vi "Position_TOTAL_R23.vi"(5 "Distance Between \nCameras  (*unit)":sgl=2.3) -> (12 "dX, dY\nLeft Cam":cluster{"X":sgl[], "Y":sgl[]}={"X"=[-1.0065897, 0.099401906, 1.1628555, 2.2500029, 0.0], "Y"=[10.716516, 10.801518, 10.883252, 10.9668045, 0.0]}, 13 "Position Valid":bool=TRUE, 14 "Left Camera Real Coordinates":cluster{"X":sgl, "Y":sgl}={"X"=10.842023, "Y"=1.3735824}, 16 "dX, dY\nRight Cam":cluster{"X":sgl[], "Y":sgl[]}={"X"=[-2.8840373, -1.7780458, -0.7145921, 0.3725553, -1.8774476], "Y"=[9.387911, 9.472914, 9.554648, 9.638201, -1.3286046]}, 18 "Robot Coordinates":cluster{"X":sgl, "Y":sgl}={"X"=10.17772, "Y"=2.3123062}, 19 "Orietnation\n(current)":sgl=-30.94054 format="%#_13g")   [LabVIEW 2015]
uses:
  <vilib>/Analysis/coordinate.llb/2D Cartesian Coordinate Rotation (Array).vi
  <vilib>/myRIO/Common/Instrument Driver Framework/myRIO v1.0/DIO/vis/myRIO v1.0 Close DIO.vi
  <vilib>/myRIO/Common/Instrument Driver Framework/myRIO v1.0/DIO/vis/myRIO v1.0 Unreserve DIO.vi
  <vilib>/myRIO/Common/Instrument Driver Framework/myRIO v1.0/DIO/vis/myRIO v1.0 Build MUX Configuration DIO.vi
  <vilib>/myRIO/Common/Instrument Driver Framework/myRIO v1.0/Resource Manager/vis/myRIO v1.0 Unreserve Channel List.vi
  <vilib>/myRIO/Common/Instrument Driver Framework/myRIO v1.0/Resource Manager/vis/myRIO v1.0 Create Configuration List.vi
  <vilib>/myRIO/Common/Instrument Driver Framework/myRIO v1.0/Resource Manager/vis/myRIO v1.0 Unreserve Channel.vi
  <vilib>/myRIO/Common/Instrument Driver Framework/myRIO v1.0/Resource Manager/vis/myRIO v1.0 Build Mutex Name.vi
  <vilib>/Instr/_visa.llb/VISA Configure Serial Port (Instr).vi
  <vilib>/myRIO/Common/Instrument Driver Framework/myRIO v1.0/DIO/vis/myRIO v1.0 Shutdown DIO.vi
  <vilib>/Utility/error.llb/Error Cluster From Error Code.vi
  <vilib>/myRIO/Common/Instrument Driver Framework/myRIO v1.0/Resource Manager/vis/myRIO v1.0 Configure IO.vi
  <vilib>/myRIO/Common/Instrument Driver Framework/Utilities/vis/Configuration Manager.vi
  <vilib>/myRIO/Common/Instrument Driver Framework/Utilities/vis/IO Manager.vi
  <vilib>/myRIO/Common/Instrument Driver Framework/myRIO v1.0/myRIO v1.0 Close.vi
  <vilib>/Analysis/NI_AALPro.lvlib
  <vilib>/myRIO/Instrument Drivers/Onboard IO/DIO/DIO.lvlib
panel:
  in  "New Orientation\nWeight":sgl=0.2
  out "Array 3":sgl[](array[numeric])=[3.2039287, 3.9103284, 4.8311996, 5.9665127, 6.4357905]
  out "Array 2":sgl[](array[numeric])=[5.5039287, 6.210328, 7.1312, 8.266513, 8.73579]
  out "Array":sgl[](array[numeric])=[9.555056, 8.575206, 8.036942, 7.810829, 6.6351933]
  in  "New Position\nWeight (Y coord)":sgl=0.3 format="%#_13g"
  out "Scale Based\nWeight":sgl=1.0 format="%#_13g"
  in  "Triangle Based\nWeight":sgl format="%#_13g"
  out "Current Cam State - R":T1(ring)=enum."Normal - 5"
  out "Current Cam State - L":T1(ring)=enum."Normal - 5"
  out "Valid Beacon Sets_":bool[](array[boolean])=[TRUE, TRUE, TRUE, TRUE, TRUE]
  in  "Distance Threshold\nRef Triangles (*unit)":sgl=30.0
  out "dA2 4":sgl=48.543114 format="%#_13g"
  out "dA2 2":sgl=48.543114 format="%#_13g"
  out "dA2 3":sgl=44.126 format="%#_13g"
  out "Beacon Scales - Left":sgl[](array[numeric])=[46.59789, 48.180458, 47.842606, 46.504417, 45.297752]
  out "Beacon Scales - Right":sgl[](array[numeric])=[50.81787, 54.150085, 54.01553, 51.723366, 54.605507]
  in  "New Orientation \nThreshold":sgl=20.0
  in  "Moving Average\nWindow Length":u8=10
  out "Current Recovery State -L":enum16{"Generic Sweep", "Recovery Search"}(ring)=enum."Recovery Search"
  out "Current Move Delta - L 2":u16
  out "Next Recovery State - Left":enum16{"Generic Sweep", "Recovery Search"}(ring)=enum."Recovery Search"
  out "Next Recovery State - Right":enum16{"Generic Sweep", "Recovery Search"}(ring)=enum."Recovery Search"
  out "Current Recovery State - Right":enum16{"Generic Sweep", "Recovery Search"}(ring)=enum."Recovery Search"
  in  "Initial Recovery State  - Right":enum16{"Generic Sweep", "Recovery Search"}(ring)=enum."Recovery Search"
  in  "Initial Recovery State - L":enum16{"Generic Sweep", "Recovery Search"}(ring)=enum."Recovery Search"
  out "Next Tracking State - Right":enum16{"Track", "Reactive Predict", ""}(ring)
  out "Current Tracking State - Right 2":enum16{"Track", "Reactive Predict", ""}(ring)
  in  "Initial Tracking State - Right":enum16{"Track", "Reactive Predict", ""}(ring)
  out "Last Track Angle - R":sgl=59.941406
  out "Next Tracking State - Left":enum16{"Track", "Reactive Predict", ""}(ring)
  in  "Initial Tracking State - Left":enum16{"Track", "Reactive Predict", ""}(ring)
  out "Current Tracking State - Left":enum16{"Track", "Reactive Predict", ""}(ring)
  in  "Timeout to \nEnable Reactive Predict":u16=5
  out "Tracking Timeout\nCount - R":i32
  in  "Tracking Timeout\nThreshold":i32=10
  out "Tracking Timeout\nCount - L":i32
  in  "Search Direction - in - Right":bool=TRUE
  out "Next Main State - Right":T2(ring)=enum."Tracking"
  in  "Recovery Search\nDirection - R":bool
  out "Recovery Mode Count in Right":i32
  out "Frames Processed\nCount - in Right":i32
  out "Recovery Search\nmove Count - Right":u16
  out "Recovery Search\nAttempt Count - Right":u16
  in  "Mounting Offset - Right":sgl=45.0
  in  "Tracking Angle - Right":sgl=58.953144
  in  "Current Servo Position\n- Right":u16
  out "New Data  Flag\nRight Servo":bool
  in  "Track Angle Valid  - Right":bool=TRUE
  out "Current Main State - Right":T2(ring)=enum."Tracking"
  in  "Initial Main State- Right":T2(ring)
  in  "Recovery Search\nDirection - L 2":bool
  in  "Max Recovery Count\n(Recovery Search) 2":u16
  in  "Max Recovery\nSearch Attempts 2":u16
  in  "Image Lock - Right 2":bool
  out "Last Track Angle - L":sgl=52.96875
  in  "Recovery Search\nDirection - L":bool=TRUE
  out "Next Main State - Left":T2(ring)=enum."Tracking"
  out "Current Move Delta - L":u16
  in  "Max Recovery Count\n(Recovery Search)":u16=10
  in  "Max Recovery\nSearch Attempts":u16=3
  out "Recovery Search\nAttempt Count - in - L":u16
  out "Recovery Search\nmove Count - in - L":u16
  in  "Image Lock - Right":bool=TRUE
  out "Recovery Mode Count - in Left":u16
  in  "Middle Beacon\nCoordinates":cluster{"X":sgl, "Y":sgl}={"X"=0.0, "Y"=2.5}
  in  "Min Num Frames\nper Search":i32=5
  in  "Wait Tick Threshold":i32=10
  out "Frames Processed\nCount - in -L":i32
  in  "Maximum Move \nServo Threshold":i16=300
  in  "Minimum Delta \nServo Threshold":i16=3
  in  "Mounting Offset - Left":sgl=-45.0
  in  "Search Step Size":u16=50
  in  "Search Direction - in - L":bool
  in  "Current Servo Position\n- Left":u16
  in  "Tracking Angle - Left":sgl=52.933372
  out "New Data  Flag\nLeft Servo":bool
  in  "Track Angle Valid - Left":bool=TRUE
  in  "Image Lock - Left":bool=TRUE
  in  "Initial Main State - Left":T2(ring)
  out "Current Main State - Left":T2(ring)=enum."Tracking"
  in  "Position Calc\nTimer":u32=100 caption="Position Calc Timer"
  in  "Fetch Input\n(mSec)":u32=20 caption="Update Camera Input\n(mSec)"
  out "Right Data\nInput Flag\n- Internal":bool
  in  "Position Calc\nReady":bool=TRUE
  out "This Servo \nAngle - Right":sgl=58.76953
  in  "Beacon Angles -R":sgl[](array[numeric])=[71.43643, 65.46979, 58.9926, 52.62266, 45.904842]
  in  "Beacon Angles - L":sgl[](array[numeric])=[64.19745, 58.642975, 52.682835, 47.05908, 41.446476]
  in  "Valid Angles -R":bool[](array[boolean])=[TRUE, TRUE, TRUE, TRUE, TRUE]
  in  "Valid Angles - L":bool[](array[boolean])=[TRUE, TRUE, TRUE, TRUE, TRUE]
  out "Left Data\nInput Flag\n- Internal":bool
  in  "Check Shared Var Timer":u32=50 caption="Main Loop\n Timer (ms)"
  out "Left_Flag 2":bool
  out "Right_Flag 2":bool
  out "Beacons Found\n- Left (Bool Array) 2":bool[](array[boolean])=[TRUE, TRUE, TRUE, TRUE, TRUE]
  out "LEFT Beacon Coord - X px (IN) 2":sgl[](array[numeric])=[96.57839, 127.0317, 159.93825, 190.94315, 221.86247]
  out "LEFT Beacon Position - Y px (IN) 2":sgl[](array[numeric])=[111.67795, 107.306076, 106.92789, 105.73433, 104.09002]
  out "This Servo \nAngle - Left":sgl=52.96875
  in  "Compliance Slope":u8=128
  out "deltaMoveServo\n- R":i16
  out "Move Respond - R":bool
  out "Move Respond - L":bool
  out "Last Position":cluster{"X":sgl, "Y":sgl}={"X"=10.147585, "Y"=2.64441}
  out "Last Orientation":sgl=-35.285717
  in  "Distance\nBetween Beacons \n- Tolerance":sgl=0.5 format="%#_13g"
  in  "Distance\nBetween Beacons":sgl=1.0 format="%#_13g"
  out "dT":dbl=144.111
  out "Position Valid\nHistory":bool[](array[boolean])=[TRUE, TRUE, TRUE, TRUE, FALSE, TRUE, TRUE, TRUE, TRUE, TRUE, TRUE, TRUE, TRUE, TRUE, TRUE]
  out "Orientation\nHistory":sgl[](array[numeric])=[-35.285717, -36.86449, -36.153664, -35.44657, 0.0, -37.6105, -36.02637, -35.82032, -36.08894, -37.01076, -36.293255, -36.40525, -35.738438, -35.683483, -35.770218]
  out "Robot Coordinates\nHistory":cluster{sgl, sgl}[](array[cluster])=[{10.147585, 2.64441}, {10.056327, 2.8351064}, {10.020484, 2.7815769}, {10.034186, 2.7172103}, {0.0, 0.0}, {10.036168, 2.7859242}, {9.938812, 2.8961887}, {10.1160965, 2.6632404}, {10.016709, 2.7454932}, {10.037537, 2.8544023}, {10.017025, 2.7817721}, {9.997087, 2.8064857}, {10.065648, 2.6537364}, {10.084976, 2.6750228}, {10.082739, 2.688601}]
  in  "New Position \nThreshold":sgl=2.0
  out "Orientation Avgd":sgl=-35.285717
  in  "History Size":u8=15
  in  "Max Y (arena)":sgl=15.0
  in  "Max X (arena)":sgl=35.0
  in  "New Position\nWeight (X coord)":sgl=0.8 format="%#_13g"
  in  "Max Std Dev (3)":sgl=0.2 format="%#_13g"
  in  "Max Std Dev (4)":sgl=0.1 format="%#_13g"
  out "Post Filtering\n- Valid Beacons":bool[](array[boolean])=[TRUE, TRUE, TRUE, TRUE, FALSE]
  out "Robot Coordinates - Avgd":cluster{"X":sgl, "Y":sgl}={"X"=10.147585, "Y"=2.64441}
  out "Real Position in Course 2":cluster{"X":dbl[], "Y":dbl[]}(graph)={"X"=[10.147584990557128], "Y"=[2.644409845240164]}
  out "Position \nLock Status":bool=TRUE
  out "Right Camera Real Coordinate":cluster{"X":sgl, "Y":sgl}={"X"=9.513418, "Y"=3.25103}
  out "deltaMoveServo\n- L":i16
  in  "Search Step Size\n(deg)":sgl=15.0 format="%#_13g"
  out "Beacons Found\n- Right (Bool Array)":bool[](array[boolean])=[TRUE, TRUE, TRUE, TRUE, TRUE]
  out "RIGHT Beacon Position - Y px (IN)":sgl[](array[numeric])=[106.21975, 102.49595, 103.61968, 103.22959, 103.920715]
  out "RIGHT Beacon Coord - X px (IN)":sgl[](array[numeric])=[88.975365, 121.85722, 157.60713, 192.74931, 229.82234]
  in  "Right Servo\nID":string="\u0001"
  in  "Servo Comm\nWait Time - (ms)":i32
  in  "Left Servo\nID":string="\u0000"
  out "dT - Comm Loop":u32=21
  in  "Servo Comm\nLoop Time (ms)":i32=20
  in  "close comms":bool
  in  "Max Read\nTx Attempts":u8=3
  in  "Max Write\nTx Attempts":u8=3
  out "Current R (10bit)":u16=559
  out "Servo Moving - R":bool
  out "Servo Moving - L":bool
  out "Current L (10bit)":u16=232
  in  "SERVO ENABLE":bool=TRUE
  out "Move Servo - L":bool
  out "Move Servo - R":bool
  in  "Servo Goal Position\n - Right":u16=563
  in  "Move Servo\nThreshold (deg)":sgl=2.0 format="%#_13g"
  in  "Servo Algorithm\nCycle Time(ms)":i32=25
  in  "Servo Goal Position\n - Left":u16=232
  in  "Current Angle\n - Left (internal)":sgl=52.96875
  in  "Current Angle\n - Right (internal)":sgl=58.76953
  in  "stop":bool
  in  "Num of Beacons (Total)":i8=5
  out "Angle to Pixel Ratios":T3={"Angle to Pixel\nRatio - Horizontal"=0.18125, "Angle to Pixel\nRatio - Vertical"=0.1875} {"Angle to Pixel\nRatio - Vertical" format="%#_13g"; "Angle to Pixel\nRatio - Horizontal" format="%#_13g"}
  in  "Cam AOV Vertical (deg)":sgl=45.0
  in  "Cam AOV Horizontal (deg)":sgl=58.0
  in  "Image Height (px)":sgl=240.0
  in  "Image Width (px)":sgl=320.0
  out "Beacon Coordinates - Left Image":T4={"Beacon Position - X px"=[96.57839, 127.0317, 159.93825, 190.94315, 221.86247], "Beacon Position - Y px"=[111.67795, 107.306076, 106.92789, 105.73433, 104.09002]}
  out "Beacon Coordinates - Right Image":T4={"Beacon Position - X px"=[88.975365, 121.85722, 157.60713, 192.74931, 229.82234], "Beacon Position - Y px"=[106.21975, 102.49595, 103.61968, 103.22959, 103.920715]}
  out "Distance to LBF":sgl[](array[numeric])=[0.024284193, 0.015691843, 0.008273765, 0.028971607, 0.03291407]
  out "Local Coordinates - Calculated":cluster{sgl[], sgl[]}(graph)={[5.5039287, 6.210328, 7.1312, 8.266513, 8.73579], [9.555056, 8.575206, 8.036942, 7.810829, 6.6351933]}
  out "Local Coordinates - Rotated":cluster{dbl[], dbl[]}(graph)={[1.8774476489648846, -1.0065896210507148, 0.09940190570174412, 1.1628555490135675, 2.250002943734801, 0.0], [1.3286045709883498, 10.716515276262749, 10.801518262128845, 10.883252530212562, 10.966804865321656, 0.0]}
  out "All Object Coordinates \n- Local - Rotated":cluster{"X":sgl[], "Y":sgl[]}={"X"=[1.8774476, -1.0065897, 0.099401906, 1.1628555, 2.2500029, 0.0], "Y"=[1.3286046, 10.716516, 10.801518, 10.883252, 10.9668045, 0.0]}
  out "Local Coordinates - Normalized":cluster{sgl[], dbl[]}(graph)={[2.3, 5.368779, 6.320682, 7.235974, 8.171657, 0.0], [0.0, 9.329154968261719, 8.759660720825195, 8.21207046508789, 7.65227746963501, 0.0]}
  in  "Max Std Dev (5)":sgl=0.1 format="%#_13g"
  out "All Object Coordinates \n- Local":cluster{"X":sgl[], "Y":sgl[]}={"X"=[2.3, 5.368779, 6.320682, 7.235974, 8.171657, 0.0], "Y"=[0.0, 9.329155, 8.759661, 8.21207, 7.6522775, 0.0]}
  out "LOCAL\nBeacon Coordinates\nRelative to Robot":cluster{"dX_beacon":sgl[], "dY_beacon":sgl[]}={"dX_beacon"=[5.5039287, 6.210328, 7.1312, 8.266513, 8.73579], "dY_beacon"=[9.555056, 8.575206, 8.036942, 7.810829, 6.6351933]}
  in  "Real Beacon\n - Coordinates":cluster{"X":dbl[], "Y":dbl[]}={"X"=[0.0, 0.0, 0.0, 0.0, 0.0, 0.0], "Y"=[0.5, 1.5, 2.5, 3.5, 4.5, 0.0]}
  # "POSITION CALCULATION VARIABLES"
  # "OUTPUT VALUES"
  # "CONFIG VALUES"
  # "FILTER CONFIG VALUES"
  # "FEEDBACK INPUT VALUES"
  # "INPUT VALUES"
  # "INTERMEDIATE VALUES"
  # "IMAGE TO ANGLE VARIABLES"
  # "update to coordinate outlier filtering R2"
  # "VISION PROCESSEING INPUTS"
  # "Use moving average for previous orientation thresholds"
  # "INPUTS"
  # "CONFIG"
  # "OUTPUT VALUES"
  # "*********************"
  # "unfiltered"
  # "NEW FILTER VALS"
  # "Inter Beacon Distance Filtering"
  # "MOVING AVERAGE\nVARIABLES"
  # "DISTANCE SOURCE WEIGHT"
  # "*****  I made this 0\n         bc it seems to be \n        more stable"
  # "SERVO CONTROL VARIABLES"
  # "SERVO CONTROL VARIABLES"
  # "CONFIG"
  # "SHARED VARIABLE INPUTS"
  # "LOCAL VARIABLE INPUTS"
  # "INTERNRAL VARIABLES"
  # "SEARCH ROUTINE VARIABLES"
  # "MISC"
  # "SERVO IDs"
  # "CONTROL DELAYS"
  # "COMM LOOP DELAY"
  # "COMM PROTOCOL"
  # "SETTINGS"
  # "Make function of distance^^"
  # "**** only left side starts search\nat previously known good angle"
  # "LEFT SERVO"
  # "RIGHT SERVO"
  # "Main State Machine"
  # "Recovery State Machine"
  # "Current Track Angle Inputs"
  # "Servo Status Inputs"
  # "Main State Machine Inputs"
  # "Recovery State Machine Inputs"
  # "Current Track Angle Inputs"
  # "Servo Status Inputs"
  # "Recovery State Machine Feedback"
  # "Tracking State Machine Inputs"
  # "Tracking State Machine Inputs"
  # "NOTE: Must be 1 bigger than amount of beacons"
  # "NOTE: Must be 1 bigger than amount of beacons"
types:
  T1 = enum16{"Sub - 2", "Sub - 3", "Sub - 4", "Normal - 5"}
  T2 = enum16{"Start Up Search", "Tracking", "Recovery Mode", ""}
  T3 = cluster{"Angle to Pixel\nRatio - Horizontal":sgl, "Angle to Pixel\nRatio - Vertical":sgl}
  T4 = cluster{"Beacon Position - X px":sgl[], "Beacon Position - Y px":sgl[]}
  T5 = cluster{"Tracking Coordinates":cluster{"X":dbl, "Y":dbl}, "Current Valid":bool, "Current State - Out":enum16{"Sub - 2", "Sub - 3", "Sub - 4", "Normal - 5"}, "Setting Values":cluster{"Min Scale":dbl, "Max Scale":dbl, "Min Score":dbl}}
  T6 = cluster{"Array of Double":dbl[], "Array of Double":dbl[]}
  T7 = typedef "DIO.lvlib/DIO Reference.ctl" = cluster{"myRIO Reference":T8, "DIO Channels List":T12}
  T8 = typedef "myRIO Generic Hardware Reference.ctl" = cluster{"myRIO Model":T9, "myRIO Hardware Reference":T10}
  T9 = typedef "Hardware Version Enum.ctl" = enum16{"Unknown", "myRIO-1900", "myRIO-1950", "roboRIO"}
  T10 = typedef "myRIO v1.0 Reference.ctl" = cluster{"Generic FPGA Reference":T11, "Allow multiple opens":bool}
  T11 = typedef "Generic FPGA Reference.ctl" = refnum<k20>
  T12 = typedef "DIO Channels List.ctl" = T13[]
  T13 = typedef "DIO Channels Enum.ctl" = enum16{"Not Connected", "C/DIO0", "C/DIO1", "C/DIO2", "C/DIO3", "C/DIO4", "C/DIO5", "C/DIO6", "C/DIO7", "A/DIO0", "A/DIO1", "A/DIO2", "A/DIO3", "A/DIO4", "A/DIO5", "A/DIO6", "A/DIO7", "A/DIO8", "A/DIO9", "A/DIO10", "A/DIO11", "A/DIO12", "A/DIO13", "A/DIO14", "A/DIO15", "B/DIO0", "B/DIO1", "B/DIO2", "B/DIO3", "B/DIO4", "B/DIO5", "B/DIO6", "B/DIO7", "B/DIO8", "B/DIO9", "B/DIO10", "B/DIO11", "B/DIO12", "B/DIO13", "B/DIO14", "B/DIO15", "LED0", "LED1", "LED2", "LED3", "Button0", "DIO/DIO0", "DIO/DIO1", "DIO/DIO2", "DIO/DIO3", "DIO/DIO4", "DIO/DIO5", "DIO/DIO6", "DIO/DIO7", "DIO/DIO8", "DIO/DIO9", "SPI/CS0", "SPI/CS1", "SPI/CS2", "SPI/CS3", "LED RADIO (Green)", "LED RADIO (Red)", "LED COMM (Green)", "LED COMM (Red)", "LED MODE (Green)", "LED MODE (Red)"}
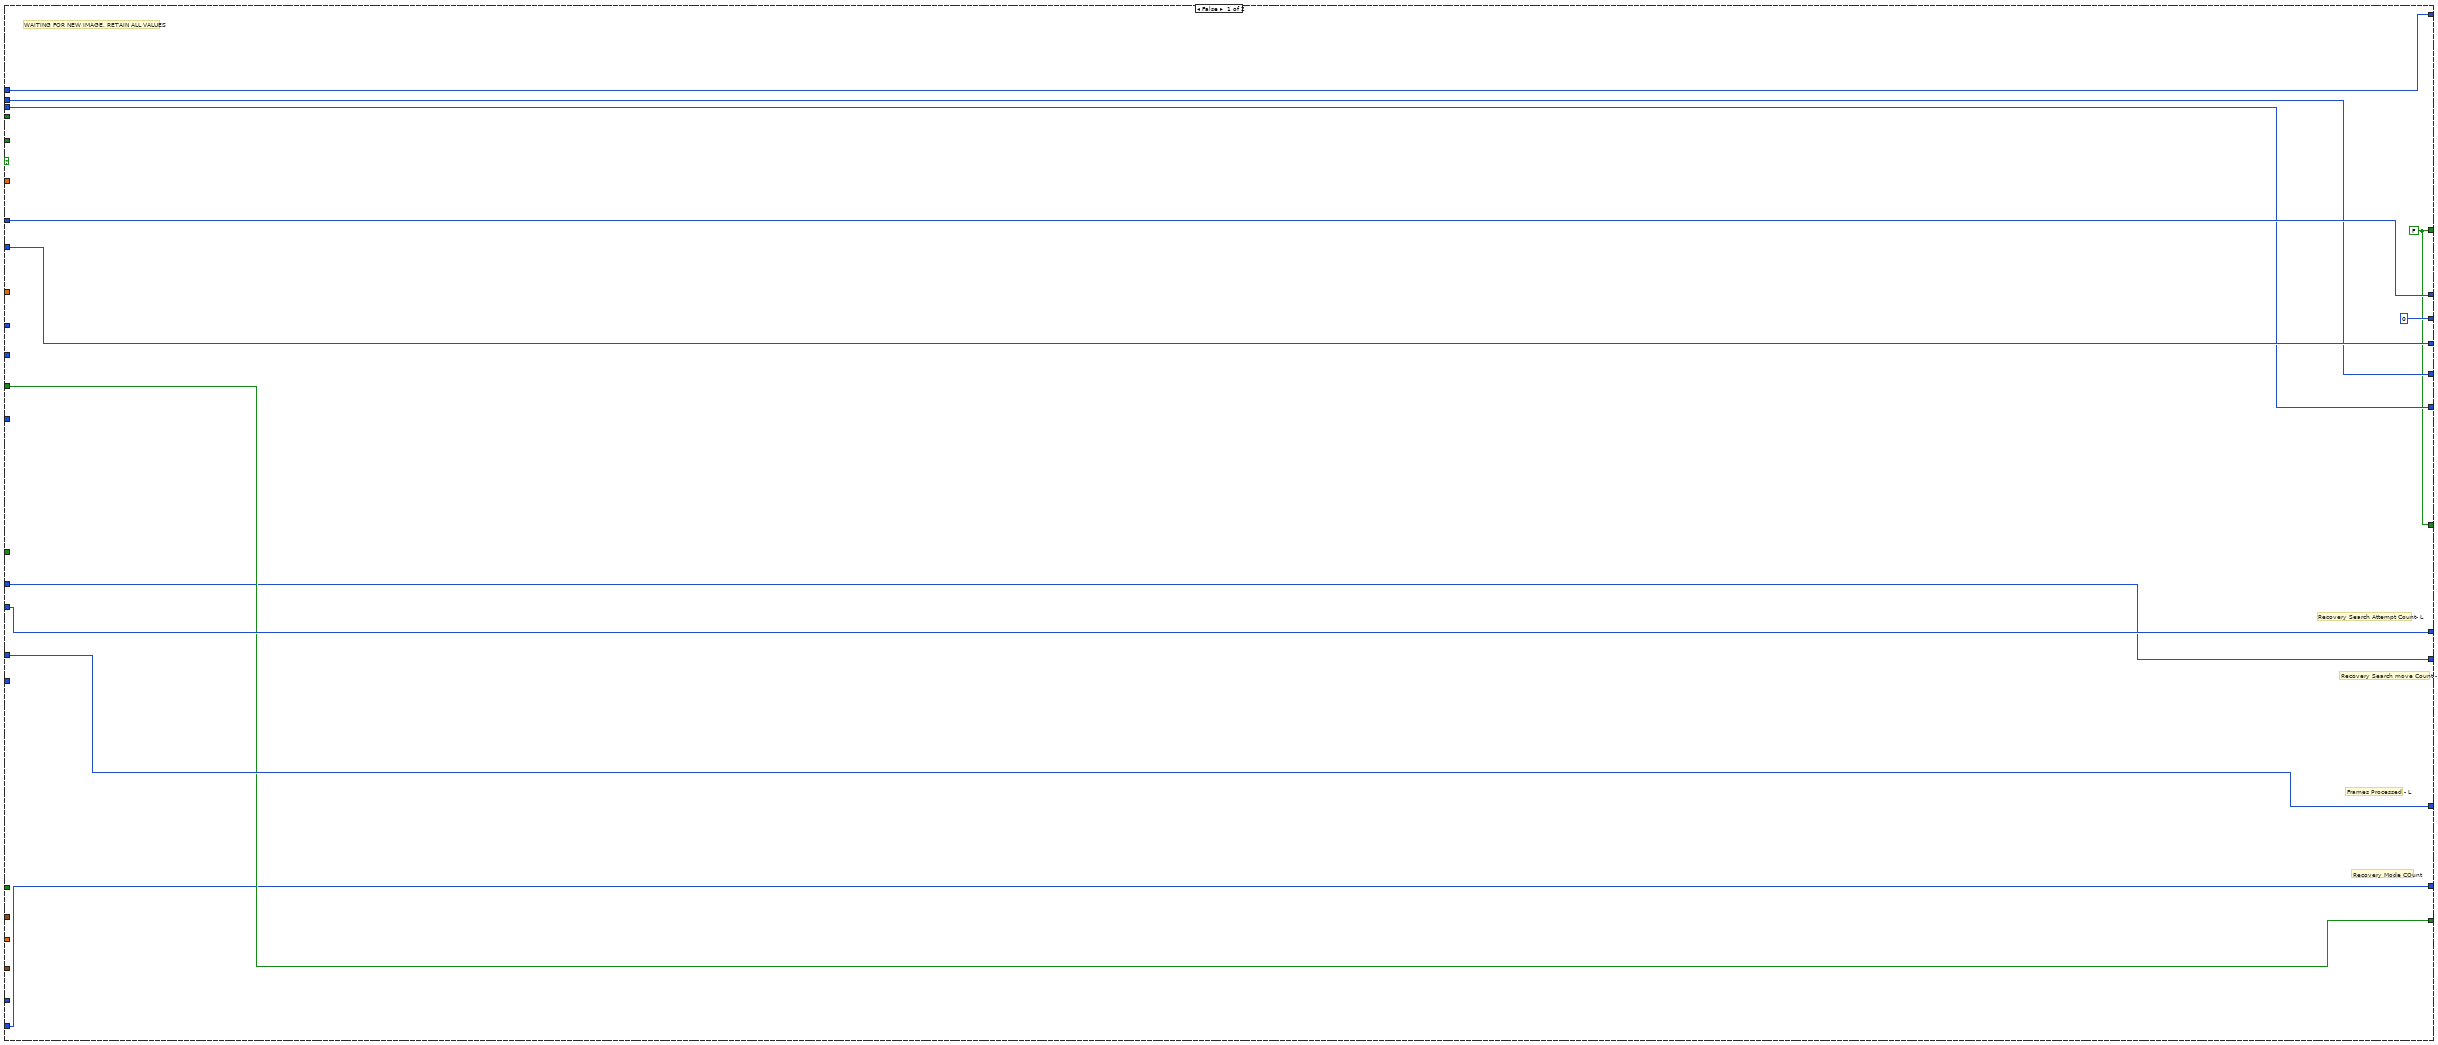
[diagram p2: hidden frame]
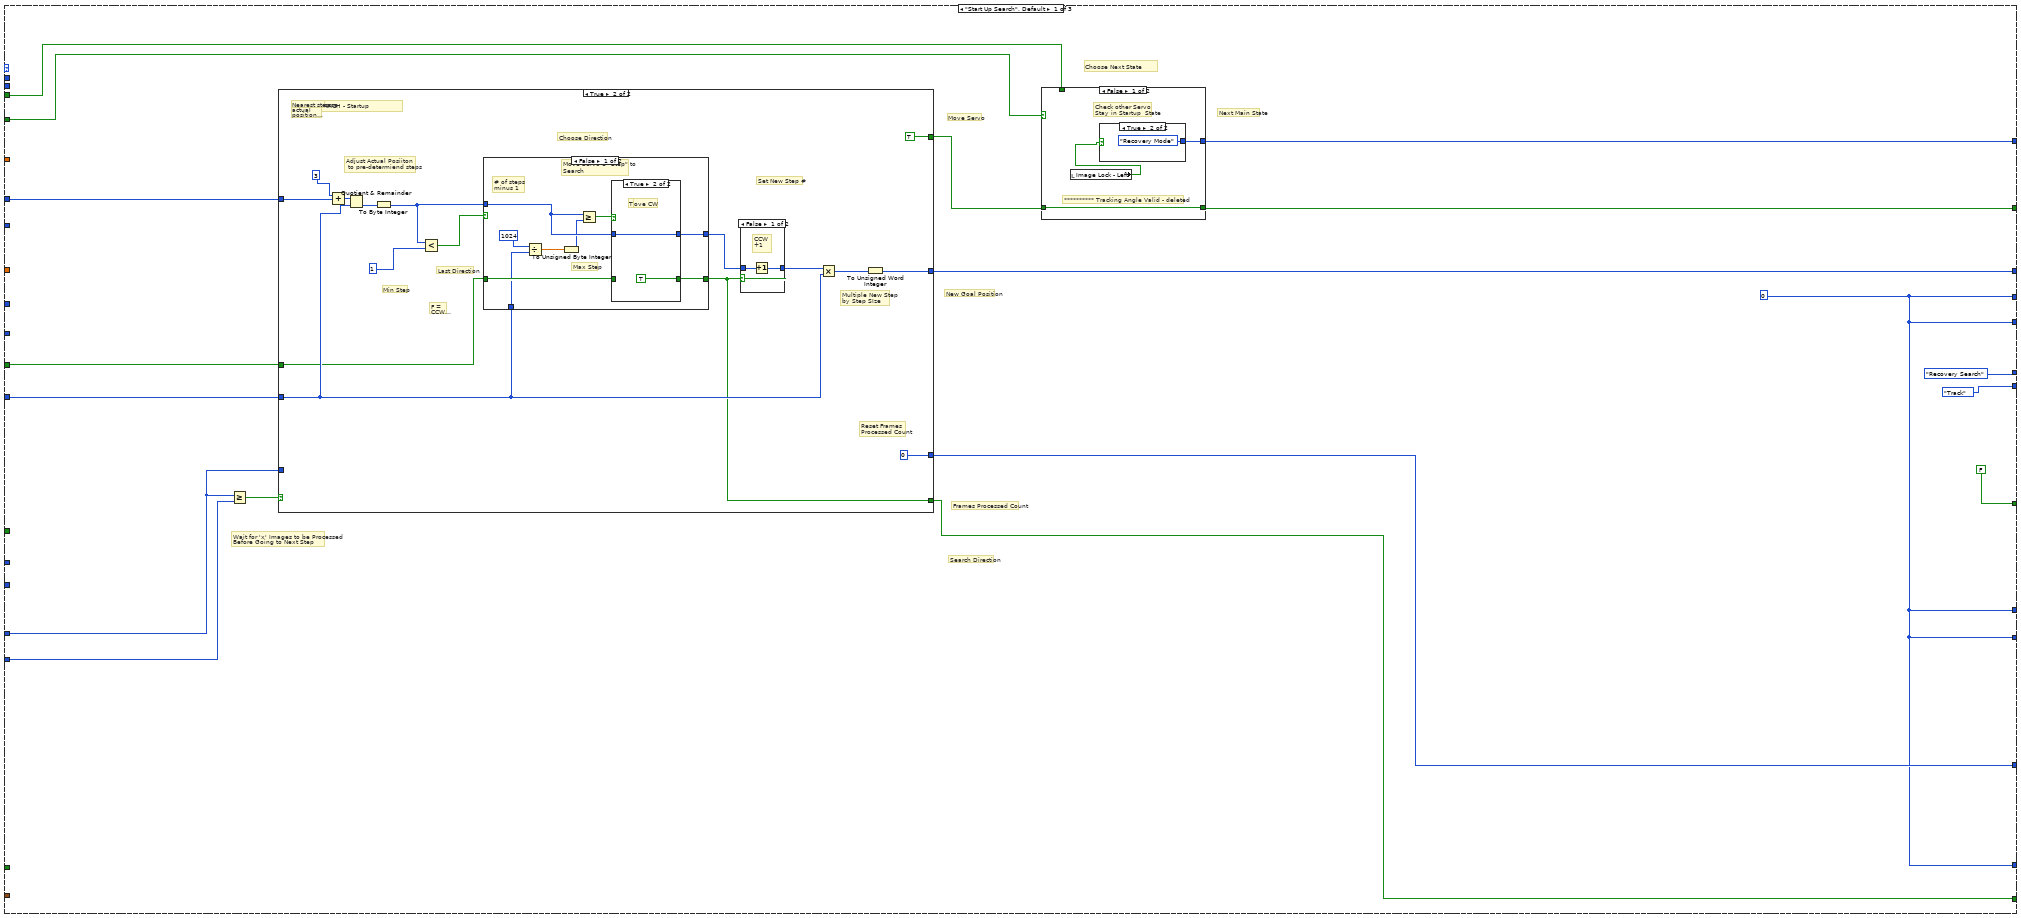
[diagram p3: hidden frame]
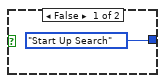
[diagram p4: hidden frame]
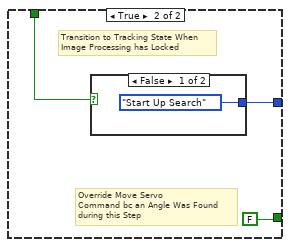
[diagram p5: hidden frame]
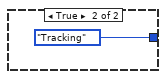
[diagram p6: hidden frame]
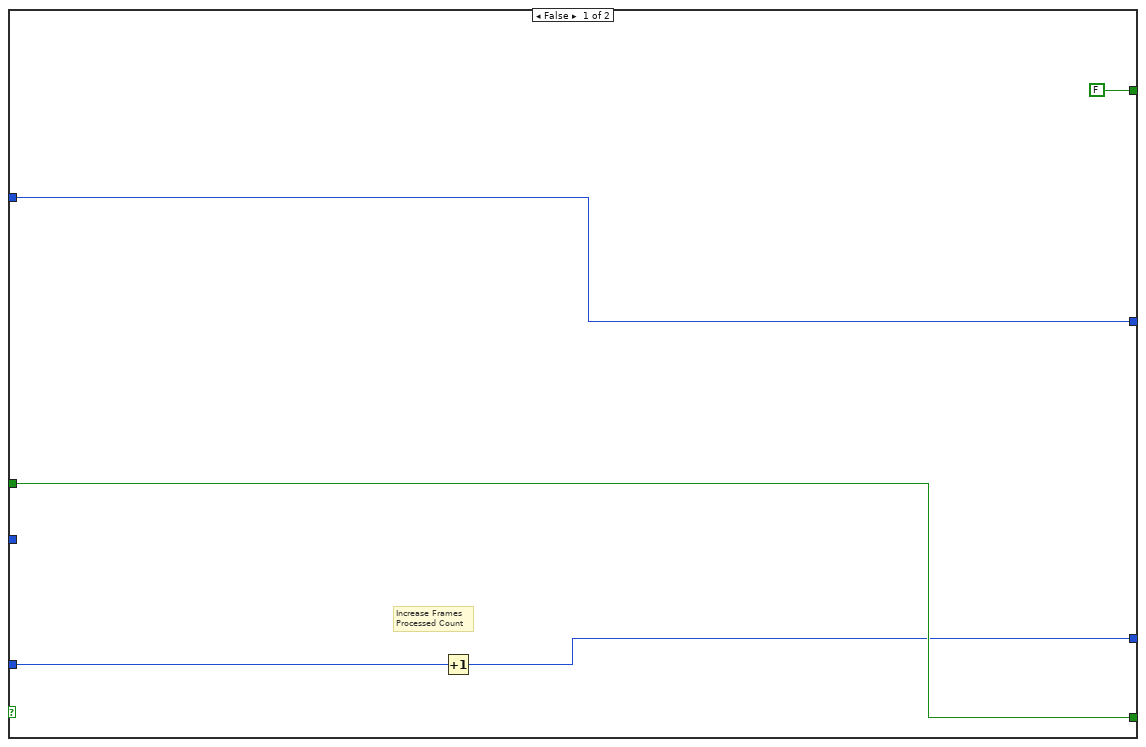
[diagram p7: hidden frame]
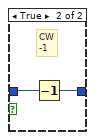
[diagram p8: hidden frame]
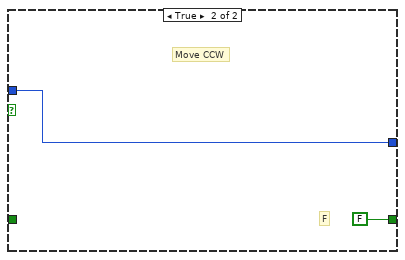
[diagram p10: hidden frame]
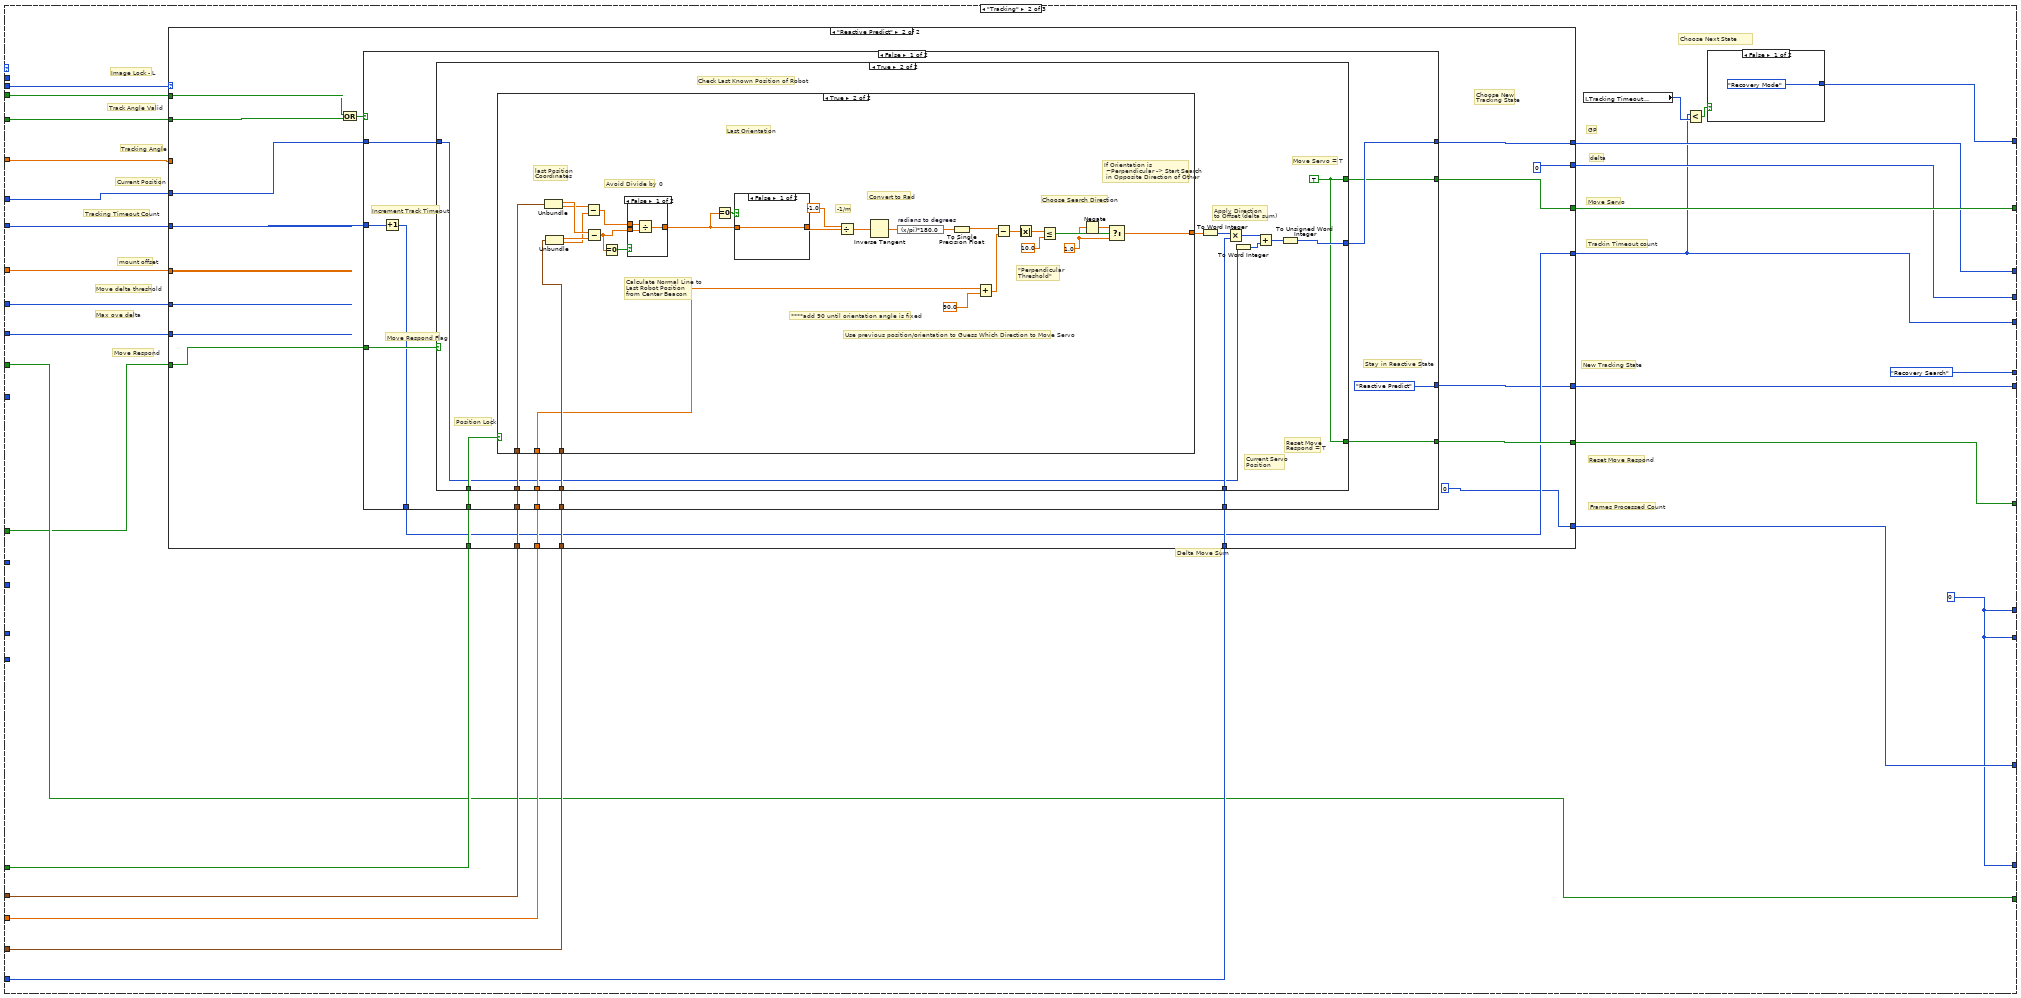
[diagram p11: hidden frame]
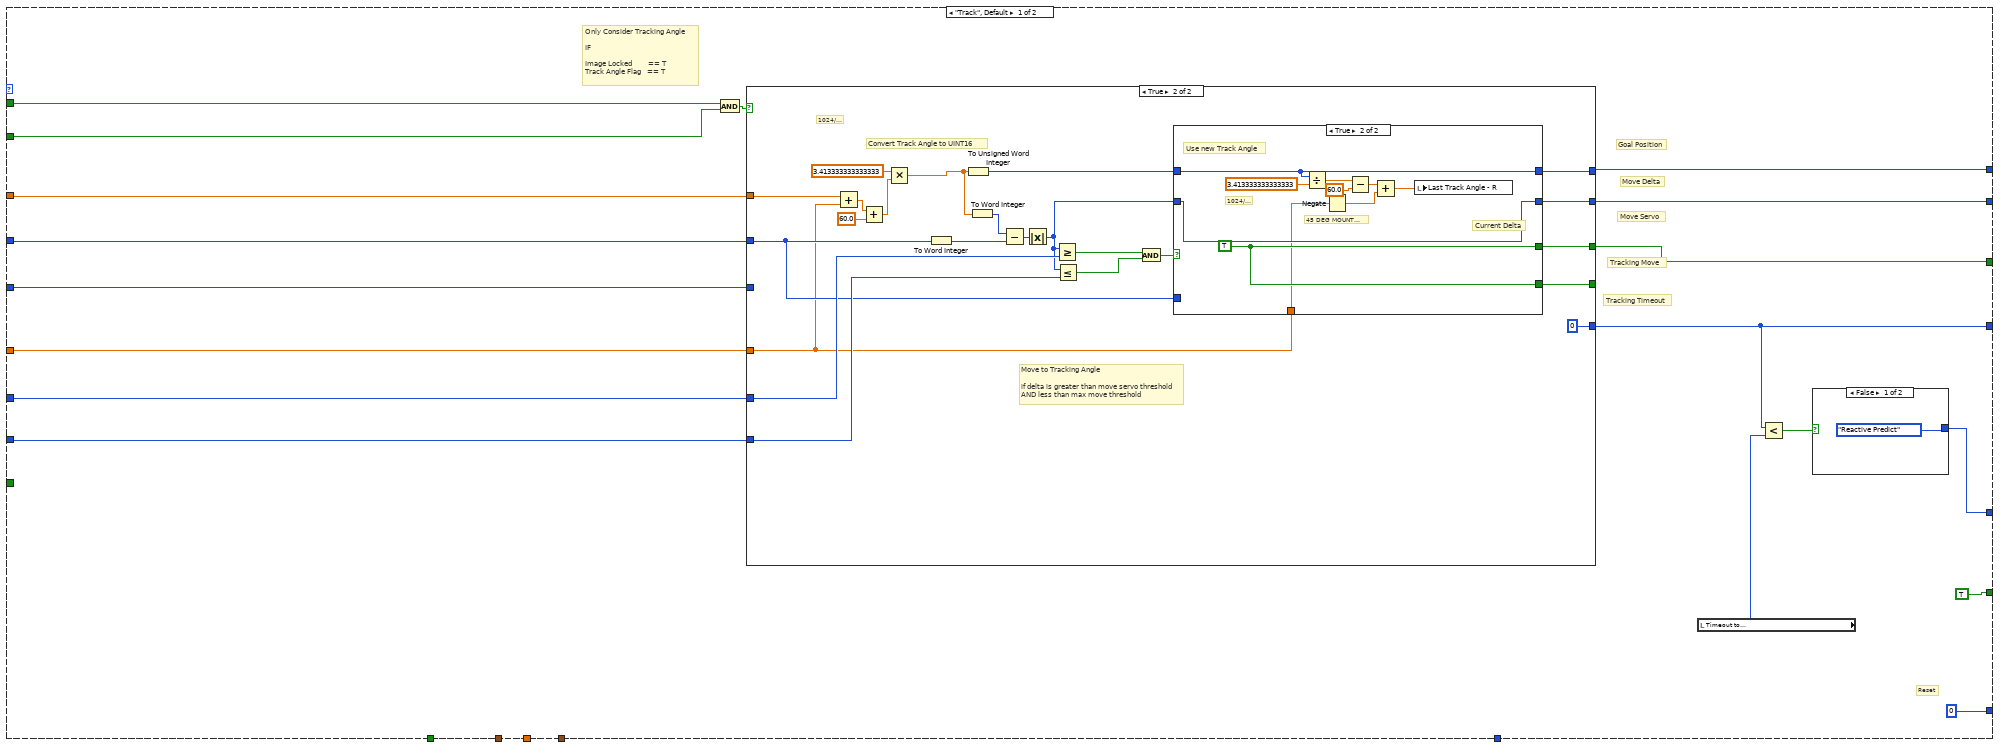
[diagram p12: hidden frame]
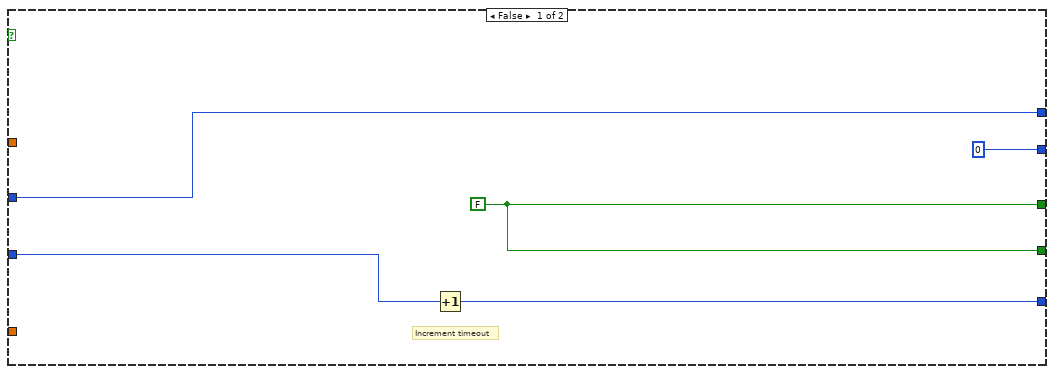
[diagram p13: hidden frame]
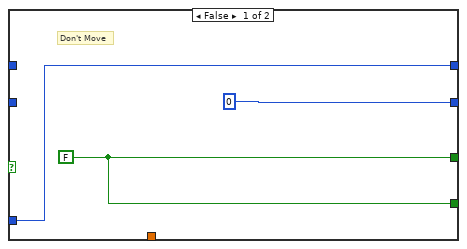
[diagram p14: hidden frame]
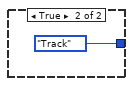
[diagram p15: hidden frame]
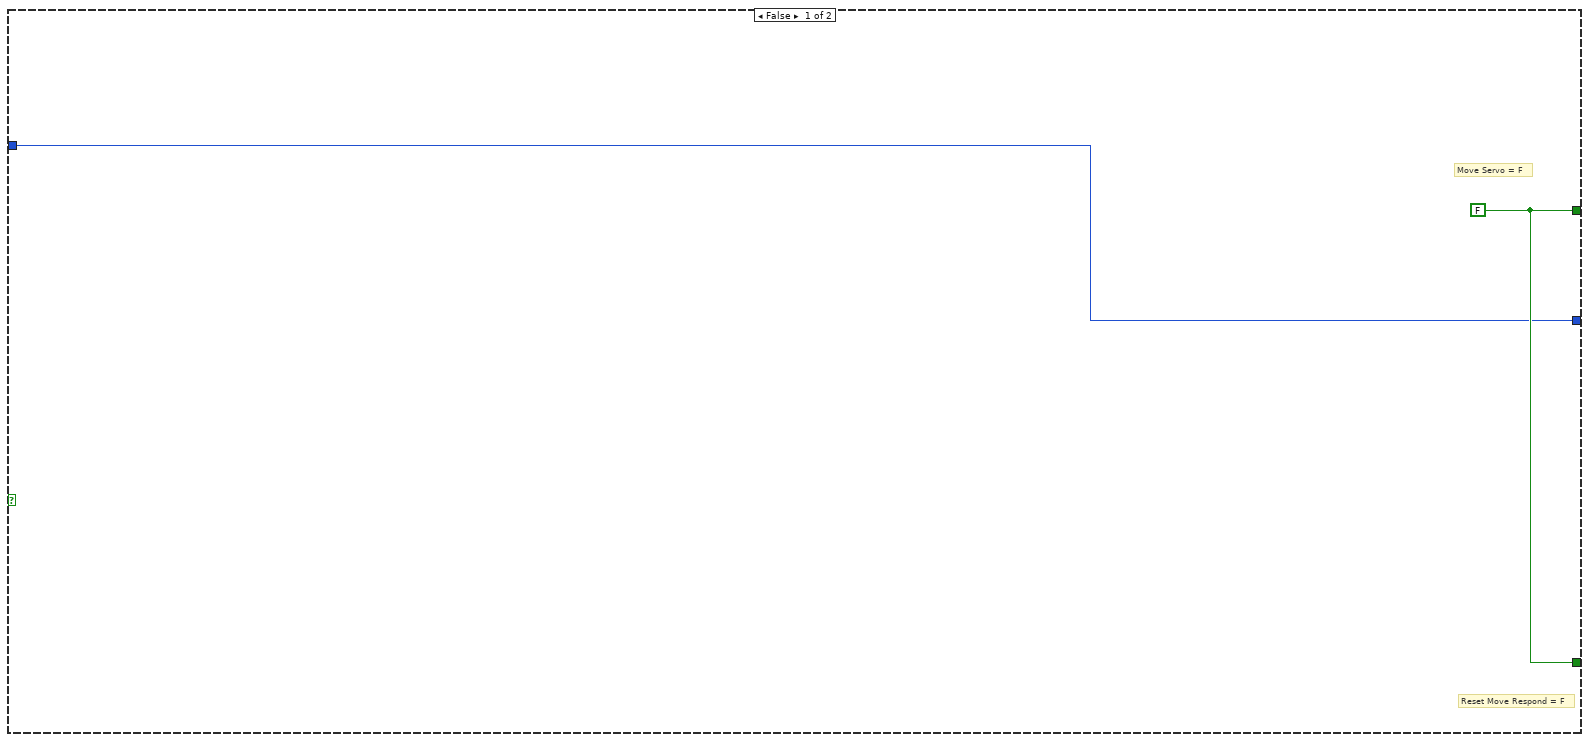
[diagram p16: hidden frame]
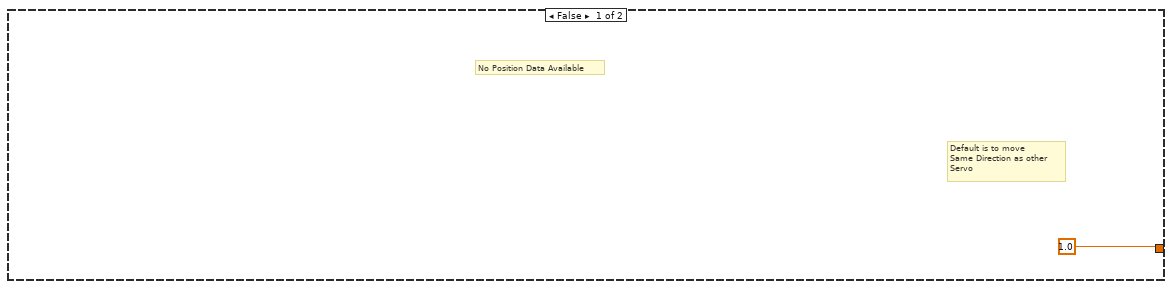
[diagram p17: hidden frame]
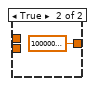
[diagram p18: hidden frame]
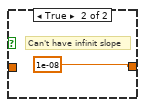
[diagram p19: hidden frame]
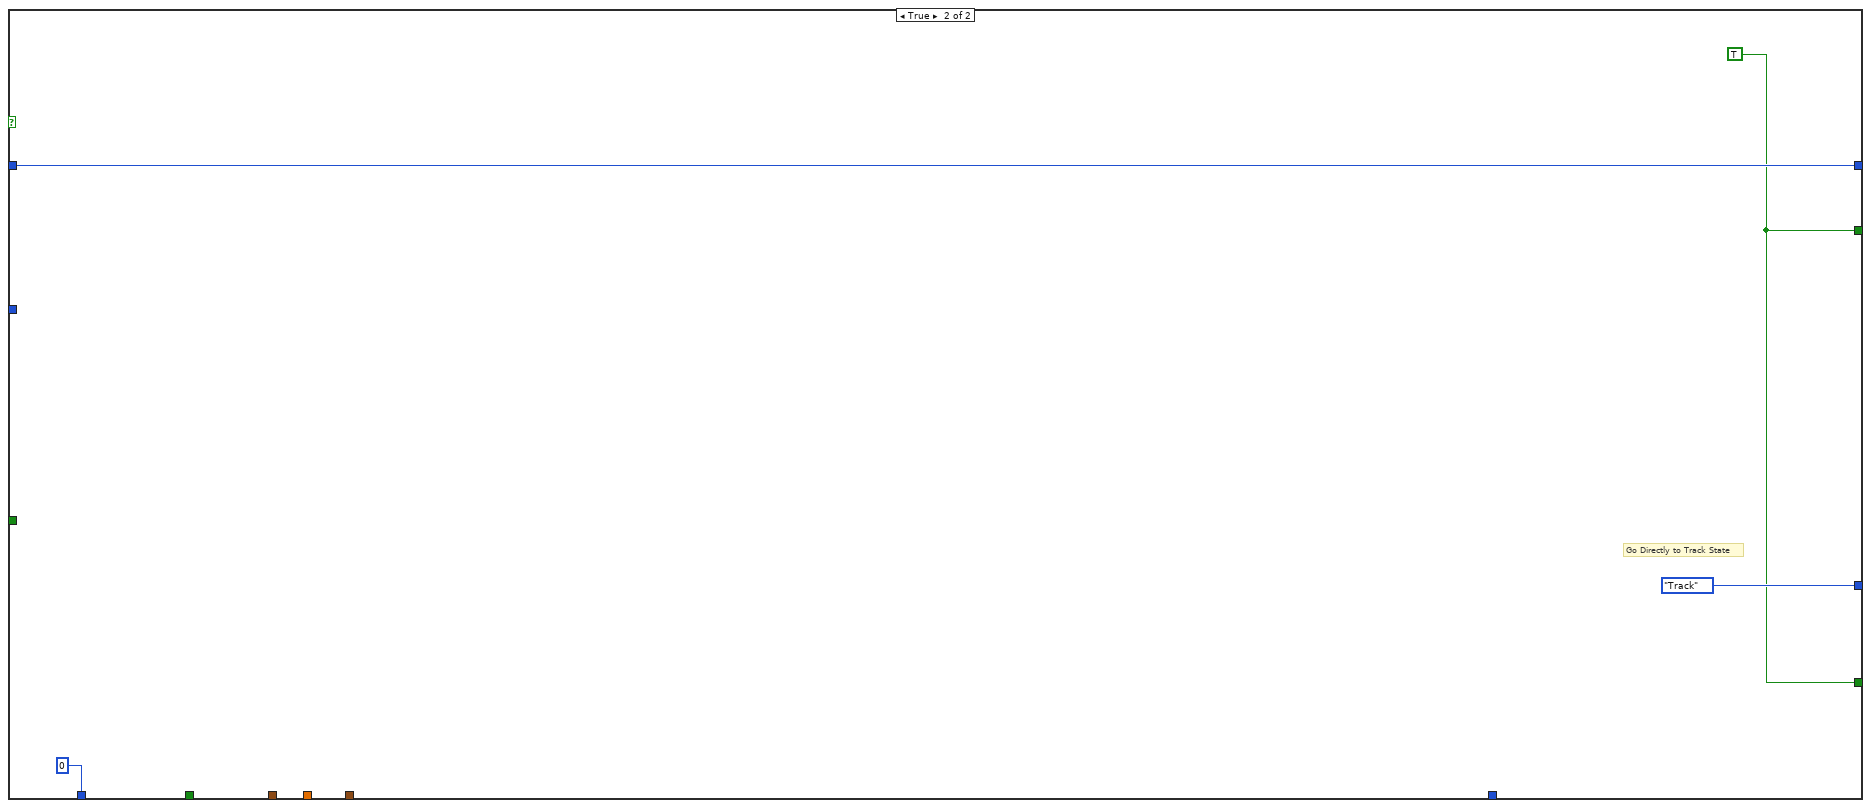
[diagram p20: hidden frame]
diagram:
  (unwired) enum16{"Generic Sweep", "Recovery Search"}."Recovery Search"
  w12 = 0 ("Frames Processed\nCount - in")
  w13 = 0 ("Frames Processed\nCount - in")
  w2 = FALSE
  w34 = sgl 0.0
  # "SERVO CONTROL FLAGS"
  # "***"
  # "Next Tracking State"
  # "Tracking Timeout Count"
  # "Search Direction - L"
  # "Next Recovery State"
  # "Move Respond"
  # "Recovery Mode Count - L"
  # "Delta Move Sum - L"
  # "Wait Tick Count - L"
  # "Frames Processed - L"
  # "Recovery Search move Count - L"
  # "Recovery Search Attempt Count- L"
  # "Next Main State"
  # "Search Direction - L"
  # "Next Recovery State"
  # "INPUTS - Local vars"
  # "Recovery Mode Count - L"
  # "Delta Move Sum - L"
  # "Frames Processed\nLeft"
  # "Move Respond - R"
  # "Initial Search Direction\n- Right"
  # "Move Respond"
  # "Recovery Mode Count - L"
  # "Delta Move Sum - L"
  # "Wait Tick Count - L"
  # "Frames Processed - L"
  # "Recovery Search move Count - L"
  # "Recovery Search Attempt Count- L"
  # "Next Main State"
  # "Settings -- Update in a slow loop"
  # "Recovery Mode Count - L"
  # "Delta Move Sum - L"
  # "Frames Processed\nLeft"
  # "Move Respond - L"
  # "Replace these with\nconstants"
  # "Initial Search Direction\n- Left"
  # "Read Inputs when Available"
  # "# of Physical Beacons"
  # "Right Data Internal Falg"
  # "Left Data Internal Falg"
  # "Initialize Shift Arrays"
  # "Robot Position (cluster)\nShift Array"
  # "Robot Position (cluster)\nShift Array"
  # "Position Valid Shift Array"
  # "Orientation Shift Array"
  # "Position Valid Shift Array"
  # "Orientation Shift Array"
  # "Servo Communication (to Servo- UART))"
  # "Internal Local Variables"
  # "Servo Control Logic"
  # "Local Variables"
  # "Images to Robot Position Calculation Process"
  # "SERVO MOTOR CONTROL"
  # "SERVO MOTOR CONTROL"
  n1 = Divide(x="Cam AOV Horizontal (deg)", y="Image Width (px)") -> (x/y=w25:sgl)
  n2 = Divide(x="Cam AOV Vertical (deg)", y="Image Height (px)") -> (x/y=w26:sgl)
  n3 = Bundle(w25, w26) -> (w20:cluster{sgl, sgl})  [unwired: 1 in]
  "Angle to Pixel Ratios" <- w20
  n4 = disable-structure shown="Disabled" {
    frame Disabled {
      # "Always Read Incoming Flags & Store"
      n5 = while {
        tunnel: "Check Shared Var Timer" -> [w46]
        stop <- FALSE stop-if-true
        n6 = shared-variable "myRIO-1900\\Lib1.lvlib\\RIGHT_FLAG"() -> (→"Right_Flag 2":bool)  [unwired: 1 in, 1 out]
        n7 = shared-variable "myRIO-1900\\Lib1.lvlib\\Left_Flag"() -> (→"Left_Flag 2":bool)  [unwired: 1 in, 1 out]
        n8 = call "Wait8"("Count(mSec)"=w46) -> ()  [unwired: 1 out]
      }
    }
    frame Enabled {
    }
  }
  n9 = while {
    shift-right: [w55] -> _
    shift-left: w2 -> [w60]
    shift-right: [w54] -> _
    shift-left: w2 -> [w58]
    tunnel: w20 -> [w56]
    tunnel: "Num of Beacons (Total)" -> [w57]
    stop <- FALSE stop-if-true
    # "Wait for Both Internal Flags"
    n10 = call "Wait6"("Count(mSec)"="Fetch Input\n(mSec)") -> ()  [unwired: 1 out]
    n11 = shared-variable "RT myRIO Target - Overlord\\Localization_Variables_r0.lvlib\\RIGHT_FLAG"() -> (w51:bool)  [unwired: 1 in, 1 out]
    n12 = shared-variable "RT myRIO Target - Overlord\\Localization_Variables_r0.lvlib\\Left_Flag"() -> (w52:bool)  [unwired: 1 in, 1 out]
    n13 = case shown="True" w51 {
      tunnel: w57 -> [_ w79]
      tunnel: w56 -> [_ w77]
      tunnel: [w61 w67] -> w49
      tunnel: w58 -> [w61 _]
      frame False {
        # "Don't Update Servo Position\nbc we're waiting on new Data to\ncome in and the servo position\nwas set at the previous set of data"
      }
      frame True {
        w67 = TRUE
        # "Store Values"
        # "Raise Internal Flag"
        # "If New Data Available"
        # "From Shift Reg"
        # "Perforrm Indivudual Angle Calculation"
        # "Pull Down Individual Flag"
        n14 = shared-variable "RT myRIO Target - Overlord\\Localization_Variables_r0.lvlib\\RIGHT_BEACON_X_array"() -> (w73:dbl[])  [unwired: 1 in, 1 out]
        "RIGHT Beacon Coord - X px (IN)" <- w73
        n15 = shared-variable "RT myRIO Target - Overlord\\Localization_Variables_r0.lvlib\\Image Lock - R"() -> (w68:bool)  [unwired: 1 in, 1 out]
        n16 = shared-variable "RT myRIO Target - Overlord\\Localization_Variables_r0.lvlib\\RIGHT_BEACON_Scales"() -> (→"Beacon Scales - Right":sgl[])  [unwired: 1 in, 1 out]
        n17 = shared-variable "RT myRIO Target - Overlord\\Localization_Variables_r0.lvlib\\Info - Right"() -> (w65:T5)  [unwired: 1 in, 1 out]
        n18 = shared-variable "RT myRIO Target - Overlord\\Localization_Variables_r0.lvlib\\RIGHT_BEACON_Y_array"() -> (w72:dbl[])  [unwired: 1 in, 1 out]
        "RIGHT Beacon Position - Y px (IN)" <- w72
        n19 = shared-variable "RT myRIO Target - Overlord\\Localization_Variables_r0.lvlib\\RIGHT_BEACON_BOOL_array"() -> (w71:bool[])  [unwired: 1 in, 1 out]
        "Beacons Found\n- Right (Bool Array)" <- w71
        n20 = Unbundle By Name(w65) -> ("Tracking Coordinates"=w64:cluster{"X":dbl, "Y":dbl}, "Current Valid"=w63:bool, "Current State - Out"=→"Current Cam State - R":T1)
        n21 = local write "Image Lock - Right"(w68) -> ()
        n22 = Bundle("Array of Double"=w73, "Array of Double"=w72) -> (w70:T6)  [unwired: 1 in]
        "Beacon Coordinates - Right Image" <- w70
        n23 = shared-variable "RT myRIO Target - Overlord\\Localization_Variables_r0.lvlib\\Right Servo Angle_Image"() -> (w69:dbl)  [unwired: 1 in, 1 out]
        "This Servo \nAngle - Right" <- w69
        n24 = shared-variable "RT myRIO Target - Overlord\\Localization_Variables_r0.lvlib\\RIGHT_FLAG"(FALSE) -> ()  [unwired: 1 in, 1 out]
        n25 = feedback #1() -> (w81:sgl[])  [unwired: 1 in]
        n26 = feedback #2() -> (w80:bool[])  [unwired: 1 in]
        n27 = call "Angle Calc_Individual Process R4.vi"("Angle to Pixel Ratios"=w77, "Previous Angles"=w81, "Num of Beacons"=w79, "Beacon Coordinates - Image"=w70, "Current Servo Angle"=w69, "Beacons Found (Bool Array)"=w71, "Previous Valid Angles"=w80, "Tracking Coordinates"=w64) -> ("Servo Goal Angle"=w76:sgl, "Valid Beacons (Bool Array)\nPosition Calc"=w75:bool[], "Angle Of Beacons \nRelative to Robot"=w74:sgl[])  [unwired: 4 in, 1 out]
        n28 = feedback-in #1(w74) -> ()
        n29 = feedback-in #2(w75) -> ()
        n30 = local write "Beacon Angles -R"(w74) -> ()
        n31 = local write "Tracking Angle - Right"(w76) -> ()
        n32 = local write "Valid Angles -R"(w75) -> ()
        n33 = local write "Track Angle Valid  - Right"(w63) -> ()
        n34 = local write "New Data  Flag\nRight Servo"(w67) -> ()
      }
    }
    "Right Data\nInput Flag\n- Internal" <- w49
    n35 = case shown="True" w52 {
      tunnel: [w82 w88] -> w48
      tunnel: w60 -> [w82 _]
      tunnel: w56 -> [_ w92]
      tunnel: w57 -> [_ w91]
      frame False {
        # "Don't Update Servo Position\nbc we're waiting on new Data to\ncome in and the servo position\nwas set at the previous set of data"
      }
      frame True {
        w88 = TRUE
        # "Store Values"
        # "Raise Internal Flag"
        # "If New Data Available"
        # "Perforrm Indivudual Angle Calculation"
        # "Pull Down Individual Flag"
        n36 = shared-variable ".\\Localization_Variables_r0.lvlib\\LEFT_BEACON_X_array"() -> (w98:dbl[])  [unwired: 1 in, 1 out]
        "LEFT Beacon Coord - X px (IN) 2" <- w98
        n37 = shared-variable "RT myRIO Target - Overlord\\Localization_Variables_r0.lvlib\\LEFT_BEACON_Scales"() -> (→"Beacon Scales - Left":sgl[])  [unwired: 1 in, 1 out]
        n38 = shared-variable "RT myRIO Target - Overlord\\Localization_Variables_r0.lvlib\\LEFT_BEACON_Y_array"() -> (w99:dbl[])  [unwired: 1 in, 1 out]
        "LEFT Beacon Position - Y px (IN) 2" <- w99
        n39 = shared-variable "RT myRIO Target - Overlord\\Localization_Variables_r0.lvlib\\LEFT_BEACON_BOOL_array"() -> (w100:bool[])  [unwired: 1 in, 1 out]
        "Beacons Found\n- Left (Bool Array) 2" <- w100
        n40 = shared-variable "RT myRIO Target - Overlord\\Localization_Variables_r0.lvlib\\Image Lock - L"() -> (w89:bool)  [unwired: 1 in, 1 out]
        n41 = shared-variable "RT myRIO Target - Overlord\\Localization_Variables_r0.lvlib\\Info - Left"() -> (w86:T5)  [unwired: 1 in, 1 out]
        n42 = Unbundle By Name(w86) -> ("Tracking Coordinates"=w85:cluster{"X":dbl, "Y":dbl}, "Current Valid"=w84:bool, "Current State - Out"=→"Current Cam State - L":T1)
        n43 = local write "Image Lock - Left"(w89) -> ()
        n44 = Bundle("Array of Double"=w98, "Array of Double"=w99) -> (w96:T6)  [unwired: 1 in]
        "Beacon Coordinates - Left Image" <- w96
        n45 = shared-variable "RT myRIO Target - Overlord\\Localization_Variables_r0.lvlib\\Left Servo Angle_Image"() -> (w90:dbl)  [unwired: 1 in, 1 out]
        "This Servo \nAngle - Left" <- w90
        n46 = shared-variable "RT myRIO Target - Overlord\\Localization_Variables_r0.lvlib\\Left_Flag"(FALSE) -> ()  [unwired: 1 in, 1 out]
        n47 = feedback #3() -> (w102:sgl[])  [unwired: 1 in]
        n48 = feedback #4() -> (w101:bool[])  [unwired: 1 in]
        n49 = call "Angle Calc_Individual Process R4.vi"("Angle to Pixel Ratios"=w92, "Previous Angles"=w102, "Num of Beacons"=w91, "Beacon Coordinates - Image"=w96, "Current Servo Angle"=w90, "Beacons Found (Bool Array)"=w100, "Previous Valid Angles"=w101, "Tracking Coordinates"=w85) -> ("Servo Goal Angle"=w95:sgl, "Valid Beacons (Bool Array)\nPosition Calc"=w94:bool[], "Angle Of Beacons \nRelative to Robot"=w93:sgl[])  [unwired: 4 in, 1 out]
        n50 = feedback-in #3(w93) -> ()
        n51 = feedback-in #4(w94) -> ()
        n52 = local write "Beacon Angles - L"(w93) -> ()
        n53 = local write "Valid Angles - L"(w94) -> ()
        n54 = local write "Tracking Angle - Left"(w95) -> ()
        n55 = local write "Track Angle Valid - Left"(w84) -> ()
        n56 = local write "New Data  Flag\nLeft Servo"(w88) -> ()
      }
    }
    "Left Data\nInput Flag\n- Internal" <- w48
    n57 = And(x=w48, y=w49) -> (x .and. y?=w59:bool)
    n58 = case shown="True" w59 {
      selector: w59 -> [_ w105]
      tunnel: w48 -> [w104 _]
      tunnel: [w104 w106] -> w55
      tunnel: [w103 w106] -> w54
      tunnel: w49 -> [w103 _]
      frame False {
      }
      frame True {
        w106 = FALSE
        # "Reset Internal Data Flags"
        # "Position Data\nReady Enabled"
        n59 = local write "Position Calc\nReady"(w105) -> ()
      }
    }
  }
  n60 = Bundle(w34, w34) -> (w37:cluster{sgl, sgl})  [unwired: 1 in]
  n61 = Initialize Array(w34, "History Size") -> (w32:sgl[])
  n62 = Initialize Array(w37, "History Size") -> (w33:cluster{sgl, sgl}[])
  n63 = Initialize Array(FALSE, "History Size") -> (w31:bool[])
  n64 = call "Tick Count4"() -> ("Tick Count(uSec)"=w30:u32)
  n65 = while {
    shift-right: [w117] -> _
    shift-left: w32 -> [w114]
    shift-right: [w116] -> _
    shift-left: w31 -> [w115]
    shift-right: [w118] -> _
    shift-left: w33 -> [w109]
    shift-right: [w110] -> _
    shift-left: w30 -> [w111]
    stop <- "stop" stop-if-true
    n66 = call "Wait5"("Count(mSec)"="Position Calc\nTimer") -> ()  [unwired: 1 out]
    n67 = case shown="True" "Position Calc\nReady" {
      selector: "Position Calc\nReady" -> [_ w187]
      tunnel: w109 -> [_ w209]
      tunnel: w109 -> [w127 w203]
      tunnel: w114 -> [w129 w202]
      tunnel: w115 -> [w128 w201]
      tunnel: [w129 w208] -> w117
      tunnel: [w128 w206] -> w116
      tunnel: [w127 w207] -> w118
      tunnel: w115 -> [_ w200]
      tunnel: w114 -> [_ w199]
      tunnel: [w126 w194] -> w112
      tunnel: w111 -> [_ w194]
      tunnel: [FALSE TRUE] -> w113
      tunnel: w109 -> [_ w189]
      frame False {
        n68 = call "Tick Count5"() -> ("Tick Count(uSec)"=w126:u32)
      }
      frame True {
        # "dY"
        # "dX"
        # "Valid"
        # "Find Local Coordinates"
        # "Valid COunt"
        # "Make sure 2+ Data Sets are Still available"
        # "Check 1st element\nwith rest of elements"
        # "Make Sure all Pointed \nIn Same Direction"
        # "For Each Valid Beacon\nCalculate Distance from Each Camera to Each Beacon"
        # "Find Common Beacons\nAmong Cameras"
        # "Currently will only\ncalculate position if 2+ \nbeacons are available \nfrom both cameras"
        # "System is in Normal (long range) State"
        # "Average Both Data Sets"
        # "Estimate Distance for each Available Beacon Angle\nPER Camera, indivduallly"
        # "At least 2+ Avaialbe"
        # "CALCULATE AVERAGE ORIENTATION"
        # "Update Outputs\nif Current Calc is Invalid\n(shouldn't matter)"
        # "Estimate Orienation Based on Previous Position"
        # "****# of previous in history that must be true\nin order for position to be considered \"locked\""
        # "New Position is Valid if both \nOrientation and Positions\nis within range of previous"
        # "Robot Position\n Shift Array"
        # "Position Valid Shift Array"
        # "Orientation Shift Array"
        # "Orientation Value"
        # "Shift & Insert Current Position Valid"
        # "Position Valid\n(orientation)"
        # "Position Valid\n(position)"
        # "Update Shift Registers"
        # "Shift & Insert Current Calculated Orientation"
        # "Shift & Insert Current Robot Position"
        # "UPDATE FINAL OUTPUT\n VALUES"
        n69 = local read "Num of Beacons (Total)"() -> (w170:i8)
        n70 = Not(x=w187) -> (.not. x?=w188:bool)
        n71 = local write "Position Calc\nReady"(w188) -> ()
        n72 = disable-structure shown="Disabled" {
          frame Disabled {
            w210 = T1."Normal - 5" ("Initial State")
            # "***********do for both"
            # "sTATE"
            n73 = local read "Current Cam State - L"() -> (w214:T1)
            n74 = local read "Current Cam State - R"() -> (w213:T1)
            n75 = Equal?(x=w214, y=w210) -> (x = y?=w212:bool)
            n76 = Equal?(x=w213, y=w210) -> (x = y?=w211:bool)
            n77 = And(x=w212, y=w211) -> ()  [unwired: 1 out]
          }
          frame Enabled {
          }
        }
        n78 = local read "Beacon Scales - Left"() -> (w176:sgl[])
        n79 = local read "Beacon Scales - Right"() -> (w173:sgl[])
        n80 = for {
          N: w170 -> [_]
          tunnel: "Valid Angles - L" -> [w346] mode=indexing
          tunnel: "Beacon Angles - L" -> [w353] mode=indexing
          tunnel: w176 -> [w354] mode=indexing
          tunnel: "Valid Angles -R" -> [w345] mode=indexing
          tunnel: "Beacon Angles -R" -> [w352] mode=indexing
          tunnel: w173 -> [w351] mode=indexing
          tunnel: "Distance Between \nCameras  (*unit)" -> [w350]
          tunnel: [w344] -> w167 mode=indexing
          tunnel: [w343] -> w166 mode=indexing
          tunnel: [w342] -> w168 mode=indexing
          tunnel: [w341] -> w132 mode=indexing
          tunnel: [w340] -> w131 mode=indexing
          tunnel: [w339] -> w130 mode=indexing
          # "dY"
          # "dX"
          # "Valid"
          # "If Both Cameras are using Same Beacon Data,\nAverage the 2 independently esitmated positions"
          # "dY"
          # "dX"
          # "dY"
          # "dX"
          n81 = case shown="True" w346 {
            tunnel: w353 -> [_ w431]
            tunnel: [w418 w422] -> w348
            tunnel: [w418 w423] -> w347
            tunnel: w354 -> [_ w419]
            frame False {
              w418 = sgl 0.0
              # "Current Data Set Was Not Valid\nFill with 0\nWill not be used later"
            }
            frame True {
              # "Estimate Distance"
              # "Negate dX if A2>90"
              # "Find LOCAL Coordinate of Each Beacon"
              # "Current - Valid Data Set"
              n82 = call "Scaling and Mapping"("Signals"=w419) -> ("Scaled Signals"=w420:dynamicdata)  [unwired: 9 in, 1 out]
              n83 = To Single Precision Float(number=w420) -> (single precision float=w421:sgl)
              n84 = Less?(x=w431, y=sgl 90.0) -> (x < y?=w433:bool)
              n85 = case shown="False" w433 {
                tunnel: w431 -> [w440 w442]
                tunnel: [w438 w443] -> w430
                tunnel: [FALSE TRUE] -> w425
                frame False {
                  # "Negative Y"
                  # "A2 is > 90"
                  n86 = Subtract(x=w440, y=sgl 90.0) -> (x-y=w438:sgl)
                }
                frame True {
                  # "Positive Y"
                  # "A2 is < 90"
                  n87 = Subtract(x=sgl 90.0, y=w442) -> (x-y=w443:sgl)
                }
              }
              "dA2 2" <- w430
              n88 = expression code="(x/180.0)*pi" "degrees to radians"(w430) -> (w428:sgl)
              n89 = expression code="(x/180.0)*pi" "degrees to radians"(w430) -> (w429:sgl)
              n90 = Cosine(x=w428) -> (cos(x)=w426:sgl)
              n91 = Sine(x=w429) -> (sin(x)=w427:sgl)
              n92 = Multiply(x=w421, y=w426) -> (x*y=w423:sgl)
              n93 = Multiply(x=w421, y=w427) -> (x*y=w424:sgl)
              n94 = case shown="True" w425 {
                tunnel: w424 -> [w435 w436]
                tunnel: [w434 w436] -> w422
                frame False {
                  n95 = Negate(x=w435) -> (-x=w434:sgl)
                }
                frame True {
                }
              }
            }
          }
          n96 = case shown="True" w345 {
            tunnel: w352 -> [_ w404]
            tunnel: [w389 w392] -> w340
            tunnel: [w389 w391] -> w341
            tunnel: w351 -> [_ w396]
            tunnel: w350 -> [_ w393]
            tunnel: [w389 w390] -> w339
            frame False {
              w389 = sgl 0.0
              # "Current Data Set Was Not Valid\nFill with 0\nWill not be used later"
            }
            frame True {
              # "Add delta for\nRIGHT camera ONLY"
              # "Estimate Distance"
              # "Negate dX if A2>90"
              # "Find LOCAL Coordinate of Each Beacon"
              # "Current - Valid Data Set"
              n97 = call "Scaling and Mapping2"("Signals"=w396) -> ("Scaled Signals"=w395:dynamicdata)  [unwired: 9 in, 1 out]
              n98 = To Single Precision Float(number=w395) -> (single precision float=w394:sgl)
              n99 = Less?(x=w404, y=sgl 90.0) -> (x < y?=w406:bool)
              n100 = case shown="False" w406 {
                tunnel: w404 -> [w413 w415]
                tunnel: [w411 w416] -> w403
                tunnel: [FALSE TRUE] -> w398
                frame False {
                  # "Negative Y"
                  # "A2 is > 90"
                  n101 = Subtract(x=w413, y=sgl 90.0) -> (x-y=w411:sgl)
                }
                frame True {
                  # "Positive Y"
                  # "A2 is < 90"
                  n102 = Subtract(x=sgl 90.0, y=w415) -> (x-y=w416:sgl)
                }
              }
              "dA2 3" <- w403
              n103 = expression code="(x/180.0)*pi" "degrees to radians"(w403) -> (w401:sgl)
              n104 = expression code="(x/180.0)*pi" "degrees to radians"(w403) -> (w402:sgl)
              n105 = Cosine(x=w401) -> (cos(x)=w399:sgl)
              n106 = Sine(x=w402) -> (sin(x)=w400:sgl)
              n107 = Multiply(x=w394, y=w399) -> (x*y=w391:sgl)
              n108 = Multiply(x=w394, y=w400) -> (x*y=w397:sgl)
              n109 = case shown="True" w398 {
                tunnel: w397 -> [w408 w409]
                tunnel: [w407 w409] -> w390
                frame False {
                  n110 = Negate(x=w408) -> (-x=w407:sgl)
                }
                frame True {
                }
              }
              n111 = Add(x=w393, y=w390) -> (x+y=w392:sgl)
            }
          }
          n112 = And(x=w346, y=w345) -> (x .and. y?=w349:bool)
          n113 = case shown="False" w349 {
            tunnel: w348 -> [w362 w388]
            tunnel: w347 -> [w359 w387]
            tunnel: w340 -> [w361 w386]
            tunnel: w341 -> [w360 w385]
            tunnel: [w357 w381] -> w344
            tunnel: [w356 w380] -> w343
            tunnel: w346 -> [w358 _]
            tunnel: w345 -> [w363 _]
            tunnel: [w355 TRUE] -> w342
            frame False {
              n114 = Exclusive Or(1:w363, 2:w358) -> (0:w364:bool)
              n115 = case shown="True" w364 {
                tunnel: w362 -> [_ w372]
                tunnel: w361 -> [_ w369]
                tunnel: w360 -> [_ w368]
                tunnel: w359 -> [_ w370]
                tunnel: w358 -> [_ w374]
                tunnel: [w365 w373] -> w357
                tunnel: [w365 w371] -> w356
                tunnel: [FALSE TRUE] -> w355
                frame False {
                  w365 = sgl 0.0
                  # "None are valid,"
                }
                frame True {
                  # "Only 1 beacon is valid,\nUse the valid beacon"
                  n116 = case shown="False" w374 {
                    tunnel: [w376 w378] -> w373
                    tunnel: w372 -> [_ w378]
                    tunnel: [w375 w377] -> w371
                    tunnel: w370 -> [_ w377]
                    tunnel: w369 -> [w376 _]
                    tunnel: w368 -> [w375 _]
                    frame False {
                      # "Left is invalid,\nRight MUST be valid"
                    }
                    frame True {
                      # "Left is Valid"
                    }
                  }
                }
              }
            }
            frame True {
              w382 = sgl 2.0 ("y")
              # "Both are Valid"
              n117 = Add(x=w388, y=w386) -> (x+y=w383:sgl)
              n118 = Add(x=w387, y=w385) -> (x+y=w384:sgl)
              n119 = Divide(x=w384, y=w382) -> (x/y=w380:sgl)
              n120 = Divide(x=w383, y=w382) -> (x/y=w381:sgl)
            }
          }
        }
        "Array" <- w132
        "Array 2" <- w131
        "Array 3" <- w130
        n121 = And(x="Valid Angles - L", y="Valid Angles -R") -> (x .and. y?=w158:bool[])
        n122 = Boolean To (0,1)(Boolean=w158) -> (0, 1=w155:i16[])
        n123 = Add Array Elements(numeric array=w155) -> (sum=w156:i16)
        n124 = Greater?(x=w156, y=1) -> (0:w154:bool)
        n125 = for {
          N: w170 -> [_]
          tunnel: w154 -> [w275]
          tunnel: "Beacon Angles - L" -> [w274] mode=indexing
          tunnel: "Beacon Angles -R" -> [w273] mode=indexing
          tunnel: "Distance Between \nCameras  (*unit)" -> [w272]
          tunnel: "Distance Threshold\nRef Triangles (*unit)" -> [w271]
          tunnel: [w270] -> w141 mode=indexing
          tunnel: [w269] -> _ mode=indexing
          tunnel: [w268] -> w140 mode=indexing
          tunnel: [w267] -> _ mode=indexing
          tunnel: [w266] -> w142 mode=indexing
          tunnel: [w265] -> w148 mode=indexing
          n126 = case shown="True" w275 {
            tunnel: w274 -> [w280 w290]
            tunnel: w273 -> [w279 w289]
            tunnel: w272 -> [_ w281]
            tunnel: w271 -> [_ w282]
            tunnel: [w280 w288] -> w270
            tunnel: [w279 w287] -> w269
            tunnel: [FALSE w286] -> w268
            tunnel: [w277 w285] -> w267
            tunnel: [w277 w284] -> w266
            tunnel: [0 w283] -> w265
            frame False {
              w277 = sgl 1.0
            }
            frame True {
              # "Build Reference Triangle"
              n127 = call "Position Calc_Build Reference Triangle_R1.vi"("A2_in"=w290, "A3_in"=w289, "S1 (Length Between\n Cameras - inches)"=w281, "Distance\nThreshold"=w282) -> ("S2"=w285:sgl, "S3"=w284:sgl, "Direction"=w283:i8, "A2"=w288:sgl, "A3"=w287:sgl, "Accept"=w286:bool)  [unwired: 6 in]
            }
          }
        }
        n128 = for {
          N: w170 -> [_]
          tunnel: w140 -> [w260] mode=indexing
          tunnel: w148 -> [w264] mode=indexing
          tunnel: [w264] -> w150 mode=indexing if=w260
          shift-right: [w263] -> w144
          shift-left: 0 -> [w261]
          # "Only add to array\nif valid distance"
          n129 = Increment(x=w261) -> (x+1=w262:i32)
          n130 = Select(t=w262, s=w260, f=w261) -> (s? t:f=w263:i32)
        }
        n131 = Index Array(array=w150, index=0) -> (element=w151:i32)
        n132 = Equal?(x=w150, y=w151) -> (x = y?=w152:bool[])
        n133 = And Array Elements(Boolean array=w152) -> (logical AND=w146:bool)
        n134 = Greater?(x=w144, y=1) -> (0:w145:bool)
        n135 = And(x=w146, y=w145) -> (x .and. y?=w139:bool)
        n136 = case shown="True" w139 {
          tunnel: w170 -> [w217 w226]
          tunnel: w142 -> [_ w225]
          tunnel: w141 -> [_ w224]
          tunnel: w140 -> [_ w223]
          tunnel: [w216 w222] -> w169
          tunnel: [w215 w221] -> w165
          tunnel: [w215 w220] -> w164
          frame False {
            # "Build Array for False"
            n137 = for {
              N: w217 -> [_]
              tunnel: [sgl 0.0] -> w215 mode=indexing
              tunnel: [FALSE] -> w216 mode=indexing
            }
          }
          frame True {
            n138 = for {
              N: w226 -> [_]
              tunnel: w224 -> [w232] mode=indexing
              tunnel: w225 -> [w231] mode=indexing
              tunnel: [w230] -> w221 mode=indexing
              tunnel: [w229] -> w220 mode=indexing
              tunnel: [w228] -> w222 mode=indexing
              tunnel: w223 -> [w227] mode=indexing
              n139 = case shown="True" w227 {
                selector: w227 -> [w234 w238]
                tunnel: w232 -> [_ w246]
                tunnel: [w233 w236] -> w230
                tunnel: [w233 w237] -> w229
                tunnel: w231 -> [_ w235]
                tunnel: [w234 w238] -> w228
                frame False {
                  w233 = sgl 0.0
                  # "Current Data Set Was Not Valid\nFill with 0\nWill not be used later"
                }
                frame True {
                  # "dY"
                  # "dX"
                  # "Negate dX if A2>90"
                  # "Find LOCAL Coordinate of Each Beacon"
                  # "Current - Valid Data Set"
                  n140 = Less?(x=w246, y=sgl 90.0) -> (x < y?=w248:bool)
                  n141 = case shown="False" w248 {
                    tunnel: w246 -> [w255 w257]
                    tunnel: [w253 w258] -> w245
                    tunnel: [FALSE TRUE] -> w240
                    frame False {
                      # "Negative Y"
                      # "A2 is > 90"
                      n142 = Subtract(x=w255, y=sgl 90.0) -> (x-y=w253:sgl)
                    }
                    frame True {
                      # "Positive Y"
                      # "A2 is < 90"
                      n143 = Subtract(x=sgl 90.0, y=w257) -> (x-y=w258:sgl)
                    }
                  }
                  "dA2 4" <- w245
                  n144 = expression code="(x/180.0)*pi" "degrees to radians"(w245) -> (w243:sgl)
                  n145 = expression code="(x/180.0)*pi" "degrees to radians"(w245) -> (w244:sgl)
                  n146 = Cosine(x=w243) -> (cos(x)=w241:sgl)
                  n147 = Sine(x=w244) -> (sin(x)=w242:sgl)
                  n148 = Multiply(x=w235, y=w241) -> (x*y=w237:sgl)
                  n149 = Multiply(x=w235, y=w242) -> (x*y=w239:sgl)
                  n150 = case shown="True" w240 {
                    tunnel: w239 -> [w250 w251]
                    tunnel: [w249 w251] -> w236
                    frame False {
                      n151 = Negate(x=w250) -> (-x=w249:sgl)
                    }
                    frame True {
                    }
                  }
                }
              }
            }
          }
        }
        n152 = Subtract(x=sgl 1.0, y="Triangle Based\nWeight") -> (x-y=w161:sgl)
        "Scale Based\nWeight" <- w161
        n153 = for {
          N: w170 -> [_]
          tunnel: w169 -> [w295] mode=indexing
          tunnel: w168 -> [w294] mode=indexing
          tunnel: w167 -> [w299] mode=indexing
          tunnel: w166 -> [w298] mode=indexing
          tunnel: w165 -> [w301] mode=indexing
          tunnel: w164 -> [w300] mode=indexing
          tunnel: "Triangle Based\nWeight" -> [w297]
          tunnel: w161 -> [w296]
          tunnel: [w293] -> w138 mode=indexing
          tunnel: [w292] -> w160 mode=indexing
          tunnel: [w291] -> w159 mode=indexing
          # "If Beacon info \nis available from\nboth"
          n154 = And(x=w295, y=w294) -> (x .and. y?=w302:bool)
          n155 = case shown="True" w302 {
            selector: w302 -> [_ w328]
            tunnel: w301 -> [w309 w336]
            tunnel: w300 -> [w307 w337]
            tunnel: w299 -> [w305 w335]
            tunnel: w298 -> [w304 w334]
            tunnel: w297 -> [_ w338]
            tunnel: w296 -> [_ w333]
            tunnel: [w308 w326] -> w291
            tunnel: [w310 w327] -> w292
            tunnel: w295 -> [w311 _]
            tunnel: w294 -> [w306 _]
            tunnel: [w303 w328] -> w293
            frame False {
              n156 = case shown="False" w311 {
                selector: w311 -> [_ w323]
                tunnel: [w316 w325] -> w310
                tunnel: w309 -> [_ w325]
                tunnel: [w314 w324] -> w308
                tunnel: w307 -> [_ w324]
                tunnel: w306 -> [w317 _]
                tunnel: w305 -> [w315 _]
                tunnel: w304 -> [w313 _]
                tunnel: [w312 w323] -> w303
                frame False {
                  n157 = case shown="False" w317 {
                    selector: w317 -> [w318 w320]
                    tunnel: [w319 w322] -> w316
                    tunnel: w315 -> [_ w322]
                    tunnel: [w319 w321] -> w314
                    tunnel: w313 -> [_ w321]
                    tunnel: [w318 w320] -> w312
                    frame False {
                      w319 = sgl 0.0
                      # "None avail"
                    }
                    frame True {
                    }
                  }
                }
                frame True {
                }
              }
            }
            frame True {
              n158 = Multiply(x=w336, y=w338) -> (x*y=w332:sgl)
              n159 = Multiply(x=w337, y=w338) -> (x*y=w330:sgl)
              n160 = Multiply(x=w335, y=w333) -> (x*y=w331:sgl)
              n161 = Multiply(x=w334, y=w333) -> (x*y=w329:sgl)
              n162 = Add(x=w332, y=w331) -> (x+y=w327:sgl)
              n163 = Add(x=w330, y=w329) -> (x+y=w326:sgl)
            }
          }
        }
        "Valid Beacon Sets_" <- w138
        n164 = Boolean To (0,1)(Boolean=w138) -> (0, 1=w181:i16[])
        n165 = Add Array Elements(numeric array=w181) -> (sum=w180:i16)
        n166 = Greater?(x=w180, y=i16 1) -> (0:w178:bool)
        n167 = case shown="True" w178 {
          tunnel: w209 -> [_ w535]
          tunnel: [0.0 ("f") w534] -> w205
          tunnel: [w447 w533] -> w204
          tunnel: w200 -> [_ w452]
          tunnel: w199 -> [_ w532]
          tunnel: [FALSE w531] -> w192
          tunnel: [FALSE w530] -> w191
          tunnel: w189 -> [_ w529]
          tunnel: [sgl 0.0 w527] -> w182
          tunnel: "Distance Between \nCameras  (*unit)" -> [_ w464]
          tunnel: w160 -> [_ w463]
          tunnel: w159 -> [_ w462]
          tunnel: w138 -> [_ w461]
          tunnel: w170 -> [_ w460]
          frame False {
            w446 = 0.0 ("f")
            n168 = Bundle("f"=w446, "f"=w446) -> (w447:cluster{"f":dbl, "f":dbl})  [unwired: 1 in]
          }
          frame True {
            w499 = sgl 2.0
            w516 = 0
            # "Current Orientaiton"
            # "Valid Position Ccount\n(within moving avg\nwinfow)"
            # "Valid Position Ccount"
            # "Only Apply This Filtering \nif 3 or More Beacons Still Valid"
            # "Orientation Value"
            # "Orientation Valid"
            # "Y (current)"
            # "X (current)"
            # "Number of Valid\nPrevious Orientations"
            # "More than 1 Previous\nValid Positions"
            # "More than\n2previous position\navailable"
            # "Choose Beacon Set\nwith Lowest Std Dev"
            # "Y value cannot be negative"
            # "Find New # Of Valid Beacons"
            # "Adjust/Normalize\nLocal Beacon Positions\nusing Line of Best fit"
            # "# Valid\nData Sets"
            # "cam, y"
            # "cam, x"
            # "Calculate dX and dY\nfor right cam"
            # "Average dX and dY from each (valid) beacon to find position of each camera\n\nthen average all  positions for each camera find center between"
            # "Convert Slope\nto Radians"
            # "*rotate CCW in rad"
            # "Rotate Coordinate\n System by Slope"
            n169 = Boolean To (0,1)(Boolean=w452) -> (0, 1=w483:i16[])
            n170 = Initialize Array(u8 0, "Moving Average\nWindow Length") -> (w457:u8[])
            n171 = Add Array Elements(numeric array=w483) -> (sum=w451:i16)
            n172 = Greater?(x=w451, y=0) -> (0:w454:bool)
            n173 = while {
              shift-right: [w537] -> w455
              shift-left: w457 -> [w539]
              tunnel: w452 -> [w544] mode=indexing
              shift-right: [w543] -> w453
              shift-left: u8 0 -> [w545]
              tunnel: "Moving Average\nWindow Length" -> [w536]
              i -> [w538]
              stop <- w540 stop-if-true
              # "Grab Last 2 Valid Position Indexes"
              n174 = case shown="True" w544 {
                tunnel: w545 -> [w547 w549]
                tunnel: [w547 w552] -> w543
                tunnel: w539 -> [w546 w551]
                tunnel: w538 -> [_ w550]
                tunnel: [w546 w548] -> w537
                frame False {
                }
                frame True {
                  # "Update Index\nto use"
                  # "Increment\nValid Count"
                  n175 = Replace Array Subset(array=w551, new element=w550, index=w549) -> (w548:u8[])
                  n176 = Increment(x=w549) -> (x+1=w552:u8)
                }
              }
              n177 = Greater Or Equal?(x=w543, y=w536) -> (x >= y?=w542:bool)
              n178 = Greater Or Equal?(x=w538, y=w536) -> (x >= y?=w541:bool)
              n179 = Or(x=w542, y=w541) -> (x .or. y?=w540:bool)
            }
            n180 = Bundle(w463, w462) -> (→"LOCAL\nBeacon Coordinates\nRelative to Robot" →"Local Coordinates - Calculated":cluster{sgl[], sgl[]})  [unwired: 1 in]
            n181 = call "Coordinate_Outlier_Filtering_R2.vi"("Num of Beacons"=w460, "Max Std Dev(all 5)"="Max Std Dev (5)", "X in"=w463, "Valid Data\nSets in"=w461, "Y in"=w462, "Max Std Dev( 4 )"="Max Std Dev (4)", "Max Std Dev (3)"="Max Std Dev (3)") -> ("Y out"=w474:sgl[], "X out"=w475:sgl[], "Valid Beacons\nout"=w472:bool[], "Slope out"=w480:dbl)  [unwired: 3 in, 2 out]
            n182 = Inverse Tangent(1:w480) -> (0:w495:dbl)
            n183 = expression code="(x/pi)*180.0" "radians to degrees"(w495) -> (w479:dbl)
            n184 = Boolean To (0,1)(Boolean=w472) -> (0, 1=w471:i16[])
            n185 = To Single Precision Float(number=w479) -> (single precision float=w527:sgl)
            n186 = case shown="True" w454 {
              tunnel: [w562 w580] -> w530
              tunnel: w532 -> [_ w582]
              tunnel: w527 -> [w563 w577]
              tunnel: [w561 w581] -> w534
              tunnel: w529 -> [_ _]
              tunnel: w455 -> [_ w578]
              tunnel: w453 -> [_ w568]
              frame False {
                # "Since no history available,\ncheck that current is with 0-360"
                # "Use Current Orientation bc \nPrevious are not available"
                # "New Position\nValid"
                n187 = In Range and Coerce(upper limit=sgl 360.0, x=w563, lower limit=sgl -360.0 ("upper limit")) -> (In Range?=w562:bool)  [unwired: 1 out]
                n188 = Select(t=w563, s=w562, f=sgl 0.0) -> (s? t:f=w561:sgl)
              }
              frame True {
                # "Moving Average Out"
                n189 = for {
                  N: w568 -> [_]
                  shift-right: [w606] -> w574
                  shift-left: 0.0 -> [w605]
                  tunnel: w578 -> [w604] mode=indexing
                  tunnel: w582 -> [w602]
                  # "Fetch Last Valid Values\nand Sum"
                  n190 = Index Array(array=w602, index=w604) -> (element=w603:sgl)
                  n191 = Add(x=w603, y=w605) -> (x+y=w606:dbl)
                }
                n192 = Subtract(x=sgl 1.0, y="New Orientation\nWeight") -> (x-y=w573:sgl)
                n193 = Multiply(x=w577, y="New Orientation\nWeight") -> (x*y=w571:sgl)
                n194 = Multiply(x=w573, y=w574) -> (x*y=w569:dbl)
                n195 = To Double Precision Float(number=w568) -> (double precision float=w567:dbl)
                n196 = Divide(x=w569, y=w567) -> (x/y=w570:dbl)
                n197 = Add(x=w571, y=w570) -> (x+y=w572:dbl)
                n198 = Greater Than 0?(x=w568) -> (x > 0?=w579:bool)
                n199 = case shown="True" w579 {
                  tunnel: w572 -> [w586 w592]
                  tunnel: w578 -> [_ w599]
                  tunnel: w582 -> [_ w598]
                  tunnel: [w585 w591] -> w581
                  tunnel: [w584 w594] -> w580
                  frame False {
                    # "No Pevious is Available to Compare\ncheck that current is real angle"
                    n200 = In Range and Coerce(upper limit=sgl 360.0, x=w586, lower limit=sgl -360.0 ("upper limit")) -> (In Range?=w584:bool)  [unwired: 1 out]
                    n201 = Select(t=w586, s=w584, f=sgl 0.0) -> (s? t:f=w585:dbl)
                  }
                  frame True {
                    # "Calculate New, Weighted\nOrientation"
                    # "Check That New Value\nis within Range of Old\n(avg)"
                    # "(X1 - X2)^2"
                    # "Previous"
                    # "Pevious is Available to Compare"
                    n202 = Index Array(array=w599, index=u8 0) -> (element=w600:u8)
                    n203 = Index Array(array=w598, index=w600) -> (element=w597:sgl)
                    n204 = Subtract(x=w597, y=w592) -> (x-y=w596:dbl)
                    n205 = Absolute Value(x=w596) -> (abs(x)=w595:dbl)
                    n206 = Less Or Equal?(x=w595, y="New Orientation \nThreshold") -> (x <= y?=w594:bool)
                    n207 = Select(t=w592, s=w594, f=sgl 0.0) -> (s? t:f=w591:dbl)
                  }
                }
              }
            }
            n208 = Add Array Elements(numeric array=w471) -> (sum=w470:i16)
            n209 = Greater?(x=w470, y=i16 2) -> (0:w468:bool)
            n210 = case shown="True" w468 {
              tunnel: w460 -> [_ w560]
              tunnel: w472 -> [w553 w559]
              tunnel: w475 -> [_ w558]
              tunnel: w474 -> [_ w557]
              tunnel: [w553 w556] -> w473
              tunnel: "Distance\nBetween Beacons" -> [_ w555]
              tunnel: "Distance\nBetween Beacons \n- Tolerance" -> [_ w554]
              frame False {
                # "Don't apply filtering,\nnot enough data points"
              }
              frame True {
                # "This will filter beacons if they are calculate to be \ntoo close to each other. The beacon(s) that is\n discarded is chosen based distance between each/every\nbeacon,. Capable of filtering as long as 1/2 of sample\nset has uniform distances (between beacons)."
                # "Validate Distance Between\nEach Beacon"
                n211 = call "Beacon_Filtering_Inter_Beacon_Distance_R1.vi"("Num of Beacons"=w560, "Inter Beacon\nReal Distance"=w555, "X in"=w558, "Inter Beacon\ndelta Threshold"=w554, "Y in"=w557, "Valid Data\nSets in"=w559) -> ("Beacons Valid - Out"=w556:bool[])  [unwired: 9 in]
              }
            }
            "Post Filtering\n- Valid Beacons" <- w473
            n212 = Increment(x=w460) -> (x+1=w517:i8)
            n213 = for {
              N: w517 -> [_]
              tunnel: [w722] -> w518 mode=indexing
              tunnel: w475 -> [w718]
              tunnel: w474 -> [w721]
              tunnel: [w720] -> w519 mode=indexing
              tunnel: w464 -> [w717]
              i -> [w719]
              # "Build Array's of Coordinates\nFor All Objects"
              n214 = Greater Than 0?(x=w719) -> (x > 0?=w723:bool)
              n215 = case shown="True" w723 {
                tunnel: [w725 w731] -> w722
                tunnel: w718 -> [w728 _]
                tunnel: w721 -> [w727 _]
                tunnel: [w724 0.0] -> w720
                tunnel: w719 -> [w729 _]
                tunnel: w717 -> [_ w731]
                frame True {
                  # "Rest of Array is\nBeacon Coordinates"
                  n216 = Decrement(x=w729) -> (x-1=w726:i32)
                  n217 = Index Array(array=w728, index=w726) -> (element=w725:sgl)
                  n218 = Index Array(array=w727, index=w726) -> (element=w724:sgl)
                }
                frame False {
                  # "First object is the\nother Camera\n\nthis coordinate\nis simply:\nx = 0\ny = distance btween cams"
                }
              }
            }
            n219 = Bundle(w518, w519) -> (→"All Object Coordinates \n- Local" →"Local Coordinates - Normalized":cluster{sgl[], dbl[]})  [unwired: 1 in]
            n220 = expression code="(x/180.0)*pi" "degrees to radians"(w534) -> (w478:dbl)
            n221 = call-poly <vilib>:"2D Cartesian Coordinate Rotation.vi"("theta"=w478, "Y"=w519, "X"=w518) -> ("Y Out"=w496:dbl[], "X Out"=w497:dbl[])  [unwired: 6 in, 1 out]
            n222 = Bundle("X Out"=w497, "Y Out"=w496) -> (→"All Object Coordinates \n- Local - Rotated" →"Local Coordinates - Rotated":cluster{"X Out":dbl[], "Y Out":dbl[]})  [unwired: 1 in]
            n223 = Index Array(array=w496, index=w516) -> (element=w492:dbl)
            n224 = Index Array(array=w497, index=w516) -> (element=w515:dbl)
            n225 = for {
              N: w460 -> [_]
              tunnel: w496 -> [w713]
              tunnel: w497 -> [w714]
              tunnel: w515 -> [w712]
              tunnel: w492 -> [w711]
              tunnel: [w710] -> w489 mode=indexing
              tunnel: [w709] -> w488 mode=indexing
              tunnel: [w708] -> w465 mode=indexing
              tunnel: [w707] -> w490 mode=indexing
              i -> [w716]
              n226 = Increment(x=w716) -> (x+1=w715:i32)
              n227 = Index Array(array=w713, index=w715) -> (element=w707:dbl)
              n228 = Index Array(array=w714, index=w715) -> (element=w708:dbl)
              n229 = Subtract(x=w707, y=w711) -> (x-y=w709:dbl)
              n230 = Subtract(x=w708, y=w712) -> (x-y=w710:dbl)
            }
            n231 = Bundle(w489, w488) -> (→"dX, dY\nRight Cam":cluster{dbl[], dbl[]})  [unwired: 1 in]
            n232 = Bundle(w465, w490) -> (→"dX, dY\nLeft Cam":cluster{dbl[], dbl[]})  [unwired: 1 in]
            n233 = Unbundle("Real Beacon\n - Coordinates") -> ("X"=w513:dbl[], "Y"=w493:dbl[])
            n234 = Boolean To (0,1)(Boolean=w473) -> (0, 1=w491:i16[])
            n235 = for {
              N: w460 -> [_]
              tunnel: w473 -> [w693] mode=indexing
              tunnel: w513 -> [w690] mode=indexing
              tunnel: w493 -> [w689] mode=indexing
              tunnel: w465 -> [w692] mode=indexing
              tunnel: w490 -> [w688] mode=indexing
              tunnel: w489 -> [w691] mode=indexing
              tunnel: w488 -> [w687] mode=indexing
              tunnel: [w686] -> w512 mode=indexing
              tunnel: [w685] -> w511 mode=indexing
              tunnel: [w684] -> w510 mode=indexing
              tunnel: [w683] -> w509 mode=indexing
              n236 = case shown="True" w693 {
                tunnel: w692 -> [_ w706]
                tunnel: w691 -> [_ w705]
                tunnel: w690 -> [_ w696]
                tunnel: w689 -> [_ w695]
                tunnel: w688 -> [_ w704]
                tunnel: w687 -> [_ w697]
                tunnel: [w694 w702] -> w686
                tunnel: [w694 w701] -> w685
                tunnel: [w694 w700] -> w684
                tunnel: [w694 w699] -> w683
                frame False {
                  w694 = sgl 0.0
                  # "Add Nothing"
                }
                frame True {
                  # "realX = beaconX + dY\nrealY = beaconY + (-dx)"
                  # "Right Cam"
                  # "Left Cam"
                  # "dX = -dX\nSwap dX, dY"
                  # "Translate to Real Coordinates\nOnly Apply for Valid Beacons"
                  n237 = Negate(x=w706) -> (-x=w703:dbl)
                  n238 = Negate(x=w705) -> (-x=w698:dbl)
                  n239 = Add(x=w696, y=w704) -> (x+y=w702:dbl)
                  n240 = Add(x=w695, y=w703) -> (x+y=w701:dbl)
                  n241 = Add(x=w696, y=w697) -> (x+y=w700:dbl)
                  n242 = Add(x=w695, y=w698) -> (x+y=w699:dbl)
                }
              }
            }
            n243 = Add Array Elements(numeric array=w491) -> (sum=w494:i16)
            n244 = Add Array Elements(numeric array=w512) -> (sum=w508:dbl)
            n245 = Add Array Elements(numeric array=w511) -> (sum=w507:dbl)
            n246 = Add Array Elements(numeric array=w510) -> (sum=w506:dbl)
            n247 = Add Array Elements(numeric array=w509) -> (sum=w505:dbl)
            n248 = Divide(x=w508, y=w494) -> (x/y=w504:dbl)
            n249 = Divide(x=w507, y=w494) -> (x/y=w502:dbl)
            n250 = Divide(x=w506, y=w494) -> (x/y=w503:dbl)
            n251 = Divide(x=w505, y=w494) -> (x/y=w501:dbl)
            n252 = Bundle(w504, w502) -> (→"Left Camera Real Coordinates":cluster{dbl, dbl})  [unwired: 1 in]
            n253 = Bundle(w503, w501) -> (→"Right Camera Real Coordinate":cluster{dbl, dbl})  [unwired: 1 in]
            n254 = Add(x=w504, y=w503) -> (x+y=w500:dbl)
            n255 = Add(x=w502, y=w501) -> (x+y=w498:dbl)
            n256 = Divide(x=w500, y=w499) -> (x/y=w482:dbl)
            n257 = Divide(x=w498, y=w499) -> (x/y=w481:dbl)
            n258 = Bundle(w482, w481) -> (→"Robot Coordinates":cluster{dbl, dbl})  [unwired: 1 in]
            n259 = Less Than 0?(x=w481) -> ()  [unwired: 1 out]
            n260 = case shown="True" w454 {
              tunnel: w451 -> [_ _]
              tunnel: w482 -> [w611 w632]
              tunnel: [w612 w642] -> w531
              tunnel: w535 -> [_ w636]
              tunnel: w481 -> [w610 w619]
              tunnel: [w609 w646] -> w533
              tunnel: "Max X (arena)" -> [w608 w641]
              tunnel: "Max Y (arena)" -> [w607 w640]
              tunnel: w455 -> [_ w638]
              tunnel: w453 -> [_ w637]
              frame False {
                # "New Position\nValid"
                # "Since no history available,\ncheck that current is within\nthe bounds of the arena size"
                # "Use Current Position bc \nPrevious are not available"
                n261 = In Range and Coerce(upper limit=w608, x=w611, lower limit=sgl 0.0 ("upper limit")) -> (In Range?=w614:bool)  [unwired: 1 out]
                n262 = In Range and Coerce(upper limit=w607, x=w610, lower limit=sgl 0.0 ("upper limit")) -> (In Range?=w613:bool)  [unwired: 1 out]
                n263 = Bundle(w611, w610) -> (w609:cluster{dbl, dbl})  [unwired: 1 in]
                n264 = And(x=w614, y=w613) -> (x .and. y?=w612:bool)
              }
              frame True {
                w639 = 0.0
                # "If needed, make seperate FOR Loop for \nY only... Using more previous values than X"
                # "New Y"
                # "New X"
                # "Only consider if velocity is\ngreater than certain speed"
                # "Weighted Robot \nCoordinates"
                # "Position\nValid\n(current)"
                n265 = for {
                  N: w637 -> [_]
                  shift-right: [w655] -> w635
                  shift-left: w639 -> [w654]
                  shift-right: [w653] -> w620
                  shift-left: w639 -> [w652]
                  tunnel: w638 -> [w650] mode=indexing
                  tunnel: w636 -> [w648]
                  # "Fetch Last Valid Values\nand Sum"
                  n266 = Index Array(array=w648, index=w650) -> (element=w649:cluster{sgl, sgl})
                  n267 = Unbundle(w649) -> (w651:sgl, w647:sgl)
                  n268 = Add(x=w647, y=w652) -> (x+y=w653:dbl)
                  n269 = Add(x=w651, y=w654) -> (x+y=w655:dbl)
                }
                n270 = Subtract(x=sgl 1.0, y="New Position\nWeight (X coord)") -> (x-y=w634:sgl)
                n271 = Subtract(x=sgl 1.0, y="New Position\nWeight (Y coord)") -> (x-y=w618:sgl)
                n272 = To Single Precision Float(number=w637) -> (single precision float=w626:sgl)
                n273 = Multiply(x=w634, y=w635) -> (x*y=w627:dbl)
                n274 = Multiply(x=w620, y=w618) -> (x*y=w628:dbl)
                n275 = Divide(x=w627, y=w626) -> (x/y=w624:dbl)
                n276 = Divide(x=w628, y=w626) -> (x/y=w625:dbl)
                n277 = Multiply(x="New Position\nWeight (X coord)", y=w632) -> (x*y=w630:dbl)
                n278 = Multiply(x=w619, y="New Position\nWeight (Y coord)") -> (x*y=w629:dbl)
                n279 = Add(x=w630, y=w624) -> (x+y=w623:dbl)
                n280 = Add(x=w629, y=w625) -> (x+y=w622:dbl)
                n281 = Greater Than 0?(x=w637) -> (x > 0?=w645:bool)
                n282 = case shown="True" w645 {
                  tunnel: w623 -> [w660 w667]
                  tunnel: w622 -> [w659 w666]
                  tunnel: w638 -> [_ w679]
                  tunnel: w636 -> [_ w678]
                  tunnel: [w657 w667] -> w644
                  tunnel: [w656 w666] -> w643
                  tunnel: [w661 w668] -> w642
                  tunnel: w641 -> [w663 _]
                  tunnel: w640 -> [w662 _]
                  frame False {
                    w658 = sgl 0.0 ("upper limit")
                    # "Check that within bounds of arena"
                    # "No Pevious is Available to Compare"
                    n283 = In Range and Coerce(upper limit=w663, x=w660, lower limit=w658) -> (In Range?=w665:bool)  [unwired: 1 out]
                    n284 = In Range and Coerce(upper limit=w662, x=w659, lower limit=w658) -> (In Range?=w664:bool)  [unwired: 1 out]
                    n285 = And(x=w665, y=w664) -> (x .and. y?=w661:bool)
                    n286 = Select(t=w660, s=w661, f=w658) -> (s? t:f=w657:dbl)
                    n287 = Select(t=w659, s=w661, f=w658) -> (s? t:f=w656:dbl)
                  }
                  frame True {
                    # "New"
                    # "(Y1 - Y2)^2"
                    # "(X1 - X2)^2"
                    # "Previous"
                    # "Pevious is Available to Compare"
                    n288 = Index Array(array=w679, index=u8 0) -> (element=w681:u8)
                    n289 = Index Array(array=w678, index=w681) -> (element=w680:cluster{sgl, sgl})
                    n290 = Unbundle(w680) -> (w670:sgl, w669:sgl)
                    n291 = Subtract(x=w670, y=w667) -> (x-y=w675:dbl)
                    n292 = Subtract(x=w666, y=w669) -> (x-y=w674:dbl)
                    n293 = Square(x=w675) -> (x^2=w673:dbl)
                    n294 = Square(x=w674) -> (x^2=w672:dbl)
                    n295 = Add(x=w673, y=w672) -> (x+y=w676:dbl)
                    n296 = Square Root(x=w676) -> (sqrt(x)=w671:dbl)
                    n297 = Less Or Equal?(x=w671, y="New Position \nThreshold") -> (x <= y?=w668:bool)
                  }
                }
                n298 = Bundle("upper limit"=w644, "upper limit"=w643) -> (w646:cluster{"upper limit":dbl, "upper limit":dbl})  [unwired: 1 in]
              }
            }
          }
        }
        "Orietnation\n(current)" <- w182
        n299 = And(x=w192, y=w191) -> (x .and. y?=w133:bool)
        "Position Valid" <- w133
        n300 = Exclusive Or(1:w191, 2:w192) -> (0:w190:bool)
        n301 = case shown="True" w133 {
          tunnel: [w738 w741] -> w134
          tunnel: [w739 w740] -> w137
          tunnel: w205 -> [_ w741]
          tunnel: w204 -> [_ w740]
          tunnel: w190 -> [_ _]
          frame False {
            w738 = sgl 0.0 ("f")
            n302 = Bundle("f"=w738, "f"=w738) -> (w739:cluster{"f":sgl, "f":sgl})  [unwired: 1 in]
          }
          frame True {
            # "For Servos"
            "Last Orientation" <- w741
            "Last Position" <- w740
          }
        }
        "Robot Coordinates - Avgd" <- w137
        "Orientation Avgd" <- w134
        n303 = local read "History Size"() -> (w184:u8)
        n304 = Decrement(x=w184) -> (x-1=w185:u8)
        n305 = for {
          N: w184 -> [_]
          shift-right: [w779] -> w207
          shift-left: w203 -> [w778]
          tunnel: w137 -> [w777]
          tunnel: w185 -> [w776]
          i -> [w775]
          n306 = Subtract(x=w776, y=w775) -> (x-y=w774:i32)
          n307 = Equal To 0?(x=w774) -> (x = 0?=w773:bool)
          n308 = case shown="False" w773 {
            tunnel: w774 -> [w781 w786]
            tunnel: w778 -> [w784 w787]
            tunnel: [w782 w788] -> w779
            tunnel: w777 -> [_ w785]
            frame False {
              n309 = Decrement(x=w781) -> (x-1=w780:i32)
              n310 = Index Array(array=w784, index=w780) -> (element=w783:cluster{sgl, sgl})
              n311 = Replace Array Subset(array=w784, new element=w783, index=w781) -> (w782:cluster{sgl, sgl}[])
            }
            frame True {
              n312 = Replace Array Subset(array=w787, new element=w785, index=w786) -> (w788:cluster{sgl, sgl}[])
            }
          }
        }
        n313 = Unbundle(w137) -> ("upper limit"=w136:dbl, "upper limit"=w135:dbl)
        n314 = shared-variable "RT myRIO Target - Overlord\\Localization_Variables_r0.lvlib\\loc_x"(w136) -> ()  [unwired: 1 in, 1 out]
        n315 = shared-variable "RT myRIO Target - Overlord\\Localization_Variables_r0.lvlib\\loc_y"(w135) -> ()  [unwired: 1 in, 1 out]
        n316 = shared-variable "RT myRIO Target - Overlord\\Localization_Variables_r0.lvlib\\loc_theta"(w134) -> ()  [unwired: 1 in, 1 out]
        n317 = shared-variable "RT myRIO Target - Overlord\\Localization_Variables_r0.lvlib\\loc_flag"(w133) -> ()  [unwired: 1 in, 1 out]
        n318 = Decrement(x=w184) -> (x-1=w186:u8)
        n319 = for {
          N: w184 -> [_]
          shift-right: [w763] -> w208
          shift-left: w202 -> [w762]
          tunnel: w134 -> [w761]
          tunnel: w186 -> [w760]
          i -> [w759]
          n320 = Subtract(x=w760, y=w759) -> (x-y=w757:i32)
          n321 = Equal To 0?(x=w757) -> (x = 0?=w758:bool)
          n322 = case shown="False" w758 {
            tunnel: w757 -> [w765 w770]
            tunnel: w762 -> [w768 w771]
            tunnel: [w766 w772] -> w763
            tunnel: w761 -> [_ w769]
            frame False {
              # "Shift"
              n323 = Decrement(x=w765) -> (x-1=w764:i32)
              n324 = Index Array(array=w768, index=w764) -> (element=w767:sgl)
              n325 = Replace Array Subset(array=w768, new element=w767, index=w765) -> (w766:sgl[])
            }
            frame True {
              # "insert new"
              n326 = Replace Array Subset(array=w771, new element=w769, index=w770) -> (w772:sgl[])
            }
          }
        }
        n327 = Decrement(x=w184) -> (x-1=w183:u8)
        n328 = for {
          N: w184 -> [_]
          shift-right: [w748] -> w206
          shift-left: w201 -> [w747]
          tunnel: w133 -> [w746]
          tunnel: w183 -> [w745]
          i -> [w744]
          n329 = Subtract(x=w745, y=w744) -> (x-y=w742:i32)
          n330 = Equal To 0?(x=w742) -> (x = 0?=w743:bool)
          n331 = case shown="False" w743 {
            tunnel: w747 -> [w753 w755]
            tunnel: [w751 w756] -> w748
            tunnel: w746 -> [_ w754]
            tunnel: w742 -> [w749 _]
            frame False {
              n332 = Decrement(x=w749) -> (x-1=w750:i32)
              n333 = Index Array(array=w753, index=w750) -> (element=w752:bool)
              n334 = Replace Array Subset(array=w753, new element=w752, index=w749) -> (w751:bool[])
            }
            frame True {
              n335 = Replace Array Subset(array=w755, new element=w754) -> (w756:bool[])  [unwired: 1 in]
            }
          }
        }
        n336 = Boolean To (0,1)(Boolean=w206) -> (0, 1=w198:i16[])
        n337 = Add Array Elements(numeric array=w198) -> (sum=w196:i16)
        n338 = Greater Or Equal?(x=w196, y=i16 2) -> (x >= y?=→"Position \nLock Status":bool)
        n339 = case shown="True" w133 {
          tunnel: w137 -> [_ w737]
          frame False {
          }
          frame True {
            # "update debug graph\nif current is valid"
            n340 = Unbundle(w737) -> ("upper limit"=w736:dbl, "upper limit"=w735:dbl)
            n341 = Build Array(w735) -> (w733:dbl[])
            n342 = Build Array(w736) -> (w734:dbl[])
            n343 = Bundle(w734, w733) -> (→"Real Position in Course 2":cluster{dbl[], dbl[]})  [unwired: 1 in]
          }
        }
      }
    }
    n344 = case shown="True" w113 {
      tunnel: w112 -> [_ w120]
      frame False {
      }
      frame True {
        n345 = call "Tick Count3"() -> ("Tick Count(uSec)"=w121:u32)
        n346 = Subtract(x=w121, y=w120) -> (x-y=w124:u32)
        n347 = Divide(x=w124, y=u32 1000 ("x")) -> (x/y=→"dT":dbl)
      }
    }
    n348 = call "Tick Count6"() -> ("Tick Count(uSec)"=w110:u32)
    "Robot Coordinates\nHistory" <- w109
    "Orientation\nHistory" <- w114
    "Position Valid\nHistory" <- w115
  }
  n349 = disable-structure shown="Enabled" {
    disable-tunnel: [w791 _] -> _
    disable-tunnel: ["Search Step Size\n(deg)" _] -> _
    frame Enabled {
      n350 = Multiply(x=3.413333333333333, y="Search Step Size\n(deg)") -> (x*y=w789:dbl)
      n351 = To Unsigned Word Integer(number=w789) -> (unsigned 16bit integer=w791:u16)
    }
    frame Disabled {
    }
  }
  n352 = Multiply(x="Move Servo\nThreshold (deg)", y=3.413333333333333) -> (x*y=w18:dbl)
  n353 = To Unsigned Word Integer(number=w18) -> ()  [unwired: 1 out]
  n354 = call "Tick Count8"() -> ()  [unwired: 1 out]
  n355 = flat-sequence {
    tunnel: [w795] -> w42
    tunnel: [w794] -> w41
    tunnel: [w799] -> w40
    tunnel: ["Left Servo\nID"] -> w29
    tunnel: ["Right Servo\nID"] -> w28
    tunnel: ["Compliance Slope"] -> w27
    tunnel: [w839] -> w39
    tunnel: [w838] -> w38
    tunnel: w42 -> [w837]
    tunnel: w41 -> [w836]
    tunnel: w40 -> [w835]
    tunnel: w29 -> [w833]
    tunnel: w28 -> [w832]
    tunnel: w27 -> [w831]
    tunnel: w39 -> [w1112]
    tunnel: w38 -> [w1111]
    frame #0 {
      # "BAUD RATE"
      # "Initialize UART and DIO"
      n356 = call-poly "VISA Configure Serial Port"("VISA resource name"=refnum<visa-resource-name> "ASRL1::INSTR", "Enable Termination\nChar (T)"=FALSE ("Enable Termination\nChar (T)"), "baud rate (9600)"=u32 115200) -> ("VISA resource name out"=w795:refnum<visa-resource-name>)  [unwired: 11 in, 1 out]
      n357 = call <vilib>:"Smart Open.vi"("Channel Names"=tag[] ["A/DIO2"]) -> ("DIO Ref Out"=w794:T7)  [unwired: 9 in, 1 out]
      n358 = flat-sequence {
        tunnel: w795 -> [w807]
        tunnel: w794 -> [w806]
        tunnel: "Left Servo\nID" -> [w808]
        tunnel: [w805] -> w796
        tunnel: "Compliance Slope" -> [w804]
        tunnel: "Right Servo\nID" -> [w821]
        tunnel: w796 -> [w820]
        tunnel: "Compliance Slope" -> [w819]
        tunnel: w795 -> [w818]
        tunnel: w794 -> [w817]
        frame #0 {
          w805 = 3
          n359 = while {
            tunnel: w805 -> [w814]
            tunnel: w807 -> [w812]
            tunnel: w806 -> [w811]
            tunnel: w808 -> [w810]
            tunnel: w804 -> [w809]
            i -> [w815]
            stop <- w813 stop-if-true
            n360 = call "Set_Compliance_Slope_R2.vi"("Compliance Slope"=w809, "DIO Ref Out"=w811, "VISA resource name"=w812, "Servo ID"=w810) -> ()  [unwired: 6 in, 2 out]
            n361 = Increment(x=w815) -> (x+1=w816:i32)
            n362 = Greater Or Equal?(x=w816, y=w814) -> (x >= y?=w813:bool)
          }
        }
        frame #1 {
          n363 = while {
            tunnel: w820 -> [w827]
            tunnel: w821 -> [w825]
            tunnel: w818 -> [w824]
            tunnel: w817 -> [w823]
            tunnel: w819 -> [w822]
            i -> [w828]
            stop <- w826 stop-if-true
            n364 = call "Set_Compliance_Slope_R2.vi"("Compliance Slope"=w822, "DIO Ref Out"=w823, "VISA resource name"=w824, "Servo ID"=w825) -> ()  [unwired: 6 in, 2 out]
            n365 = Increment(x=w828) -> (x+1=w829:i32)
            n366 = Greater Or Equal?(x=w829, y=w827) -> (x >= y?=w826:bool)
          }
        }
      }
      n367 = call "Tick Count"() -> ("Tick Count(uSec)"=w799:u32)
    }
    frame #1 {
      # "Service Count"
      n368 = while {
        shift-right: [w842] -> _
        shift-left: w835 -> [w859]
        tunnel: "Max Write\nTx Attempts" -> [w854]
        tunnel: "Max Read\nTx Attempts" -> [w853]
        shift-right: [w849] -> w839
        shift-left: w837 -> [w852]
        shift-right: [w848] -> w838
        shift-left: w836 -> [w851]
        tunnel: w833 -> [w847]
        tunnel: w832 -> [w846]
        tunnel: w831 -> [w845]
        shift-right: [w843] -> _
        shift-left: u16 0 -> [w844]
        stop <- "close comms" stop-if-true
        # "Loop Timer"
        n369 = local read "SERVO ENABLE"() -> (w841:bool)
        n370 = call "Tick Count2"() -> ("Tick Count(uSec)"=w842:u32)
        n371 = Subtract(x=w842, y=w859) -> (x-y=w858:u32)
        n372 = call "Wait4"("Count(mSec)"="Servo Comm\nLoop Time (ms)") -> ()  [unwired: 1 out]
        n373 = Divide(x=w858, y=u32 1000) -> (x/y=→"dT - Comm Loop":dbl)
        n374 = case shown="True" w841 {
          tunnel: w854 -> [_ w868]
          tunnel: w853 -> [_ w899]
          tunnel: w852 -> [w862 w863]
          tunnel: w851 -> [w861 w892]
          tunnel: [w862 w865] -> w849
          tunnel: [w861 w864] -> w848
          tunnel: w847 -> [_ w871]
          tunnel: w846 -> [_ w870]
          tunnel: w845 -> [_ w869]
          tunnel: w844 -> [_ w867]
          tunnel: [u16 100 w866] -> w843
          frame False {
            # "Restart at same value\nUsed to Periodically update \nCompliance Slope"
          }
          frame True {
            n375 = flat-sequence {
              tunnel: [w905] -> w903
              tunnel: [w906] -> w902
              tunnel: [w904] -> w901
              tunnel: w899 -> [w907]
              tunnel: [w909] -> w890
              tunnel: [w908] -> w888
              tunnel: w863 -> [w909]
              tunnel: w892 -> [w908]
              tunnel: w871 -> [w904]
              tunnel: w903 -> [w927]
              tunnel: w902 -> [w928]
              tunnel: w901 -> [w926]
              tunnel: [w926] -> w900
              tunnel: [w925] -> w893
              tunnel: [w924] -> w891
              tunnel: w890 -> [w924]
              tunnel: [w923] -> w889
              tunnel: w888 -> [w923]
              tunnel: w900 -> [w949]
              tunnel: w868 -> [w948]
              tunnel: w893 -> [w943]
              tunnel: w891 -> [w945]
              tunnel: w889 -> [w944]
              tunnel: [w945] -> w886
              tunnel: [w944] -> w884
              tunnel: [w982] -> w887
              tunnel: w886 -> [w982]
              tunnel: [w981] -> w885
              tunnel: w884 -> [w981]
              tunnel: ["Servo Comm\nWait Time - (ms)"] -> w876
              tunnel: w899 -> [w989]
              tunnel: [w988] -> w898
              tunnel: [w987] -> w897
              tunnel: [w983] -> w895
              tunnel: w887 -> [w986]
              tunnel: w885 -> [w985]
              tunnel: [w986] -> w883
              tunnel: [w985] -> w880
              tunnel: [w984] -> w877
              tunnel: w876 -> [w984]
              tunnel: w870 -> [w983]
              tunnel: w898 -> [w1009]
              tunnel: w897 -> [w1008]
              tunnel: [w1007] -> w896
              tunnel: w895 -> [w1007]
              tunnel: [w1006] -> w894
              tunnel: w883 -> [w1005]
              tunnel: [w1005] -> w882
              tunnel: [w1004] -> w881
              tunnel: w880 -> [w1004]
              tunnel: w877 -> [w1003]
              tunnel: [w1003] -> w875
              tunnel: w896 -> [w1031]
              tunnel: w894 -> [w1029]
              tunnel: w868 -> [w1030]
              tunnel: w882 -> [w1028]
              tunnel: w881 -> [w1027]
              tunnel: [w1028] -> w879
              tunnel: [w1027] -> w878
              tunnel: w875 -> [w1024]
              tunnel: [w1024] -> w874
              tunnel: w879 -> [w1064]
              tunnel: w878 -> [w1063]
              tunnel: w874 -> [w1062]
              tunnel: [w1064] -> w873
              tunnel: [w1063] -> w872
              tunnel: w873 -> [w1068]
              tunnel: w872 -> [w1067]
              tunnel: w871 -> [w1073]
              tunnel: w870 -> [w1072]
              tunnel: w869 -> [w1071]
              tunnel: w867 -> [w1066]
              tunnel: w868 -> [w1070]
              tunnel: [w1069] -> w866
              tunnel: [w1068] -> w865
              tunnel: [w1067] -> w864
              frame #0 {
                n376 = while {
                  tunnel: [w922] -> w905
                  tunnel: w904 -> [w921]
                  tunnel: [w914] -> w906
                  tunnel: w907 -> [w912]
                  tunnel: w909 -> [w911]
                  tunnel: w908 -> [w910]
                  i -> [w913]
                  stop <- w915 stop-if-true
                  # "Attemp to Read Until\nMax Read Tx Attemps Limit"
                  n377 = call "ReadServo_R3.vi"("DIO Ref In"=w910, "VISA resource name out"=w911, "Servo ID"=w921) -> ("Error"=w918:u8, "Valid Checksum"=w919:bool, "Current Position"=w922:u64)  [unwired: 6 in]
                  n378 = Increment(x=w913) -> (x+1=w916:i32)
                  n379 = Equal To 0?(x=w918) -> (x = 0?=w920:bool)
                  n380 = Greater Or Equal?(x=w916, y=w912) -> (x >= y?=w917:bool)
                  n381 = And(x=w919, y=w920) -> (x .and. y?=w914:bool)
                  n382 = Or(x=w914, y=w917) -> (x .or. y?=w915:bool)
                }
              }
              frame #1 {
                # "Read Position First"
                n383 = local read "Servo Goal Position\n - Left"() -> (w925:u16)
                n384 = case shown="True" w928 {
                  tunnel: w927 -> [_ w933]
                  tunnel: w925 -> [_ w931]
                  frame False {
                  }
                  frame True {
                    # "Convert Received Position to Angle Relative to Robot"
                    # "45 DEG MOUNT OFFSET"
                    # "1024/300"
                    n385 = local write "Current L (10bit)"(w933) -> ()
                    n386 = To Word Integer(number=w933) -> (16bit integer=w937:i16)
                    n387 = To Word Integer(number=w931) -> (16bit integer=w936:i16)
                    n388 = Subtract(x=w936, y=w937) -> (x-y=w935:i16)
                    n389 = Divide(x=w933, y=3.413333333333333) -> (x/y=w941:dbl)
                    n390 = Absolute Value(x=w935) -> (abs(x)=w934:i16)
                    n391 = Subtract(x=w941, y=sgl 60.0) -> (x-y=w939:dbl)
                    n392 = Greater?(x=w934, y=u16 5) -> (0:w930:bool)
                    n393 = Add(x=w939, y=sgl 45.0) -> (x+y=w929:dbl)
                    n394 = local write "Move Servo - L"(w930) -> ()
                    n395 = local write "Servo Moving - L"(w930) -> ()
                    n396 = local write "Current Angle\n - Left (internal)"(w929) -> ()
                    n397 = shared-variable "RT myRIO Target - Overlord\\Localization_Variables_r0.lvlib\\Left Servo Angle_Current"(w929) -> ()  [unwired: 1 in, 1 out]
                  }
                }
              }
              frame #2 {
                n398 = local read "Move Servo - L"() -> (w946:bool)
                n399 = case shown="True" w946 {
                  tunnel: w949 -> [_ w964]
                  tunnel: w943 -> [_ w951]
                  tunnel: [TRUE w962] -> w947
                  tunnel: w948 -> [_ w954]
                  tunnel: w945 -> [_ w953]
                  tunnel: w944 -> [_ w952]
                  frame False {
                    # "Only Send if Current Position is far enough"
                  }
                  frame True {
                    w960 = 1
                    # "High Byte"
                    # "Low Byte"
                    n400 = Type Cast(type="", x=w951) -> (*(type *) &x=w961:string)
                    n401 = local write "Servo Moving - L"(TRUE) -> ()
                    n402 = String Subset(string=w961, offset (0)=1, length (rest)=w960) -> (substring=w956:string)
                    n403 = String Subset(string=w961, offset (0)=0, length (rest)=w960) -> (substring=w955:string)
                    n404 = while {
                      tunnel: w964 -> [w978]
                      tunnel: [w970] -> w962
                      tunnel: w956 -> [w974]
                      tunnel: w955 -> [w973]
                      tunnel: w954 -> [w967]
                      tunnel: w953 -> [w966]
                      tunnel: w952 -> [w965]
                      i -> [w968]
                      stop <- w969 stop-if-true
                      # "Attemp to Write Until\nMax Write Tx Attemps Limit"
                      n405 = call "MoveServo_R3.vi"("DIO Ref Out"=w965, "VISA resource name out"=w966, "GP - Low Byte"=w974, "GP - High Byte"=w973, "Servo ID"=w978) -> ("Valid Checksum"=w975:bool, "Error"=w977:u64)  [unwired: 5 in]
                      n406 = Equal To 0?(x=w977) -> (x = 0?=w976:bool)
                      n407 = And(x=w975, y=w976) -> (x .and. y?=w970:bool)
                      n408 = Increment(x=w968) -> (x+1=w972:i32)
                      n409 = Greater Or Equal?(x=w972, y=w967) -> (x >= y?=w971:bool)
                      n410 = Or(x=w970, y=w971) -> (x .or. y?=w969:bool)
                    }
                  }
                }
                n411 = case shown="True" w947 {
                  frame False {
                  }
                  frame True {
                    # "Update Servo flag"
                    n412 = local write "Move Servo - L"(FALSE) -> ()
                  }
                }
              }
              frame #3 {
                n413 = call "Wait2"("Count(mSec)"="Servo Comm\nWait Time - (ms)") -> ()  [unwired: 1 out]
              }
              frame #4 {
                n414 = while {
                  tunnel: [w1002] -> w988
                  tunnel: w983 -> [w1001]
                  tunnel: [w994] -> w987
                  tunnel: w989 -> [w992]
                  tunnel: w986 -> [w991]
                  tunnel: w985 -> [w990]
                  i -> [w993]
                  stop <- w995 stop-if-true
                  # "Attemp to Read Until\nMax Read Tx Attemps Limit"
                  n415 = call "ReadServo_R3.vi"("DIO Ref In"=w990, "VISA resource name out"=w991, "Servo ID"=w1001) -> ("Error"=w998:u8, "Valid Checksum"=w999:bool, "Current Position"=w1002:u64)  [unwired: 6 in]
                  n416 = Increment(x=w993) -> (x+1=w996:i32)
                  n417 = Equal To 0?(x=w998) -> (x = 0?=w1000:bool)
                  n418 = Greater Or Equal?(x=w996, y=w992) -> (x >= y?=w997:bool)
                  n419 = And(x=w999, y=w1000) -> (x .and. y?=w994:bool)
                  n420 = Or(x=w994, y=w997) -> (x .or. y?=w995:bool)
                }
              }
              frame #5 {
                n421 = local read "Servo Goal Position\n - Right"() -> (w1006:u16)
                n422 = case shown="True" w1008 {
                  tunnel: w1009 -> [_ w1013]
                  tunnel: w1006 -> [_ w1012]
                  frame False {
                    # "Don't update current position"
                  }
                  frame True {
                    # "Convert Received Position to Angle Relative to Robot"
                    # "45 DEG MOUNT OFFSET"
                    # "1024/300"
                    n423 = local write "Current R (10bit)"(w1013) -> ()
                    n424 = Divide(x=w1013, y=3.413333333333333) -> (x/y=w1022:dbl)
                    n425 = Subtract(x=w1022, y=sgl 60.0) -> (x-y=w1020:dbl)
                    n426 = Subtract(x=w1020, y=sgl 45.0) -> (x-y=w1010:dbl)
                    n427 = To Word Integer(number=w1012) -> (16bit integer=w1017:i16)
                    n428 = To Word Integer(number=w1013) -> (16bit integer=w1018:i16)
                    n429 = shared-variable "RT myRIO Target - Overlord\\Localization_Variables_r0.lvlib\\Right Servo Angle_Current"(w1010) -> ()  [unwired: 1 in, 1 out]
                    n430 = local write "Current Angle\n - Right (internal)"(w1010) -> ()
                    n431 = Subtract(x=w1017, y=w1018) -> (x-y=w1016:i16)
                    n432 = Absolute Value(x=w1016) -> (abs(x)=w1015:i16)
                    n433 = Greater?(x=w1015, y=u16 5) -> (0:w1011:bool)
                    n434 = local write "Move Servo - R"(w1011) -> ()
                    n435 = local write "Servo Moving - R"(w1011) -> ()
                  }
                }
              }
              frame #6 {
                n436 = local read "Move Servo - R"() -> (w1025:bool)
                n437 = case shown="True" w1025 {
                  tunnel: w1029 -> [_ w1034]
                  tunnel: w1031 -> [_ w1041]
                  tunnel: [TRUE w1042] -> w1026
                  tunnel: w1030 -> [_ w1037]
                  tunnel: w1028 -> [_ w1036]
                  tunnel: w1027 -> [_ w1035]
                  frame False {
                  }
                  frame True {
                    w1044 = 1
                    # "High Byte"
                    # "Low Byte"
                    n438 = Type Cast(type="", x=w1034) -> (*(type *) &x=w1043:string)
                    n439 = local write "Servo Moving - R"(TRUE) -> ()
                    n440 = String Subset(string=w1043, offset (0)=1, length (rest)=w1044) -> (substring=w1040:string)
                    n441 = String Subset(string=w1043, offset (0)=0, length (rest)=w1044) -> (substring=w1039:string)
                    n442 = while {
                      tunnel: [w1053] -> w1042
                      tunnel: w1041 -> [w1058]
                      tunnel: w1040 -> [w1057]
                      tunnel: w1039 -> [w1056]
                      tunnel: w1037 -> [w1051]
                      tunnel: w1036 -> [w1049]
                      tunnel: w1035 -> [w1048]
                      i -> [w1052]
                      stop <- w1050 stop-if-true
                      # "Attemp to Write Until\nMax Write Tx Attemps Limit"
                      n443 = call "MoveServo_R3.vi"("DIO Ref Out"=w1048, "VISA resource name out"=w1049, "GP - Low Byte"=w1057, "GP - High Byte"=w1056, "Servo ID"=w1058) -> ("Valid Checksum"=w1060:bool, "Error"=w1059:u64)  [unwired: 5 in]
                      n444 = Increment(x=w1052) -> (x+1=w1054:i32)
                      n445 = Greater Or Equal?(x=w1054, y=w1051) -> (x >= y?=w1055:bool)
                      n446 = Equal To 0?(x=w1059) -> (x = 0?=w1061:bool)
                      n447 = And(x=w1060, y=w1061) -> (x .and. y?=w1053:bool)
                      n448 = Or(x=w1053, y=w1055) -> (x .or. y?=w1050:bool)
                    }
                  }
                }
                n449 = case shown="True" w1026 {
                  frame False {
                  }
                  frame True {
                    # "Update Servo flag"
                    n450 = local write "Move Servo - R"(FALSE) -> ()
                  }
                }
              }
              frame #7 {
                n451 = call "Wait3"("Count(mSec)"=w1062) -> ()  [unwired: 1 out]
              }
              frame #8 {
                # "Increment Service Count"
                # "Update Compliance Slope\nEvery x loops"
                n452 = Equal?(x=w1066, y=u16 1000) -> (x = y?=w1075:bool)
                n453 = case shown="True" w1075 {
                  tunnel: w1071 -> [_ w1085]
                  tunnel: w1068 -> [_ w1084]
                  tunnel: w1067 -> [_ w1083]
                  tunnel: w1068 -> [_ w1082]
                  tunnel: w1067 -> [_ w1081]
                  tunnel: w1073 -> [_ w1080]
                  tunnel: w1072 -> [_ w1079]
                  tunnel: w1066 -> [w1076 _]
                  tunnel: [w1076 u16 0] -> w1074
                  tunnel: w1070 -> [_ w1077]
                  frame False {
                  }
                  frame True {
                    # "Reset Service\nCount"
                    n454 = flat-sequence {
                      tunnel: w1084 -> [w1090]
                      tunnel: w1083 -> [w1089]
                      tunnel: w1080 -> [w1091]
                      tunnel: [w1087] -> w1086
                      tunnel: w1085 -> [w1088]
                      tunnel: w1077 -> [w1087]
                      tunnel: w1079 -> [w1103]
                      tunnel: w1086 -> [w1102]
                      tunnel: w1085 -> [w1101]
                      tunnel: w1082 -> [w1100]
                      tunnel: w1081 -> [w1099]
                      frame #0 {
                        n455 = while {
                          tunnel: w1087 -> [w1098]
                          tunnel: w1090 -> [w1096]
                          tunnel: w1089 -> [w1095]
                          tunnel: w1091 -> [w1094]
                          tunnel: w1088 -> [w1093]
                          i -> [w1092]
                          stop <- w1097 stop-if-true
                          n456 = call "Set_Compliance_Slope_R2.vi"("Compliance Slope"=w1093, "DIO Ref Out"=w1095, "VISA resource name"=w1096, "Servo ID"=w1094) -> ()  [unwired: 6 in, 2 out]
                          n457 = Greater Or Equal?(x=w1092, y=w1098) -> (x >= y?=w1097:bool)
                        }
                      }
                      frame #1 {
                        n458 = while {
                          tunnel: w1102 -> [w1110]
                          tunnel: w1103 -> [w1108]
                          tunnel: w1100 -> [w1107]
                          tunnel: w1099 -> [w1106]
                          tunnel: w1101 -> [w1105]
                          i -> [w1104]
                          stop <- w1109 stop-if-true
                          n459 = call "Set_Compliance_Slope_R2.vi"("Compliance Slope"=w1105, "DIO Ref Out"=w1106, "VISA resource name"=w1107, "Servo ID"=w1108) -> ()  [unwired: 6 in, 2 out]
                          n460 = Greater Or Equal?(x=w1104, y=w1110) -> (x >= y?=w1109:bool)
                        }
                      }
                    }
                  }
                }
                n461 = Increment(x=w1074) -> (x+1=w1069:u16)
              }
            }
          }
        }
      }
    }
    frame #2 {
      n462 = VISA Close(VISA resource name=w1112) -> ()  [unwired: 1 in, 1 out]
      n463 = call <vilib>:"Close.vi"("DIO Ref In"=w1111) -> ()  [unwired: 10 in, 1 out]
    }
  }
  n464 = while {
    stop <- FALSE stop-if-true
    n465 = call "Wait9"("Count(mSec)"=u32 1000) -> ()  [unwired: 1 out]
  }
  n466 = while {
    shift-right: [w1173] -> _
    shift-left: "Initial Main State - Left" -> [w1198]
    shift-right: [w1165] -> _
    shift-left: "Search Direction - in - L" -> [w1192]
    shift-right: [w1164] -> _
    shift-left: FALSE -> [w1191]
    shift-right: [w1167] -> _
    shift-left: w13 -> [w1166]
    shift-right: [w1168] -> _
    shift-left: w13 -> [w1185]
    shift-right: [w1169] -> _
    shift-left: w13 -> [w1190]
    shift-right: [w1170] -> _
    shift-left: w13 -> [w1184]
    shift-right: [w1171] -> _
    shift-left: w13 -> [w1183]
    shift-right: [w1116] -> _
    shift-left: "Search Direction - in - Right" -> [w1140]
    shift-right: [w1161] -> _
    shift-left: FALSE -> [w1138]
    shift-right: [w1162] -> _
    shift-left: w12 -> [w1129]
    shift-right: [w1117] -> _
    shift-left: w12 -> [w1128]
    shift-right: [w1118] -> _
    shift-left: w12 -> [w1135]
    shift-right: [w1119] -> _
    shift-left: w12 -> [w1137]
    shift-right: [w1120] -> _
    shift-left: w12 -> [w1136]
    shift-right: [w1127] -> _
    shift-left: "Initial Main State- Right" -> [w1152]
    shift-right: [w1157] -> _
    shift-left: 0 -> [w1159]
    shift-right: [w1124] -> _
    shift-left: 0 -> [w1144]
    shift-right: [w1156] -> _
    shift-left: "Initial Tracking State - Left" -> [w1158]
    shift-right: [w1122] -> _
    shift-left: "Initial Tracking State - Right" -> [w1150]
    shift-right: [w1123] -> _
    shift-left: "Initial Recovery State  - Right" -> [w1151]
    shift-right: [w1154] -> _
    shift-left: "Initial Recovery State - L" -> [w1155]
    stop <- FALSE stop-if-true
    w1177 = T2."Tracking" ("Next Main State")
    # "Wait for New"
    # "ADD TRACKING TIMEOUT COUNT**********************"
    # "Service Track Angle Flag"
    # "Add Logic to Have Search Directions\nopposite if Both Searching"
    # "REMOVE LAST GOAL POSITION WITH cURRENT"
    # "Go to Current State"
    # "Add Logic to Have Search Directions\nopposite if Both Searching"
    # "Manuallly Reset\nRespond Var"
    # "Manuallly Reset\nRespond Var"
    # "Update Comm Process Variables"
    # "Both Tracking"
    # "Current delta - L"
    # "delta move sum - R"
    # "delta move sum - L"
    # "Current delta - R"
    # "Service Move Respond Variables"
    n467 = local read "Min Num Frames\nper Search"() -> (w1163:i32)
    n468 = local read "Minimum Delta \nServo Threshold"() -> (w1182:i16)
    n469 = local read "Maximum Move \nServo Threshold"() -> (w1181:i16)
    n470 = local read "Middle Beacon\nCoordinates"() -> (w1130:cluster{"X":sgl, "Y":sgl})
    n471 = local read "Position \nLock Status"() -> (w1189:bool)
    n472 = local read "Position \nLock Status"() -> (w1133:bool)
    n473 = local read "Search Step Size"() -> (w1180:u16)
    n474 = local read "Last Orientation"() -> (w1187:sgl)
    n475 = local read "Last Orientation"() -> (w1131:sgl)
    n476 = local read "Last Position"() -> (w1188:cluster{"X":sgl, "Y":sgl})
    n477 = local read "Last Position"() -> (w1132:cluster{"X":sgl, "Y":sgl})
    n478 = local read "Min Num Frames\nper Search"() -> (w1134:i32)
    n479 = call "Wait"("Count(mSec)"="Servo Algorithm\nCycle Time(ms)") -> ()  [unwired: 1 out]
    n480 = local read "Minimum Delta \nServo Threshold"() -> (w1142:i16)
    n481 = local read "Maximum Move \nServo Threshold"() -> (w1141:i16)
    n482 = local read "Search Step Size"() -> (w1139:u16)
    n483 = local read "New Data  Flag\nRight Servo"() -> (w1147:bool)
    n484 = local read "New Data  Flag\nLeft Servo"() -> (w1153:bool)
    n485 = local read "Image Lock - Right"() -> (w1149:bool)
    n486 = local read "Image Lock - Left"() -> (w1197:bool)
    n487 = local read "Tracking Angle - Right"() -> (w1146:sgl)
    n488 = local read "Tracking Angle - Left"() -> (w1195:sgl)
    n489 = local read "Current R (10bit)"() -> (w1145:u16)
    n490 = local read "Current L (10bit)"() -> (w1194:u16)
    n491 = case shown="True" w1147 {
      tunnel: [w1225 w1263] -> w1115
      tunnel: [w1219 w1262] -> w1126
      tunnel: w1152 -> [w1220 w1261]
      tunnel: w1149 -> [_ w1260]
      tunnel: "Track Angle Valid  - Right" -> [_ w1259]
      tunnel: w1146 -> [_ w1258]
      tunnel: w1145 -> [w1225 w1257]
      tunnel: "Mounting Offset - Right" -> [_ w1256]
      tunnel: w1140 -> [w1216 w1255]
      tunnel: w1138 -> [_ w1254]
      tunnel: w1135 -> [w1217 w1253]
      tunnel: w1133 -> [_ w1252]
      tunnel: w1132 -> [_ w1251]
      tunnel: w1131 -> [_ w1250]
      tunnel: w1130 -> [_ w1249]
      tunnel: w1128 -> [w1215 w1248]
      tunnel: w1137 -> [w1214 w1247]
      tunnel: w1136 -> [w1218 w1246]
      tunnel: w1142 -> [_ w1245]
      tunnel: w1141 -> [_ w1244]
      tunnel: w1139 -> [_ w1243]
      tunnel: [0 w1242] -> w1125
      tunnel: [w1220 w1241] -> w1127
      tunnel: [w1219 w1240] -> w1121
      tunnel: [w1218 w1239] -> w1120
      tunnel: [w1214 w1238] -> w1119
      tunnel: [w1217 w1237] -> w1118
      tunnel: [w1215 w1236] -> w1117
      tunnel: w1129 -> [_ w1235]
      tunnel: [w1216 w1234] -> w1116
      tunnel: w1134 -> [_ w1233]
      tunnel: w1144 -> [w1223 w1232]
      tunnel: w1150 -> [w1222 w1231]
      tunnel: [w1223 w1230] -> w1124
      tunnel: [w1222 w1229] -> w1122
      tunnel: w1151 -> [w1221 w1228]
      tunnel: [w1221 w1227] -> w1123
      frame False {
        w1219 = FALSE
        # "Recovery Mode COunt"
        # "Frames Processed - L"
        # "Recovery Search move Count - L"
        # "Recovery Search Attempt Count- L"
        # "WAITING FOR NEW IMAGE, RETAIN ALL VALUES"
      }
      frame True {
        w1265 = u16 1023
        w1268 = u16 0
        # "New Tracking State"
        # "Tracking Timeout Count"
        # "Next Main State"
        # "Next Recovery State"
        # "Reset Respond"
        # "Search Direction"
        # "Recovery Count"
        # "Recovery Search move Count"
        # "Recovery Search Attempt Count"
        # "Frames Processed"
        # "Apply Floor/Ceiling to Goal Position"
        # "Current move Delta"
        # "Service Track Angle Flag"
        # "Move Servo"
        # "Goal Position"
        # "Go to Current State"
        n492 = case shown="\"Recovery Mode\"" w1261 {
          tunnel: w1257 -> [w1287 w1362 w1539]
          tunnel: w1258 -> [_ w1364 _]
          tunnel: w1243 -> [w1286 _ w1534]
          tunnel: w1255 -> [w1285 w1344 w1528]
          tunnel: [w1284 w1360 w1538] -> w1269
          tunnel: [w1282 w1361 w1537] -> w1262
          tunnel: w1259 -> [w1280 w1355 w1513]
          tunnel: [w1279 w1357 w1524] -> w1241
          tunnel: w1260 -> [w1278 w1356 w1514]
          tunnel: w1256 -> [_ w1365 w1535]
          tunnel: w1245 -> [_ w1363 _]
          tunnel: [w1272 w1359 w1519] -> w1242
          tunnel: w1244 -> [_ w1358 _]
          tunnel: w1253 -> [w1277 _ w1529]
          tunnel: [enum16{"Generic Sweep", "Recovery Search"}."Recovery Search" enum16{"Generic Sweep", "Recovery Search"}."Recovery Search" w1536] -> w1227
          tunnel: w1248 -> [_ _ w1533]
          tunnel: w1228 -> [_ _ w1516]
          tunnel: w1254 -> [_ w1341 w1545]
          tunnel: w1235 -> [_ w1346 w1540]
          tunnel: w1250 -> [_ w1348 w1542]
          tunnel: w1251 -> [_ w1349 w1543]
          tunnel: w1252 -> [_ w1350 w1544]
          tunnel: w1249 -> [_ w1347 w1541]
          tunnel: [FALSE w1343 w1517] -> w1240
          tunnel: w1233 -> [w1276 _ w1527]
          tunnel: [w1272 w1338 w1526] -> w1236
          tunnel: [w1272 w1338 w1532] -> w1239
          tunnel: [w1272 w1338 w1531] -> w1238
          tunnel: [w1275 w1339 w1530] -> w1237
          tunnel: w1247 -> [_ _ w1522]
          tunnel: w1246 -> [_ _ w1521]
          tunnel: [w1273 w1344 w1520] -> w1234
          tunnel: w1232 -> [_ w1354 _]
          tunnel: [w1272 w1345 w1519] -> w1230
          tunnel: w1231 -> [_ w1351 _]
          tunnel: [enum16{"Track", "Reactive Predict", ""}."Track" ("Initial Tracking State - Right") w1342 enum16{"Track", "Reactive Predict", ""}."Track" ("Initial Tracking State - Right")] -> w1229
          frame "Start Up Search", Default {
            w1272 = u16 0
            # "Search Direction"
            # "Wait for 'x' Images to be Processed\nBefore Going to Next Step"
            # "Next Main State"
            # "New Goal Position"
            # "Move Servo"
            # "Choose Next State"
            # "Frames Processed Count"
            n493 = Greater Or Equal?(x=w1277, y=w1276) -> (x >= y?=w1283:bool)
            n494 = case shown="True" w1283 {
              tunnel: w1287 -> [w1300 w1312]
              tunnel: w1286 -> [_ w1310]
              tunnel: w1285 -> [w1299 w1309]
              tunnel: [w1300 w1306] -> w1284
              tunnel: [w1298 0] -> w1275
              tunnel: [FALSE TRUE] -> w1281
              tunnel: w1277 -> [w1301 _]
              tunnel: [w1299 w1303] -> w1273
              frame False {
                # "Increase Frames\nProcessed Count"
                n495 = Increment(x=w1301) -> (x+1=w1298:i32)
              }
              frame True {
                # "Reset Frames\nProcessed Count"
                # "SWEEP SEARCH - Startup"
                # "Multiple New Step\nby Step SIze"
                # "F = CCW\nT = CW"
                # "Last Direction"
                # "Min Step"
                # "add 10 in case\nactual position\nis lower than GP"
                # "Set New Step #"
                # "Choose Direction"
                # "Nearest step"
                # "Adjust Actual Posiiton\n to pre-determiend steps"
                # "Move Servo 1 \"Step\" to\nSearch"
                n496 = Add(x=3, y=w1312) -> (x+y=w1318:i32)
                n497 = Quotient & Remainder(x=w1318, y=w1310) -> (floor(x/y)=w1316:i32)  [unwired: 1 out]
                n498 = To Byte Integer(number=w1316) -> (8bit integer=w1307:i8)
                n499 = Less?(x=w1307, y=1) -> (x < y?=w1313:bool)
                n500 = case shown="False" w1313 {
                  tunnel: w1307 -> [w1329 w1337]
                  tunnel: [w1331 FALSE] -> w1303
                  tunnel: [w1330 w1337] -> w1315
                  tunnel: w1309 -> [w1328 _]
                  tunnel: w1310 -> [w1326 _]
                  frame False {
                    # "Max Step"
                    # "# of steps\nminus 1"
                    n501 = Divide(x=1024, y=w1326) -> (x/y=w1323:dbl)
                    n502 = To Unsigned Byte Integer(number=w1323) -> (unsigned 8bit integer=w1324:u8)
                    n503 = Greater Or Equal?(x=w1329, y=w1324) -> (x >= y?=w1325:bool)
                    n504 = case shown="True" w1325 {
                      tunnel: [w1332 TRUE] -> w1331
                      tunnel: [w1333 w1334] -> w1330
                      tunnel: w1329 -> [w1333 w1334]
                      tunnel: w1328 -> [w1332 _]
                      frame False {
                        # "No Need to\nChange Direction"
                      }
                      frame True {
                        # "T"
                        # "Move CW"
                      }
                    }
                  }
                  frame True {
                    # "F"
                    # "Move CCW"
                  }
                }
                n505 = case shown="False" w1303 {
                  tunnel: w1315 -> [w1320 w1321]
                  tunnel: [w1319 w1322] -> w1311
                  frame False {
                    # "CCW\n+1"
                    n506 = Increment(x=w1320) -> (x+1=w1319:i8)
                  }
                  frame True {
                    # "CW\n-1"
                    n507 = Decrement(x=w1321) -> (x-1=w1322:i8)
                  }
                }
                n508 = Multiply(x=w1311, y=w1310) -> (x*y=w1308:u16)
                n509 = To Unsigned Word Integer(number=w1308) -> (unsigned 16bit integer=w1306:u16)
              }
            }
            n510 = case shown="False" w1280 {
              tunnel: [w1289 FALSE] -> w1282
              tunnel: w1281 -> [w1289 _]
              tunnel: [w1290 w1295] -> w1279
              tunnel: w1278 -> [_ w1293]
              frame False {
                # "********** Tracking Angle Valid - deleted"
                # "Check other Servo\nStay in Startup  State"
                n511 = local read "Image Lock - Left"() -> (w1288:bool)
                n512 = case shown="True" w1288 {
                  tunnel: [T2."Start Up Search" ("Next Main State") T2."Recovery Mode" ("Next Main State")] -> w1290
                  frame False {
                  }
                  frame True {
                  }
                }
              }
              frame True {
                # "Override Move Servo\nCommand bc an Angle Was Found\nduring this Step"
                # "Transition to Tracking State When\nImage Processing has Locked"
                n513 = case shown="False" w1293 {
                  tunnel: [T2."Start Up Search" ("Next Main State") T2."Tracking" ("Next Main State")] -> w1295
                  frame False {
                  }
                  frame True {
                  }
                }
              }
            }
          }
          frame "Tracking" {
            w1338 = 0
            # "Frames Processed Count"
            # "Image Lock - L"
            # "Track Angle Valid"
            # "Tracking Angle"
            # "Tracking Timeout Count"
            # "Max ove delta"
            # "Move delta threshold"
            # "mount offset"
            # "Current Position"
            # "Move Respond"
            # "Trackin Timeout count"
            # "Move Servo"
            # "delta"
            # "GP"
            # "Reset Move Respond"
            # "New Tracking State"
            # "Delta Move Sum"
            # "Choose Next State"
            n514 = case shown="\"Reactive Predict\"" w1351 {
              tunnel: w1365 -> [w1383 _]
              tunnel: w1364 -> [w1382 _]
              tunnel: w1363 -> [w1381 _]
              tunnel: w1362 -> [w1380 w1438]
              tunnel: [w1379 w1436] -> w1361
              tunnel: [w1378 w1444] -> w1360
              tunnel: [w1377 0] -> w1359
              tunnel: w1358 -> [w1376 _]
              tunnel: w1356 -> [w1375 w1428]
              tunnel: w1355 -> [w1374 w1431]
              tunnel: w1354 -> [w1373 w1433]
              tunnel: w1350 -> [_ w1443]
              tunnel: w1349 -> [_ w1442]
              tunnel: w1348 -> [_ w1441]
              tunnel: w1347 -> [_ w1440]
              tunnel: w1341 -> [_ w1439]
              tunnel: w1346 -> [_ w1437]
              tunnel: [TRUE w1434] -> w1343
              tunnel: [w1370 w1432] -> w1345
              tunnel: [w1368 w1430] -> w1342
              tunnel: [0 0] -> w1339
              frame "Track", Default {
                # "Reset"
                # "Tracking Timeout"
                # "Move Delta"
                # "Goal Position"
                # "Tracking Move"
                # "Move Servo"
                # "Only Consider Tracking Angle\n\nIF\n\nImage Locked        == T\nTrack Angle Flag   == T"
                n515 = And(x=w1375, y=w1374) -> (x .and. y?=w1367:bool)
                n516 = case shown="True" w1367 {
                  tunnel: w1383 -> [_ w1389]
                  tunnel: w1382 -> [_ w1407]
                  tunnel: w1381 -> [_ w1404]
                  tunnel: w1380 -> [w1386 w1394]
                  tunnel: [w1386 w1403] -> w1378
                  tunnel: [w1388 w1402] -> w1379
                  tunnel: [w1388 w1401] -> _
                  tunnel: [u16 0 w1400] -> w1377
                  tunnel: w1376 -> [_ w1396]
                  tunnel: w1373 -> [w1385 _]
                  tunnel: [w1384 0] -> w1370
                  frame False {
                    w1388 = FALSE
                    # "Increment timeout"
                    n517 = Increment(x=w1385) -> (x+1=w1384:i32)
                  }
                  frame True {
                    # "Convert Track Angle to UINT16"
                    # "1024/300"
                    # "Move to Tracking Angle \n\nif delta is greater than move servo threshold\nAND less than max move threshold"
                    n518 = Add(x=w1407, y=w1389) -> (x+y=w1410:sgl)
                    n519 = Add(x=w1410, y=sgl 60.0) -> (x+y=w1409:sgl)
                    n520 = Multiply(x=3.413333333333333, y=w1409) -> (x*y=w1390:dbl)
                    n521 = To Word Integer(number=w1394) -> (16bit integer=w1392:i16)
                    n522 = To Unsigned Word Integer(number=w1390) -> (unsigned 16bit integer=w1406:u16)
                    n523 = To Word Integer(number=w1390) -> (16bit integer=w1405:i16)
                    n524 = Subtract(x=w1405, y=w1392) -> (x-y=w1395:i16)
                    n525 = Absolute Value(x=w1395) -> (abs(x)=w1391:i16)
                    n526 = Greater Or Equal?(x=w1391, y=w1404) -> (x >= y?=w1398:bool)
                    n527 = Less Or Equal?(x=w1391, y=w1396) -> (x <= y?=w1397:bool)
                    n528 = And(x=w1398, y=w1397) -> (x .and. y?=w1399:bool)
                    n529 = case shown="True" w1399 {
                      tunnel: w1406 -> [_ w1418]
                      tunnel: [w1413 w1418] -> w1403
                      tunnel: [w1414 w1424] -> w1402
                      tunnel: [w1414 w1424] -> w1401
                      tunnel: w1394 -> [w1413 _]
                      tunnel: w1391 -> [_ w1423]
                      tunnel: [u16 0 w1423] -> w1400
                      tunnel: w1389 -> [_ w1417]
                      frame False {
                        w1414 = FALSE
                        # "Don't Move"
                      }
                      frame True {
                        w1424 = TRUE
                        # "45 DEG MOUNT OFFSET"
                        # "1024/300"
                        # "Current Delta"
                        # "Use new Track Angle"
                        n530 = Divide(x=w1418, y=3.413333333333333) -> (x/y=w1420:dbl)
                        n531 = Negate(x=w1417) -> (-x=w1416:sgl)
                        n532 = Subtract(x=w1420, y=sgl 60.0) -> (x-y=w1422:dbl)
                        n533 = Add(x=w1422, y=w1416) -> (x+y=w1415:dbl)
                        n534 = local write "Last Track Angle - R"(w1415) -> ()
                      }
                    }
                  }
                }
                n535 = local read "Timeout to \nEnable Reactive Predict"() -> (w1371:u16)
                n536 = Less?(x=w1370, y=w1371) -> (x < y?=w1369:bool)
                n537 = case shown="False" w1369 {
                  tunnel: [enum16{"Track", "Reactive Predict", ""}."Reactive Predict" ("Initial Tracking State - Right") enum16{"Track", "Reactive Predict", ""}."Track" ("Initial Tracking State - Right")] -> w1368
                  frame False {
                  }
                  frame True {
                  }
                }
              }
              frame "Reactive Predict" {
                # "Choose New\nTracking State"
                n538 = Or(x=w1428, y=w1431) -> (x .or. y?=w1427:bool)
                n539 = case shown="False" w1427 {
                  tunnel: [w1457 w1509] -> w1444
                  tunnel: w1443 -> [w1456 _]
                  tunnel: w1442 -> [w1455 _]
                  tunnel: w1441 -> [w1454 _]
                  tunnel: w1440 -> [w1453 _]
                  tunnel: w1439 -> [w1452 _]
                  tunnel: w1437 -> [w1451 _]
                  tunnel: [w1450 w1508] -> w1436
                  tunnel: [w1449 w1508] -> w1434
                  tunnel: w1433 -> [w1448 _]
                  tunnel: [w1447 0] -> w1432
                  tunnel: [enum16{"Track", "Reactive Predict", ""}."Reactive Predict" ("Initial Tracking State - Right") enum16{"Track", "Reactive Predict", ""}."Track" ("Initial Tracking State - Right")] -> w1430
                  tunnel: w1438 -> [w1445 w1509]
                  frame False {
                    # "Stay in Reactive State"
                    # "Increment Track Timeout"
                    # "Move Respond Flag"
                    n540 = Increment(x=w1448) -> (x+1=w1447:i32)
                    n541 = case shown="True" w1452 {
                      tunnel: w1456 -> [_ w1472]
                      tunnel: w1455 -> [_ w1471]
                      tunnel: w1454 -> [_ w1470]
                      tunnel: w1453 -> [_ w1469]
                      tunnel: w1451 -> [_ w1466]
                      tunnel: [w1458 w1462] -> w1457
                      tunnel: [w1459 w1461] -> w1450
                      tunnel: [w1459 w1461] -> w1449
                      tunnel: w1445 -> [w1458 w1460]
                      frame False {
                        w1459 = FALSE
                        # "Reset Move Respond = F"
                        # "Move Servo = F"
                      }
                      frame True {
                        w1461 = TRUE
                        # "Position Lock"
                        # "Current Servo\nPosition"
                        # "Reset Move\nRespond = T"
                        # "Move Servo = T"
                        # "Apply Direction \nto Offset (delta sum)"
                        # "Check Last Known Position of Robot"
                        n542 = case shown="True" w1472 {
                          tunnel: w1471 -> [_ w1500]
                          tunnel: w1470 -> [_ w1475]
                          tunnel: w1469 -> [_ w1476]
                          tunnel: [sgl 1.0 ("y") w1474] -> w1468
                          frame False {
                            # "No Position Data Available"
                            # "Default is to move\nSame Direction as other\nServo"
                          }
                          frame True {
                            w1481 = sgl 1.0 ("y")
                            # "Use previous position/orientation to Guess Which Direction to Move Servo"
                            # "Choose Search Direction"
                            # "\"Perpendicular \nThreshold\""
                            # "If Orientation is\n ~Perpendicular -> Start Search\n in Opposite Direction of Other"
                            # "****add 90 until orientation angle is fixed"
                            # "Last Orientation"
                            # "Convert to Rad"
                            # "Avoid Divide by 0"
                            # "-1/m"
                            # "Calculate Normal Line to \nLast Robot Position\nfrom Center Beacon"
                            # "last Position \nCoordinates"
                            n543 = Unbundle(w1500) -> ("X"=w1480:sgl, "Y"=w1479:sgl)
                            n544 = Unbundle(w1476) -> ("X"=w1478:sgl, "Y"=w1477:sgl)
                            n545 = Subtract(x=w1479, y=w1477) -> (x-y=w1496:sgl)
                            n546 = Subtract(x=w1480, y=w1478) -> (x-y=w1494:sgl)
                            n547 = Equal To 0?(x=w1494) -> (x = 0?=w1495:bool)
                            n548 = case shown="False" w1495 {
                              tunnel: w1496 -> [w1503 _]
                              tunnel: w1494 -> [w1502 _]
                              tunnel: [w1501 1000000000000000.0] -> w1493
                              frame False {
                                n549 = Divide(x=w1503, y=w1502) -> (x/y=w1501:sgl)
                              }
                              frame True {
                              }
                            }
                            n550 = Equal To 0?(x=w1493) -> (x = 0?=w1498:bool)
                            n551 = case shown="False" w1498 {
                              tunnel: [w1505 1e-08] -> w1497
                              tunnel: w1493 -> [w1505 _]
                              frame False {
                              }
                              frame True {
                                # "Can't have infinit slope"
                              }
                            }
                            n552 = Divide(x=-1.0, y=w1497) -> (x/y=w1492:dbl)
                            n553 = Inverse Tangent(1:w1492) -> (0:w1490:dbl)
                            n554 = expression code="(x/pi)*180.0" "radians to degrees"(w1490) -> (w1491:dbl)
                            n555 = To Single Precision Float(number=w1491) -> (single precision float=w1488:sgl)
                            n556 = Add(x=w1475, y=sgl 90.0) -> (x+y=w1487:sgl)
                            n557 = Subtract(x=w1488, y=w1487) -> (x-y=w1486:sgl)
                            n558 = Absolute Value(x=w1486) -> (abs(x)=w1485:sgl)
                            n559 = Less Or Equal?(x=w1485, y=sgl 10.0) -> (x <= y?=w1483:bool)
                            n560 = Negate(x=w1481) -> (-x=w1482:sgl)
                            n561 = Select(t=w1482, s=w1483, f=w1481) -> (s? t:f=w1474:sgl)
                          }
                        }
                        n562 = To Word Integer(number=w1468) -> (16bit integer=w1467:i16)
                        n563 = Multiply(x=w1467, y=w1466) -> (x*y=w1465:i32)
                        n564 = To Word Integer(number=w1460) -> (16bit integer=w1464:i16)
                        n565 = Add(x=w1465, y=w1464) -> (x+y=w1463:i32)
                        n566 = To Unsigned Word Integer(number=w1463) -> (unsigned 16bit integer=w1462:u16)
                      }
                    }
                  }
                  frame True {
                    w1508 = TRUE
                    # "Go Directly to Track State"
                  }
                }
              }
            }
            n567 = local read "Tracking Timeout\nThreshold"() -> (w1352:i32)
            n568 = Less?(x=w1345, y=w1352) -> (x < y?=w1353:bool)
            n569 = case shown="False" w1353 {
              tunnel: [T2."Recovery Mode" ("Next Main State") T2."Tracking" ("Next Main State")] -> w1357
              frame False {
              }
              frame True {
              }
            }
          }
          frame "Recovery Mode" {
            w1519 = u16 0
            # "Increment Recovery Mode Count"
            # "Recovvery Mode\nCount"
            # "Frames Processed"
            # "Choose Next Main State"
            # "Reset recovery count"
            # "Recovery move\nCount"
            # "Recovery Search\nAttempt count"
            # "Move Servo = T"
            # "delta move sum"
            # "Robot Position Valid"
            n570 = local read "Image Lock - Left"() -> (w1523:bool)
            n571 = case shown="\"Recovery Search\"" w1516 {
              tunnel: w1545 -> [_ _]
              tunnel: w1544 -> [_ _]
              tunnel: w1543 -> [_ _]
              tunnel: w1542 -> [_ _]
              tunnel: w1541 -> [_ _]
              tunnel: w1540 -> [_ _]
              tunnel: w1539 -> [w1573 w1659]
              tunnel: [w1565 w1657] -> w1538
              tunnel: [w1562 w1651] -> w1537
              tunnel: [FALSE FALSE] -> w1517
              tunnel: [w1567 w1648] -> w1536
              tunnel: w1533 -> [w1571 _]
              tunnel: w1535 -> [w1574 _]
              tunnel: w1534 -> [w1572 w1654]
              tunnel: [w1564 w1647] -> w1531
              tunnel: [w1563 w1647] -> w1532
              tunnel: w1523 -> [w1561 _]
              tunnel: [w1552 w1658] -> w1530
              tunnel: w1529 -> [w1550 w1642]
              tunnel: w1528 -> [w1555 w1655]
              tunnel: w1527 -> [w1551 w1653]
              tunnel: w1514 -> [_ _]
              tunnel: w1513 -> [_ w1650]
              tunnel: [FALSE w1649] -> w1525
              tunnel: w1522 -> [w1559 _]
              tunnel: w1521 -> [w1558 _]
              tunnel: [w1555 w1646] -> w1520
              frame "Recovery Search" {
                # "Wait for 2 Images to be Processed\nBefore Going to Next Step"
                # "Choose Next Reovery State"
                # "Recovery Search \nAttempt Count"
                # "Move Servo"
                # "Goal Position"
                # "Recovery Search\nmove Count"
                # "Attempt Recovery Search if Other Servo has Valid Angle"
                n572 = local read "Last Track Angle - L"() -> (w1554:sgl)
                n573 = Greater Or Equal?(x=w1550, y=w1551) -> (x >= y?=w1553:bool)
                n574 = case shown="True" w1553 {
                  tunnel: w1574 -> [_ w1594]
                  tunnel: [w1579 w1593] -> w1563
                  tunnel: w1573 -> [w1582 w1592]
                  tunnel: w1572 -> [_ w1591]
                  tunnel: [w1580 w1590] -> w1564
                  tunnel: [w1582 w1589] -> w1565
                  tunnel: [FALSE w1588] -> w1562
                  tunnel: w1559 -> [w1580 w1587]
                  tunnel: w1558 -> [w1579 w1586]
                  tunnel: w1561 -> [_ w1585]
                  tunnel: w1554 -> [_ w1584]
                  tunnel: [w1577 0 ("Frames Processed\nCount - in")] -> w1552
                  tunnel: w1550 -> [w1578 _]
                  frame False {
                    # "Increment Frames Processed"
                    # "WAIT"
                    n575 = Increment(x=w1578) -> (x+1=w1577:i32)
                  }
                  frame True {
                    n576 = case shown="True" w1585 {
                      tunnel: w1584 -> [_ w1607]
                      tunnel: w1587 -> [w1595 w1603]
                      tunnel: w1594 -> [_ w1608]
                      tunnel: [w1598 w1606] -> w1589
                      tunnel: [w1596 w1605] -> w1593
                      tunnel: w1586 -> [w1596 w1604]
                      tunnel: w1592 -> [w1598 w1602]
                      tunnel: w1591 -> [_ w1601]
                      tunnel: [FALSE TRUE] -> w1588
                      tunnel: [w1595 w1599] -> w1590
                      frame False {
                        # "Don't Move bc Other Servo Doesn't Have Image Lock"
                      }
                      frame True {
                        # "Move Servo = T"
                        n577 = Greater Than 0?(x=w1603) -> (x > 0?=w1609:bool)
                        n578 = case shown="False" w1609 {
                          tunnel: w1608 -> [w1616 _]
                          tunnel: w1607 -> [w1610 _]
                          tunnel: [w1615 w1626] -> w1606
                          tunnel: [w1613 w1632] -> w1605
                          tunnel: w1604 -> [w1614 w1632]
                          tunnel: w1603 -> [w1612 w1629]
                          tunnel: [w1611 w1631] -> w1599
                          tunnel: w1602 -> [_ w1627]
                          tunnel: w1601 -> [_ w1624]
                          frame False {
                            # "Increment move count to transition\nto Pan mode"
                            # "Increment Recovery Search Attempt Count"
                            # "1024/300"
                            # "Move Parallel to Other Servo"
                            n579 = Increment(x=w1614) -> (x+1=w1613:i32)
                            n580 = Add(x=w1610, y=w1616) -> (x+y=w1622:sgl)
                            n581 = Add(x=w1622, y=sgl 60.0) -> (x+y=w1621:sgl)
                            n582 = Multiply(x=3.413333333333333, y=w1621) -> (x*y=w1619:dbl)
                            n583 = Add(x=0.5, y=w1619) -> (x+y=w1617:dbl)
                            n584 = To Unsigned Word Integer(number=w1617) -> (unsigned 16bit integer=w1615:u16)
                            n585 = Increment(x=w1612) -> (x+1=w1611:i32)
                          }
                          frame True {
                            # "Apply Direction"
                            # "Step SIze"
                            # "Current Position"
                            # "Attempt to Pan in Steps Towards other Servo"
                            # "Could be same or function of \nregular search step size"
                            # "Max # of Pan\nMoves"
                            # "Pan Towards Other Servo"
                            n586 = Greater Or Equal?(x=w1629, y=u16 20) -> (x >= y?=w1630:bool)
                            n587 = case shown="False" w1630 {
                              tunnel: w1629 -> [w1640 _]
                              tunnel: [w1639 u16 0] -> w1631
                              frame False {
                                # "Increment Pan Count"
                                n588 = Increment(x=w1640) -> (x+1=w1639:i32)
                              }
                              frame True {
                                # "Reset move count"
                              }
                            }
                            n589 = local read "Recovery Search\nDirection - R"() -> (w1625:bool)
                            n590 = case shown="False" w1625 {
                              tunnel: w1627 -> [w1634 w1638]
                              tunnel: w1624 -> [w1635 w1637]
                              tunnel: [w1633 w1636] -> w1626
                              frame False {
                                # "CCW"
                                n591 = Add(x=w1634, y=w1635) -> (x+y=w1633:u16)
                              }
                              frame True {
                                # "CW"
                                n592 = Subtract(x=w1638, y=w1637) -> (x-y=w1636:u16)
                              }
                            }
                          }
                        }
                      }
                    }
                  }
                }
                n593 = local read "Max Recovery Count\n(Recovery Search)"() -> (w1556:u16)
                n594 = local read "Max Recovery\nSearch Attempts"() -> (w1557:u16)
                n595 = Less Or Equal?(x=w1563, y=w1557) -> (x <= y?=w1569:bool)
                n596 = Less Or Equal?(x=w1571, y=w1556) -> (x <= y?=w1570:bool)
                n597 = And(x=w1569, y=w1570) -> (x .and. y?=w1568:bool)
                n598 = case shown="True" w1568 {
                  tunnel: [enum16{"Generic Sweep", "Recovery Search"}."Generic Sweep" enum16{"Generic Sweep", "Recovery Search"}."Recovery Search"] -> w1567
                  frame False {
                  }
                  frame True {
                  }
                }
              }
              frame "Generic Sweep" {
                w1647 = u16 0
                # "Angle Valid?"
                # "Choose Next Recovery State"
                # "Wait for 2 Images to be Processed\nBefore Going to Next Step"
                # "New Goal Position"
                # "Move Servo"
                # "Frames Processed Count"
                n599 = Greater Or Equal?(x=w1642, y=w1653) -> (x >= y?=w1660:bool)
                n600 = case shown="True" w1660 {
                  tunnel: w1659 -> [w1676 w1688]
                  tunnel: w1654 -> [_ w1686]
                  tunnel: w1655 -> [w1675 w1685]
                  tunnel: [w1676 w1682] -> w1657
                  tunnel: [w1674 0] -> w1658
                  tunnel: [FALSE TRUE] -> w1652
                  tunnel: w1642 -> [w1677 _]
                  tunnel: [w1675 w1679] -> w1646
                  frame False {
                    # "Increment Frames Processed"
                    n601 = Increment(x=w1677) -> (x+1=w1674:i32)
                  }
                  frame True {
                    # "Reset Frames\nProcessed Count"
                    # "SWEEP SEARCH - Startup"
                    # "Multiple New Step\nby Step SIze"
                    # "F = CCW\nT = CW"
                    # "Last Direction"
                    # "Min Step"
                    # "add 10 in case\nactual position\nis lower than GP"
                    # "Set New Step #"
                    # "Choose Direction"
                    # "Nearest step"
                    # "Adjust Actual Posiiton\n to pre-determiend steps"
                    # "Move Servo 1 \"Step\" to\nSearch"
                    n602 = Add(x=5, y=w1688) -> (x+y=w1694:i32)
                    n603 = Quotient & Remainder(x=w1694, y=w1686) -> (floor(x/y)=w1692:i32)  [unwired: 1 out]
                    n604 = To Byte Integer(number=w1692) -> (8bit integer=w1683:i8)
                    n605 = Less?(x=w1683, y=1) -> (x < y?=w1689:bool)
                    n606 = case shown="False" w1689 {
                      tunnel: w1683 -> [w1705 w1713]
                      tunnel: [w1707 FALSE] -> w1679
                      tunnel: [w1706 w1713] -> w1691
                      tunnel: w1685 -> [w1704 _]
                      tunnel: w1686 -> [w1702 _]
                      frame False {
                        # "Max Step"
                        # "# of steps\nminus 1"
                        n607 = Divide(x=1024, y=w1702) -> (x/y=w1699:dbl)
                        n608 = To Unsigned Byte Integer(number=w1699) -> (unsigned 8bit integer=w1700:u8)
                        n609 = Greater Or Equal?(x=w1705, y=w1700) -> (x >= y?=w1701:bool)
                        n610 = case shown="True" w1701 {
                          tunnel: [w1708 TRUE] -> w1707
                          tunnel: [w1709 w1710] -> w1706
                          tunnel: w1705 -> [w1709 w1710]
                          tunnel: w1704 -> [w1708 _]
                          frame False {
                            # "No Need to\nChange Direction"
                          }
                          frame True {
                            # "T"
                            # "Move CW"
                          }
                        }
                      }
                      frame True {
                        # "F"
                        # "Move CCW"
                      }
                    }
                    n611 = case shown="True" w1679 {
                      tunnel: w1691 -> [w1696 w1697]
                      tunnel: [w1695 w1698] -> w1687
                      frame False {
                        # "CCW\n+1"
                        n612 = Increment(x=w1696) -> (x+1=w1695:i8)
                      }
                      frame True {
                        # "CW\n-1"
                        n613 = Decrement(x=w1697) -> (x-1=w1698:i8)
                      }
                    }
                    n614 = Multiply(x=w1687, y=w1686) -> (x*y=w1684:u16)
                    n615 = To Unsigned Word Integer(number=w1684) -> (unsigned 16bit integer=w1682:u16)
                  }
                }
                n616 = local read "Track Angle Valid - Left"() -> (w1645:bool)
                n617 = local read "Image Lock - Left"() -> (w1644:bool)
                n618 = Or(x=w1644, y=w1645) -> (x .or. y?=w1643:bool)
                n619 = case shown="False" w1650 {
                  tunnel: [w1663 w1673] -> w1651
                  tunnel: w1652 -> [w1664 _]
                  tunnel: [w1665 enum16{"Generic Sweep", "Recovery Search"}."Generic Sweep"] -> w1648
                  tunnel: [w1662 w1673] -> w1649
                  tunnel: w1643 -> [w1661 _]
                  frame False {
                    # "Is other servo tracking?"
                    n620 = case shown="True" w1661 {
                      tunnel: [enum16{"Generic Sweep", "Recovery Search"}."Generic Sweep" enum16{"Generic Sweep", "Recovery Search"}."Recovery Search"] -> w1665
                      tunnel: w1664 -> [w1668 _]
                      tunnel: [w1668 FALSE] -> w1663
                      tunnel: [FALSE TRUE] -> w1662
                      frame False {
                        # "Stay in Sweep"
                      }
                      frame True {
                        # "G o to Recovery Search  State"
                      }
                    }
                  }
                  frame True {
                    w1673 = FALSE
                    # "Override Move Servo\nCommand bc an Angle Was Found\nduring this Step"
                    # "Stay In Sweep\nLet Main State Machine transition\ninto Tracking"
                  }
                }
              }
            }
            n621 = Increment(x=w1533) -> (x+1=w1515:i32)
            n622 = case shown="True" w1525 {
              tunnel: w1515 -> [w1548 _]
              tunnel: [w1548 0] -> w1526
              frame False {
              }
              frame True {
              }
            }
            n623 = case shown="False" w1514 {
              tunnel: [T2."Recovery Mode" ("Next Main State") T2."Tracking" ("Next Main State")] -> w1524
              frame False {
              }
              frame True {
              }
            }
          }
        }
        "Current Move Delta - L 2" <- w1242
        n624 = Less?(x=w1269, y=w1268) -> (x < y?=w1267:bool)
        n625 = local write "New Data  Flag\nRight Servo"(FALSE) -> ()
        n626 = Select(t=w1268, s=w1267, f=w1269) -> (s? t:f=w1264:u16)
        n627 = Greater?(x=w1264, y=w1265) -> (0:w1266:bool)
        n628 = Select(t=w1265, s=w1266, f=w1264) -> (s? t:f=w1263:u16)
      }
    }
    "Next Main State - Right" <- w1127
    "Next Tracking State - Right" <- w1122
    "Next Recovery State - Right" <- w1123
    n629 = case shown="True" w1153 {
      tunnel: [w1725 w1763] -> w1200
      tunnel: [w1719 w1762] -> w1199
      tunnel: w1198 -> [w1720 w1761]
      tunnel: w1197 -> [_ w1760]
      tunnel: "Track Angle Valid - Left" -> [_ w1759]
      tunnel: w1195 -> [_ w1758]
      tunnel: w1194 -> [w1725 w1757]
      tunnel: "Mounting Offset - Left" -> [_ w1756]
      tunnel: w1192 -> [w1716 w1755]
      tunnel: w1191 -> [_ w1754]
      tunnel: w1190 -> [w1717 w1753]
      tunnel: w1189 -> [_ w1752]
      tunnel: w1188 -> [_ w1751]
      tunnel: w1187 -> [_ w1750]
      tunnel: "Middle Beacon\nCoordinates" -> [_ w1749]
      tunnel: w1185 -> [w1715 w1748]
      tunnel: w1184 -> [w1714 w1747]
      tunnel: w1183 -> [w1718 w1746]
      tunnel: w1182 -> [_ w1745]
      tunnel: w1181 -> [_ w1744]
      tunnel: w1180 -> [_ w1743]
      tunnel: [0 w1742] -> w1174
      tunnel: [w1720 w1741] -> w1173
      tunnel: [w1719 w1740] -> w1172
      tunnel: [w1718 w1739] -> w1171
      tunnel: [w1714 w1738] -> w1170
      tunnel: [w1717 w1737] -> w1169
      tunnel: [w1715 w1736] -> w1168
      tunnel: w1166 -> [_ w1735]
      tunnel: [w1716 w1734] -> w1165
      tunnel: w1163 -> [_ w1733]
      tunnel: w1159 -> [w1723 w1732]
      tunnel: w1158 -> [w1722 w1731]
      tunnel: [w1723 w1730] -> w1157
      tunnel: [w1722 w1729] -> w1156
      tunnel: w1155 -> [w1721 w1728]
      tunnel: [w1721 w1727] -> w1154
      frame False {
        w1719 = FALSE
        # "Recovery Mode COunt"
        # "Frames Processed - L"
        # "Recovery Search move Count - L"
        # "Recovery Search Attempt Count- L"
        # "WAITING FOR NEW IMAGE, RETAIN ALL VALUES"
      }
      frame True {
        w1765 = u16 1023
        w1768 = u16 0
        # "New Tracking State"
        # "Tracking Timeout Count"
        # "Next Main State"
        # "Next Recovery State"
        # "Reset Respond"
        # "Search Direction"
        # "Recovery Count"
        # "Recovery Search move Count"
        # "Recovery Search Attempt Count"
        # "Frames Processed"
        # "Apply Floor/Ceiling to Goal Position"
        # "Current move Delta"
        # "Service Track Angle Flag"
        # "Move Servo"
        # "Goal Position"
        # "Go to Current State"
        n630 = case shown="\"Recovery Mode\"" w1761 {
          tunnel: w1757 -> [w1787 w1862 w2040]
          tunnel: w1758 -> [_ w1864 _]
          tunnel: w1743 -> [w1786 _ w2035]
          tunnel: w1755 -> [w1785 w1844 w2029]
          tunnel: [w1784 w1860 w2039] -> w1769
          tunnel: [w1782 w1861 w2038] -> w1762
          tunnel: w1759 -> [w1780 w1855 w2016]
          tunnel: [w1779 w1857 w2025] -> w1741
          tunnel: w1760 -> [w1778 w1856 w2014]
          tunnel: w1756 -> [_ w1865 w2036]
          tunnel: w1745 -> [_ w1863 _]
          tunnel: [w1772 w1859 w2020] -> w1742
          tunnel: w1744 -> [_ w1858 _]
          tunnel: w1753 -> [w1777 _ w2030]
          tunnel: [enum16{"Generic Sweep", "Recovery Search"}."Recovery Search" enum16{"Generic Sweep", "Recovery Search"}."Recovery Search" w2037] -> w1727
          tunnel: w1748 -> [_ _ w2034]
          tunnel: w1728 -> [_ _ w2017]
          tunnel: w1754 -> [_ w1841 w2046]
          tunnel: w1735 -> [_ w1846 w2041]
          tunnel: w1750 -> [_ w1848 w2043]
          tunnel: w1751 -> [_ w1849 w2044]
          tunnel: w1752 -> [_ w1850 w2045]
          tunnel: w1749 -> [_ w1847 w2042]
          tunnel: [FALSE w1843 w2018] -> w1740
          tunnel: w1733 -> [w1776 _ w2028]
          tunnel: [w1772 w1838 w2027] -> w1736
          tunnel: [w1772 w1838 w2033] -> w1739
          tunnel: [w1772 w1838 w2032] -> w1738
          tunnel: [w1775 w1839 w2031] -> w1737
          tunnel: w1747 -> [_ _ w2023]
          tunnel: w1746 -> [_ _ w2022]
          tunnel: [w1773 w1844 w2021] -> w1734
          tunnel: w1732 -> [_ w1854 _]
          tunnel: [w1772 w1845 w2020] -> w1730
          tunnel: w1731 -> [_ w1851 _]
          tunnel: [enum16{"Track", "Reactive Predict", ""}."Track" ("Initial Tracking State - Right") w1842 enum16{"Track", "Reactive Predict", ""}."Track" ("Initial Tracking State - Right")] -> w1729
          frame "Start Up Search", Default {
            w1772 = u16 0
            # "Search Direction"
            # "Wait for 'x' Images to be Processed\nBefore Going to Next Step"
            # "Next Main State"
            # "New Goal Position"
            # "Move Servo"
            # "Choose Next State"
            # "Frames Processed Count"
            n631 = Greater Or Equal?(x=w1777, y=w1776) -> (x >= y?=w1783:bool)
            n632 = case shown="True" w1783 {
              tunnel: w1787 -> [w1800 w1812]
              tunnel: w1786 -> [_ w1810]
              tunnel: w1785 -> [w1799 w1809]
              tunnel: [w1800 w1806] -> w1784
              tunnel: [w1798 0] -> w1775
              tunnel: [FALSE TRUE] -> w1781
              tunnel: w1777 -> [w1801 _]
              tunnel: [w1799 w1803] -> w1773
              frame False {
                # "Increase Frames\nProcessed Count"
                n633 = Increment(x=w1801) -> (x+1=w1798:i32)
              }
              frame True {
                # "Reset Frames\nProcessed Count"
                # "SWEEP SEARCH - Startup"
                # "Multiple New Step\nby Step SIze"
                # "F = CCW\nT = CW"
                # "Last Direction"
                # "Min Step"
                # "add 10 in case\nactual position\nis lower than GP"
                # "Set New Step #"
                # "Choose Direction"
                # "Nearest step"
                # "Adjust Actual Posiiton\n to pre-determiend steps"
                # "Move Servo 1 \"Step\" to\nSearch"
                n634 = Add(x=3, y=w1812) -> (x+y=w1818:i32)
                n635 = Quotient & Remainder(x=w1818, y=w1810) -> (floor(x/y)=w1816:i32)  [unwired: 1 out]
                n636 = To Byte Integer(number=w1816) -> (8bit integer=w1807:i8)
                n637 = Less?(x=w1807, y=1) -> (x < y?=w1813:bool)
                n638 = case shown="False" w1813 {
                  tunnel: w1807 -> [w1829 w1837]
                  tunnel: [w1831 FALSE] -> w1803
                  tunnel: [w1830 w1837] -> w1815
                  tunnel: w1809 -> [w1828 _]
                  tunnel: w1810 -> [w1826 _]
                  frame False {
                    # "Max Step"
                    # "# of steps\nminus 1"
                    n639 = Divide(x=1024, y=w1826) -> (x/y=w1823:dbl)
                    n640 = To Unsigned Byte Integer(number=w1823) -> (unsigned 8bit integer=w1824:u8)
                    n641 = Greater Or Equal?(x=w1829, y=w1824) -> (x >= y?=w1825:bool)
                    n642 = case shown="True" w1825 {
                      tunnel: [w1832 TRUE] -> w1831
                      tunnel: [w1833 w1834] -> w1830
                      tunnel: w1829 -> [w1833 w1834]
                      tunnel: w1828 -> [w1832 _]
                      frame False {
                        # "No Need to\nChange Direction"
                      }
                      frame True {
                        # "T"
                        # "Move CW"
                      }
                    }
                  }
                  frame True {
                    # "F"
                    # "Move CCW"
                  }
                }
                n643 = case shown="False" w1803 {
                  tunnel: w1815 -> [w1820 w1821]
                  tunnel: [w1819 w1822] -> w1811
                  frame False {
                    # "CCW\n+1"
                    n644 = Increment(x=w1820) -> (x+1=w1819:i8)
                  }
                  frame True {
                    # "CW\n-1"
                    n645 = Decrement(x=w1821) -> (x-1=w1822:i8)
                  }
                }
                n646 = Multiply(x=w1811, y=w1810) -> (x*y=w1808:u16)
                n647 = To Unsigned Word Integer(number=w1808) -> (unsigned 16bit integer=w1806:u16)
              }
            }
            n648 = case shown="False" w1780 {
              tunnel: [w1789 FALSE] -> w1782
              tunnel: w1781 -> [w1789 _]
              tunnel: [w1790 w1795] -> w1779
              tunnel: w1778 -> [_ w1793]
              frame False {
                # "Check other Servo\nStay in Startup  State"
                n649 = local read "Image Lock - Right"() -> (w1788:bool)
                n650 = case shown="False" w1788 {
                  tunnel: [T2."Start Up Search" ("Next Main State") T2."Recovery Mode" ("Next Main State")] -> w1790
                  frame False {
                  }
                  frame True {
                  }
                }
              }
              frame True {
                # "Override Move Servo\nCommand bc an Angle Was Found\nduring this Step"
                # "Transition to Tracking State When\nImage Processing has Locked"
                n651 = case shown="True" w1793 {
                  tunnel: [T2."Start Up Search" ("Next Main State") T2."Tracking" ("Next Main State")] -> w1795
                  frame False {
                  }
                  frame True {
                  }
                }
              }
            }
          }
          frame "Tracking" {
            w1838 = 0
            # "Frames Processed Count"
            # "Image Lock - L"
            # "Track Angle Valid"
            # "Tracking Angle"
            # "Tracking Timeout Count"
            # "Max ove delta"
            # "Move delta threshold"
            # "mount offset"
            # "Current Position"
            # "Move Respond"
            # "Trackin Timeout count"
            # "Move Servo"
            # "delta"
            # "GP"
            # "Reset Move Respond"
            # "New Tracking State"
            # "Delta Move Sum"
            # "Choose Next State"
            n652 = case shown="\"Track\", Default" w1851 {
              tunnel: w1865 -> [w1883 _]
              tunnel: w1864 -> [w1882 _]
              tunnel: w1863 -> [w1881 _]
              tunnel: w1862 -> [w1880 w1939]
              tunnel: [w1879 w1937] -> w1861
              tunnel: [w1878 w1945] -> w1860
              tunnel: [w1877 0] -> w1859
              tunnel: w1858 -> [w1876 _]
              tunnel: w1856 -> [w1875 w1929]
              tunnel: w1855 -> [w1874 w1932]
              tunnel: w1854 -> [w1873 w1934]
              tunnel: w1850 -> [_ w1944]
              tunnel: w1849 -> [_ w1943]
              tunnel: w1848 -> [_ w1942]
              tunnel: w1847 -> [_ w1941]
              tunnel: w1841 -> [_ w1940]
              tunnel: w1846 -> [_ w1938]
              tunnel: [TRUE w1935] -> w1843
              tunnel: [w1870 w1933] -> w1845
              tunnel: [w1868 w1931] -> w1842
              tunnel: [0 0] -> w1839
              frame "Track", Default {
                # "Reset"
                # "Tracking Timeout"
                # "Move Delta"
                # "Goal Position"
                # "Tracking Move"
                # "Move Servo"
                # "Only Consider Tracking Angle\n\nIF\n\nImage Locked        == T\nTrack Angle Flag   == T"
                n653 = And(x=w1875, y=w1874) -> (x .and. y?=w1867:bool)
                n654 = case shown="True" w1867 {
                  tunnel: w1883 -> [_ w1891]
                  tunnel: w1882 -> [_ w1908]
                  tunnel: w1881 -> [_ w1905]
                  tunnel: w1880 -> [w1886 w1895]
                  tunnel: [w1886 w1904] -> w1878
                  tunnel: [w1888 w1903] -> w1879
                  tunnel: [w1888 w1902] -> _
                  tunnel: [u16 0 w1901] -> w1877
                  tunnel: w1876 -> [_ w1897]
                  tunnel: w1873 -> [w1885 _]
                  tunnel: [w1884 0] -> w1870
                  frame False {
                    w1888 = FALSE
                    # "Increment timeout"
                    n655 = Increment(x=w1885) -> (x+1=w1884:i32)
                  }
                  frame True {
                    # "******"
                    # "Determine Direction of Move"
                    # "Convert Track Angle to UINT16"
                    # "1024/300"
                    # "Move to Tracking Angle \n\nif delta is greater than move servo threshold\nAND less than max move threshold"
                    n656 = Add(x=w1908, y=w1891) -> (x+y=w1911:sgl)
                    n657 = local read "Last Track Angle - L"() -> (w1890:sgl)
                    n658 = Add(x=w1911, y=sgl 60.0) -> (x+y=w1910:sgl)
                    n659 = Multiply(x=3.413333333333333, y=w1910) -> (x*y=w1889:dbl)
                    n660 = To Word Integer(number=w1895) -> (16bit integer=w1893:i16)
                    n661 = To Unsigned Word Integer(number=w1889) -> (unsigned 16bit integer=w1907:u16)
                    n662 = To Word Integer(number=w1889) -> (16bit integer=w1906:i16)
                    n663 = Subtract(x=w1889, y=w1890) -> ()  [unwired: 1 out]
                    n664 = Subtract(x=w1906, y=w1893) -> (x-y=w1896:i16)
                    n665 = Absolute Value(x=w1896) -> (abs(x)=w1892:i16)
                    n666 = Greater Or Equal?(x=w1892, y=w1905) -> (x >= y?=w1899:bool)
                    n667 = Less Or Equal?(x=w1892, y=w1897) -> (x <= y?=w1898:bool)
                    n668 = And(x=w1899, y=w1898) -> (x .and. y?=w1900:bool)
                    n669 = case shown="True" w1900 {
                      tunnel: w1907 -> [_ w1919]
                      tunnel: [w1914 w1919] -> w1904
                      tunnel: [w1915 w1925] -> w1903
                      tunnel: [w1915 w1925] -> w1902
                      tunnel: w1895 -> [w1914 _]
                      tunnel: w1892 -> [_ w1924]
                      tunnel: [u16 0 w1924] -> w1901
                      tunnel: w1891 -> [_ w1918]
                      frame False {
                        w1915 = FALSE
                        # "Don't Move"
                      }
                      frame True {
                        w1925 = TRUE
                        # "45 DEG MOUNT OFFSET"
                        # "1024/300"
                        # "Current Delta"
                        # "Use new Track Angle"
                        n670 = Divide(x=w1919, y=3.413333333333333) -> (x/y=w1921:dbl)
                        n671 = Negate(x=w1918) -> (-x=w1917:sgl)
                        n672 = Subtract(x=w1921, y=sgl 60.0) -> (x-y=w1923:dbl)
                        n673 = Add(x=w1923, y=w1917) -> (x+y=w1916:dbl)
                        n674 = local write "Last Track Angle - L"(w1916) -> ()
                      }
                    }
                  }
                }
                n675 = local read "Timeout to \nEnable Reactive Predict"() -> (w1871:u16)
                n676 = Less?(x=w1870, y=w1871) -> (x < y?=w1869:bool)
                n677 = case shown="True" w1869 {
                  tunnel: [enum16{"Track", "Reactive Predict", ""}."Reactive Predict" ("Initial Tracking State - Right") enum16{"Track", "Reactive Predict", ""}."Track" ("Initial Tracking State - Right")] -> w1868
                  frame False {
                  }
                  frame True {
                  }
                }
              }
              frame "Reactive Predict" {
                # "Choose New\nTracking State"
                n678 = Or(x=w1929, y=w1932) -> (x .or. y?=w1928:bool)
                n679 = case shown="False" w1928 {
                  tunnel: [w1958 w2010] -> w1945
                  tunnel: w1944 -> [w1957 _]
                  tunnel: w1943 -> [w1956 _]
                  tunnel: w1942 -> [w1955 _]
                  tunnel: w1941 -> [w1954 _]
                  tunnel: w1940 -> [w1953 _]
                  tunnel: w1938 -> [w1952 _]
                  tunnel: [w1951 w2009] -> w1937
                  tunnel: [w1950 w2009] -> w1935
                  tunnel: w1934 -> [w1949 _]
                  tunnel: [w1948 0] -> w1933
                  tunnel: [enum16{"Track", "Reactive Predict", ""}."Reactive Predict" ("Initial Tracking State - Right") enum16{"Track", "Reactive Predict", ""}."Track" ("Initial Tracking State - Right")] -> w1931
                  tunnel: w1939 -> [w1946 w2010]
                  frame False {
                    # "Stay in Reactive State"
                    # "Increment Track Timeout"
                    # "Move Respond Flag"
                    n680 = Increment(x=w1949) -> (x+1=w1948:i32)
                    n681 = case shown="True" w1953 {
                      tunnel: w1957 -> [_ w1973]
                      tunnel: w1956 -> [_ w1972]
                      tunnel: w1955 -> [_ w1971]
                      tunnel: w1954 -> [_ w1970]
                      tunnel: w1952 -> [_ w1967]
                      tunnel: [w1959 w1963] -> w1958
                      tunnel: [w1960 w1962] -> w1951
                      tunnel: [w1960 w1962] -> w1950
                      tunnel: w1946 -> [w1959 w1961]
                      frame False {
                        w1960 = FALSE
                        # "Reset Move Respond = F"
                        # "Move Servo = F"
                      }
                      frame True {
                        w1962 = TRUE
                        # "Position Lock"
                        # "Current Servo\nPosition"
                        # "Reset Move\nRespond = T"
                        # "Move Servo = T"
                        # "Apply Direction \nto Offset (delta sum)"
                        # "Check Last Known Position of Robot"
                        n682 = case shown="True" w1973 {
                          tunnel: w1972 -> [_ w2001]
                          tunnel: w1971 -> [_ w1976]
                          tunnel: w1970 -> [_ w1977]
                          tunnel: [sgl 1.0 ("y") w1975] -> w1969
                          frame False {
                            # "No Position Data Available"
                            # "Default is to move\nSame Direction as other\nServo"
                          }
                          frame True {
                            w1982 = sgl 1.0 ("y")
                            # "Use previous position/orientation to Guess Which Direction to Move Servo"
                            # "Choose Search Direction"
                            # "\"Perpendicular \nThreshold\""
                            # "If Orientation is\n ~Perpendicular -> Start Search\n in Opposite Direction of Other"
                            # "****add 90 until orientation angle is fixed"
                            # "Last Orientation"
                            # "Convert to Rad"
                            # "Avoid Divide by 0"
                            # "-1/m"
                            # "Calculate Normal Line to \nLast Robot Position\nfrom Center Beacon"
                            # "last Position \nCoordinates"
                            n683 = Unbundle(w2001) -> ("X"=w1981:sgl, "Y"=w1980:sgl)
                            n684 = Unbundle(w1977) -> ("X"=w1979:sgl, "Y"=w1978:sgl)
                            n685 = Subtract(x=w1980, y=w1978) -> (x-y=w1997:sgl)
                            n686 = Subtract(x=w1981, y=w1979) -> (x-y=w1995:sgl)
                            n687 = Equal To 0?(x=w1995) -> (x = 0?=w1996:bool)
                            n688 = case shown="False" w1996 {
                              tunnel: w1997 -> [w2004 _]
                              tunnel: w1995 -> [w2003 _]
                              tunnel: [w2002 1000000000000000.0] -> w1994
                              frame False {
                                n689 = Divide(x=w2004, y=w2003) -> (x/y=w2002:sgl)
                              }
                              frame True {
                              }
                            }
                            n690 = Equal To 0?(x=w1994) -> (x = 0?=w1999:bool)
                            n691 = case shown="False" w1999 {
                              tunnel: [w2006 1e-08] -> w1998
                              tunnel: w1994 -> [w2006 _]
                              frame False {
                              }
                              frame True {
                                # "Can't have infinit slope"
                              }
                            }
                            n692 = Divide(x=-1.0, y=w1998) -> (x/y=w1993:dbl)
                            n693 = Inverse Tangent(1:w1993) -> (0:w1991:dbl)
                            n694 = expression code="(x/pi)*180.0" "radians to degrees"(w1991) -> (w1992:dbl)
                            n695 = To Single Precision Float(number=w1992) -> (single precision float=w1989:sgl)
                            n696 = Add(x=w1976, y=sgl 90.0) -> (x+y=w1988:sgl)
                            n697 = Subtract(x=w1989, y=w1988) -> (x-y=w1987:sgl)
                            n698 = Absolute Value(x=w1987) -> (abs(x)=w1986:sgl)
                            n699 = Less Or Equal?(x=w1986, y=sgl 10.0) -> (x <= y?=w1984:bool)
                            n700 = Negate(x=w1982) -> (-x=w1983:sgl)
                            n701 = Select(t=w1983, s=w1984, f=w1982) -> (s? t:f=w1975:sgl)
                          }
                        }
                        n702 = To Word Integer(number=w1969) -> (16bit integer=w1968:i16)
                        n703 = Multiply(x=w1968, y=w1967) -> (x*y=w1966:i32)
                        n704 = To Word Integer(number=w1961) -> (16bit integer=w1965:i16)
                        n705 = Add(x=w1966, y=w1965) -> (x+y=w1964:i32)
                        n706 = To Unsigned Word Integer(number=w1964) -> (unsigned 16bit integer=w1963:u16)
                      }
                    }
                  }
                  frame True {
                    w2009 = TRUE
                    # "Go Directly to Track State"
                  }
                }
              }
            }
            n707 = local read "Tracking Timeout\nThreshold"() -> (w1852:i32)
            n708 = Less?(x=w1845, y=w1852) -> (x < y?=w1853:bool)
            n709 = case shown="False" w1853 {
              tunnel: [T2."Recovery Mode" ("Next Main State") T2."Tracking" ("Next Main State")] -> w1857
              frame False {
              }
              frame True {
              }
            }
          }
          frame "Recovery Mode" {
            w2020 = u16 0
            # "***Compltetly resets as of R17, used to just reset to \"Max Recovery Count - 1\""
            # "Increment Recoveyr Mode Count"
            # "Frames Processed"
            # "Choose Next Main State"
            # "Reset recovery count"
            # "Recovery move\nCount"
            # "Recovery Search\nAttempt count"
            # "Move Servo = T"
            # "delta move sum"
            # "Robot Position Valid"
            n710 = local read "Image Lock - Right"() -> (w2024:bool)
            n711 = case shown="\"Recovery Search\"" w2017 {
              tunnel: w2046 -> [_ _]
              tunnel: w2045 -> [_ _]
              tunnel: w2044 -> [_ _]
              tunnel: w2043 -> [_ _]
              tunnel: w2042 -> [_ _]
              tunnel: w2041 -> [_ _]
              tunnel: w2040 -> [w2074 w2162]
              tunnel: [w2066 w2160] -> w2039
              tunnel: [w2063 w2154] -> w2038
              tunnel: [FALSE FALSE] -> w2018
              tunnel: [w2068 w2151] -> w2037
              tunnel: w2034 -> [w2072 _]
              tunnel: w2036 -> [w2075 _]
              tunnel: w2035 -> [w2073 w2157]
              tunnel: [w2065 w2150] -> w2032
              tunnel: [w2064 w2150] -> w2033
              tunnel: w2024 -> [w2062 _]
              tunnel: [w2053 w2161] -> w2031
              tunnel: w2030 -> [w2051 w2145]
              tunnel: w2029 -> [w2056 w2158]
              tunnel: w2028 -> [w2052 w2156]
              tunnel: w2014 -> [_ _]
              tunnel: w2016 -> [_ w2153]
              tunnel: [FALSE w2152] -> w2026
              tunnel: w2023 -> [w2060 _]
              tunnel: w2022 -> [w2059 _]
              tunnel: [w2056 w2149] -> w2021
              frame "Recovery Search" {
                # "Wait for 2 Images to be Processed\nBefore Going to Next Step"
                # "Choose Next Reovery State"
                # "Recovery Search \nAttempt Count"
                # "Move Servo"
                # "Goal Position"
                # "Recovery Search\nmove Count"
                # "Attempt Recovery Search if Other Servo has Valid Angle"
                n712 = local read "Last Track Angle - R"() -> (w2055:sgl)
                n713 = Greater Or Equal?(x=w2051, y=w2052) -> (x >= y?=w2054:bool)
                n714 = case shown="True" w2054 {
                  tunnel: w2075 -> [_ w2095]
                  tunnel: [w2080 w2094] -> w2064
                  tunnel: w2074 -> [w2083 w2093]
                  tunnel: w2073 -> [_ w2092]
                  tunnel: [w2081 w2091] -> w2065
                  tunnel: [w2083 w2090] -> w2066
                  tunnel: [FALSE w2089] -> w2063
                  tunnel: w2060 -> [w2081 w2088]
                  tunnel: w2059 -> [w2080 w2087]
                  tunnel: w2062 -> [_ w2086]
                  tunnel: w2055 -> [_ w2085]
                  tunnel: [w2078 0 ("Frames Processed\nCount - in")] -> w2053
                  tunnel: w2051 -> [w2079 _]
                  frame False {
                    # "Increment Frames Processed"
                    # "WAIT"
                    n715 = Increment(x=w2079) -> (x+1=w2078:i32)
                  }
                  frame True {
                    n716 = case shown="True" w2086 {
                      tunnel: w2085 -> [_ w2108]
                      tunnel: w2088 -> [w2096 w2104]
                      tunnel: w2095 -> [_ w2109]
                      tunnel: [w2099 w2107] -> w2090
                      tunnel: [w2097 w2106] -> w2094
                      tunnel: w2087 -> [w2097 w2105]
                      tunnel: w2093 -> [w2099 w2103]
                      tunnel: w2092 -> [_ w2102]
                      tunnel: [FALSE TRUE] -> w2089
                      tunnel: [w2096 w2100] -> w2091
                      frame False {
                        # "Don't Move bc Other Servo Doesn't Have Image Lock"
                      }
                      frame True {
                        # "Move Servo = T"
                        n717 = Greater Than 0?(x=w2104) -> (x > 0?=w2110:bool)
                        n718 = case shown="False" w2110 {
                          tunnel: w2109 -> [w2119 _]
                          tunnel: w2108 -> [w2114 _]
                          tunnel: [w2111 w2129] -> w2107
                          tunnel: [w2117 w2135] -> w2106
                          tunnel: w2105 -> [w2118 w2135]
                          tunnel: w2104 -> [w2116 w2132]
                          tunnel: [w2115 w2134] -> w2100
                          tunnel: w2103 -> [_ w2130]
                          tunnel: w2102 -> [_ w2127]
                          frame False {
                            # "************************"
                            # "Increment move count to transition\nto Pan mode"
                            # "Increment Recovery Search Attempt Count"
                            # "1024/300"
                            # "Move Parallel to Other Servo"
                            n719 = Increment(x=w2118) -> (x+1=w2117:i32)
                            n720 = Add(x=w2114, y=w2119) -> (x+y=w2125:sgl)
                            n721 = Add(x=w2125, y=sgl 60.0) -> (x+y=w2124:sgl)
                            n722 = Multiply(x=3.413333333333333, y=w2124) -> (x*y=w2122:dbl)
                            n723 = Add(x=0.5, y=w2122) -> (x+y=w2120:dbl)
                            n724 = To Unsigned Word Integer(number=w2120) -> (unsigned 16bit integer=w2112:u16)
                            n725 = Add(x=w2112, y=u16 200) -> (x+y=w2111:u16)
                            n726 = Increment(x=w2116) -> (x+1=w2115:i32)
                          }
                          frame True {
                            # "Apply Direction"
                            # "Step SIze"
                            # "Current Position"
                            # "Attempt to Pan in Steps Towards other Servo"
                            # "Could be same or function of \nregular search step size"
                            # "Max # of Pan\nMoves"
                            # "Pan Towards Other Servo"
                            n727 = Greater Or Equal?(x=w2132, y=u16 20) -> (x >= y?=w2133:bool)
                            n728 = case shown="False" w2133 {
                              tunnel: w2132 -> [w2143 _]
                              tunnel: [w2142 u16 0] -> w2134
                              frame False {
                                # "Increment Pan Count"
                                n729 = Increment(x=w2143) -> (x+1=w2142:i32)
                              }
                              frame True {
                                # "Reset move count"
                              }
                            }
                            n730 = local read "Recovery Search\nDirection - L"() -> (w2128:bool)
                            n731 = case shown="False" w2128 {
                              tunnel: w2130 -> [w2137 w2141]
                              tunnel: w2127 -> [w2138 w2140]
                              tunnel: [w2136 w2139] -> w2129
                              frame False {
                                # "CCW"
                                n732 = Add(x=w2137, y=w2138) -> (x+y=w2136:u16)
                              }
                              frame True {
                                # "CW"
                                n733 = Subtract(x=w2141, y=w2140) -> (x-y=w2139:u16)
                              }
                            }
                          }
                        }
                      }
                    }
                  }
                }
                n734 = local read "Max Recovery Count\n(Recovery Search)"() -> (w2057:u16)
                n735 = local read "Max Recovery\nSearch Attempts"() -> (w2058:u16)
                n736 = Less Or Equal?(x=w2064, y=w2058) -> (x <= y?=w2070:bool)
                n737 = Less Or Equal?(x=w2072, y=w2057) -> (x <= y?=w2071:bool)
                n738 = And(x=w2070, y=w2071) -> (x .and. y?=w2069:bool)
                n739 = case shown="False" w2069 {
                  tunnel: [enum16{"Generic Sweep", "Recovery Search"}."Generic Sweep" enum16{"Generic Sweep", "Recovery Search"}."Recovery Search"] -> w2068
                  frame False {
                  }
                  frame True {
                  }
                }
              }
              frame "Generic Sweep" {
                w2150 = u16 0
                # "Angle Valid?"
                # "Choose Next Recovery State"
                # "Wait for 2 Images to be Processed\nBefore Going to Next Step"
                # "New Goal Position"
                # "Move Servo"
                # "Frames Processed Count"
                n740 = Greater Or Equal?(x=w2145, y=w2156) -> (x >= y?=w2163:bool)
                n741 = case shown="True" w2163 {
                  tunnel: w2162 -> [w2179 w2191]
                  tunnel: w2157 -> [_ w2189]
                  tunnel: w2158 -> [w2178 w2188]
                  tunnel: [w2179 w2185] -> w2160
                  tunnel: [w2177 0] -> w2161
                  tunnel: [FALSE TRUE] -> w2155
                  tunnel: w2145 -> [w2180 _]
                  tunnel: [w2178 w2182] -> w2149
                  frame False {
                    # "Increment Frames Processed"
                    n742 = Increment(x=w2180) -> (x+1=w2177:i32)
                  }
                  frame True {
                    # "Reset Frames\nProcessed Count"
                    # "SWEEP SEARCH - Startup"
                    # "Multiple New Step\nby Step SIze"
                    # "F = CCW\nT = CW"
                    # "Last Direction"
                    # "Min Step"
                    # "add 10 in case\nactual position\nis lower than GP"
                    # "Set New Step #"
                    # "Choose Direction"
                    # "Nearest step"
                    # "Adjust Actual Posiiton\n to pre-determiend steps"
                    # "Move Servo 1 \"Step\" to\nSearch"
                    n743 = Add(x=5, y=w2191) -> (x+y=w2197:i32)
                    n744 = Quotient & Remainder(x=w2197, y=w2189) -> (floor(x/y)=w2195:i32)  [unwired: 1 out]
                    n745 = To Byte Integer(number=w2195) -> (8bit integer=w2186:i8)
                    n746 = Less?(x=w2186, y=1) -> (x < y?=w2192:bool)
                    n747 = case shown="False" w2192 {
                      tunnel: w2186 -> [w2208 w2216]
                      tunnel: [w2210 FALSE] -> w2182
                      tunnel: [w2209 w2216] -> w2194
                      tunnel: w2188 -> [w2207 _]
                      tunnel: w2189 -> [w2205 _]
                      frame False {
                        # "Max Step"
                        # "# of steps\nminus 1"
                        n748 = Divide(x=1024, y=w2205) -> (x/y=w2202:dbl)
                        n749 = To Unsigned Byte Integer(number=w2202) -> (unsigned 8bit integer=w2203:u8)
                        n750 = Greater Or Equal?(x=w2208, y=w2203) -> (x >= y?=w2204:bool)
                        n751 = case shown="True" w2204 {
                          tunnel: [w2211 TRUE] -> w2210
                          tunnel: [w2212 w2213] -> w2209
                          tunnel: w2208 -> [w2212 w2213]
                          tunnel: w2207 -> [w2211 _]
                          frame False {
                            # "No Need to\nChange Direction"
                          }
                          frame True {
                            # "T"
                            # "Move CW"
                          }
                        }
                      }
                      frame True {
                        # "F"
                        # "Move CCW"
                      }
                    }
                    n752 = case shown="True" w2182 {
                      tunnel: w2194 -> [w2199 w2200]
                      tunnel: [w2198 w2201] -> w2190
                      frame False {
                        # "CCW\n+1"
                        n753 = Increment(x=w2199) -> (x+1=w2198:i8)
                      }
                      frame True {
                        # "CW\n-1"
                        n754 = Decrement(x=w2200) -> (x-1=w2201:i8)
                      }
                    }
                    n755 = Multiply(x=w2190, y=w2189) -> (x*y=w2187:u16)
                    n756 = To Unsigned Word Integer(number=w2187) -> (unsigned 16bit integer=w2185:u16)
                  }
                }
                n757 = local read "Track Angle Valid  - Right"() -> (w2148:bool)
                n758 = local read "Image Lock - Right"() -> (w2147:bool)
                n759 = Or(x=w2147, y=w2148) -> (x .or. y?=w2146:bool)
                n760 = case shown="False" w2153 {
                  tunnel: [w2166 w2176] -> w2154
                  tunnel: w2155 -> [w2167 _]
                  tunnel: [w2168 enum16{"Generic Sweep", "Recovery Search"}."Generic Sweep"] -> w2151
                  tunnel: [w2165 w2176] -> w2152
                  tunnel: w2146 -> [w2164 _]
                  frame False {
                    # "Is other servo tracking?"
                    n761 = case shown="True" w2164 {
                      tunnel: [enum16{"Generic Sweep", "Recovery Search"}."Generic Sweep" enum16{"Generic Sweep", "Recovery Search"}."Recovery Search"] -> w2168
                      tunnel: w2167 -> [w2171 _]
                      tunnel: [w2171 FALSE] -> w2166
                      tunnel: [FALSE TRUE] -> w2165
                      frame False {
                        # "Stay in Sweep"
                      }
                      frame True {
                        # "G o to Recovery Search  State"
                      }
                    }
                  }
                  frame True {
                    w2176 = FALSE
                    # "Override Move Servo\nCommand bc an Angle Was Found\nduring this Step"
                    # "Stay In Sweep\nLet Main State Machine transition\ninto Tracking"
                  }
                }
              }
            }
            n762 = Increment(x=w2034) -> (x+1=w2015:i32)
            n763 = case shown="True" w2026 {
              tunnel: w2015 -> [w2049 _]
              tunnel: [w2049 0] -> w2027
              frame False {
              }
              frame True {
              }
            }
            n764 = case shown="True" w2014 {
              tunnel: [T2."Recovery Mode" ("Next Main State") T2."Tracking" ("Next Main State")] -> w2025
              frame False {
              }
              frame True {
              }
            }
          }
        }
        "Current Move Delta - L" <- w1742
        n765 = Less?(x=w1769, y=w1768) -> (x < y?=w1767:bool)
        n766 = local write "New Data  Flag\nLeft Servo"(FALSE) -> ()
        n767 = Select(t=w1768, s=w1767, f=w1769) -> (s? t:f=w1764:u16)
        n768 = Greater?(x=w1764, y=w1765) -> (0:w1766:bool)
        n769 = Select(t=w1765, s=w1766, f=w1764) -> (s? t:f=w1763:u16)
      }
    }
    "Next Main State - Left" <- w1173
    "Next Tracking State - Left" <- w1156
    "Next Recovery State - Left" <- w1154
    n770 = flat-sequence {
      tunnel: w1199 -> [w2223]
      tunnel: w1126 -> [w2222]
      tunnel: w1200 -> [w2225]
      tunnel: w1115 -> [w2224]
      tunnel: [w2223] -> w1213
      tunnel: [w2222] -> w1212
      tunnel: w1213 -> [w2231]
      tunnel: [w2230] -> w1208
      tunnel: [w2229] -> w1209
      tunnel: w1212 -> [w2228]
      frame #0 {
        # "Only Update GP if Moving Servo"
        n771 = case shown="True" w2223 {
          tunnel: w2225 -> [_ w2227]
          frame False {
          }
          frame True {
            # "Update Goal Position"
            n772 = local write "Servo Goal Position\n - Left"(w2227) -> ()
          }
        }
        n773 = case shown="True" w2222 {
          tunnel: w2224 -> [_ w2226]
          frame False {
          }
          frame True {
            # "New Direction"
            # "Update Goal Position"
            # "Update Direction"
            n774 = local write "Servo Goal Position\n - Right"(w2226) -> ()
          }
        }
      }
      frame #1 {
        # "Allow Comm Process to Take Down the Flag\nOnly Raise if not already in motion"
        n775 = local read "Servo Moving - R"() -> (w2236:bool)
        n776 = local read "Servo Moving - L"() -> (w2233:bool)
        n777 = local read "Move Servo - L"() -> (w2232:bool)
        n778 = local read "Move Servo - R"() -> (w2239:bool)
        n779 = Not(x=w2236) -> (.not. x?=w2238:bool)
        n780 = Not(x=w2233) -> (.not. x?=w2235:bool)
        n781 = And(x=w2228, y=w2238) -> (x .and. y?=w2237:bool)
        n782 = And(x=w2231, y=w2235) -> (x .and. y?=w2234:bool)
        n783 = case shown="True" w2237 {
          selector: w2237 -> [_ w2241]
          tunnel: [w2240 w2241] -> w2229
          tunnel: w2239 -> [w2240 _]
          frame False {
          }
          frame True {
          }
        }
        n784 = case shown="False" w2234 {
          selector: w2234 -> [_ w2243]
          tunnel: [w2242 w2243] -> w2230
          tunnel: w2232 -> [w2242 _]
          frame False {
          }
          frame True {
          }
        }
        n785 = local write "Move Servo - R"(w2229) -> ()
        n786 = local write "Move Servo - L"(w2230) -> ()
      }
    }
    n787 = local read "Current Main State - Right"() -> (w1178:T2)
    n788 = local read "Current Main State - Left"() -> (w1179:T2)
    n789 = Equal?(x=w1179, y=w1177) -> (x = y?=w1176:bool)
    n790 = Equal?(x=w1178, y=w1177) -> (x = y?=w1175:bool)
    n791 = And(x=w1176, y=w1208) -> (x .and. y?=w1204:bool)
    n792 = And(x=w1209, y=w1175) -> (x .and. y?=w1205:bool)
    n793 = And(x=w1176, y=w1175) -> (x .and. y?=w1203:bool)
    n794 = Exclusive Or(1:w1205, 2:w1204) -> (0:w1202:bool)
    n795 = case shown="True" w1202 {
      tunnel: [w2254 w2275] -> w1210
      tunnel: [w2255 w2274] -> w1206
      tunnel: w1125 -> [_ w2278]
      tunnel: w1166 -> [w2252 w2279]
      tunnel: w1129 -> [w2250 w2277]
      tunnel: [w2253 w2265] -> w1207
      tunnel: [w2251 w2264] -> w1211
      tunnel: w1174 -> [_ w2276]
      tunnel: w1203 -> [w2249 _]
      tunnel: w1204 -> [_ w2275]
      tunnel: w1205 -> [_ w2274]
      frame False {
        n796 = case shown="False" w2249 {
          tunnel: [w2259 w2261] -> w2255
          tunnel: [w2258 w2261] -> w2254
          tunnel: [w2257 w2260] -> w2253
          tunnel: w2252 -> [w2257 _]
          tunnel: [w2256 w2260] -> w2251
          tunnel: w2250 -> [w2256 _]
          frame False {
            # "No Movement\nRetain All Values"
            n797 = local read "Move Respond - L"() -> (w2259:bool)
            n798 = local read "Move Respond - R"() -> (w2258:bool)
          }
          frame True {
            w2260 = i16 0
            w2261 = FALSE
            # "Reset Delta Move sum\nfor both"
            # "F"
            # "Both Moved,\nMake Flags False"
          }
        }
      }
      frame True {
        w2271 = 200 ("y")
        w2262 = -200 ("y")
        # "Add/Clear Sum for \nServo That didn't move"
        # "Update Moving Servo's  Delta Position"
        # "if one Servo Moves, other should \nmove too eventually,\nUsed in Search Process"
        # "Only 1 Servo is Moving Due to Tracking --> Update delta move sum"
        n799 = case shown="True" w2274 {
          tunnel: w2279 -> [_ w2287]
          tunnel: w2278 -> [_ w2286]
          tunnel: [i16 0 w2285] -> w2272
          frame False {
          }
          frame True {
            n800 = Add(x=w2287, y=w2286) -> (x+y=w2285:i32)
          }
        }
        n801 = case shown="True" w2275 {
          tunnel: w2277 -> [_ w2283]
          tunnel: w2276 -> [_ w2282]
          tunnel: [i16 0 w2281] -> w2269
          frame False {
          }
          frame True {
            n802 = Add(x=w2283, y=w2282) -> (x+y=w2281:i32)
          }
        }
        n803 = Greater?(x=w2272, y=w2271) -> (0:w2273:bool)
        n804 = Greater?(x=w2269, y=w2271) -> (0:w2270:bool)
        n805 = Select(t=w2271, s=w2270, f=w2269) -> (s? t:f=w2266:i32)
        n806 = Select(t=w2271, s=w2273, f=w2272) -> (s? t:f=w2267:i32)
        n807 = Greater?(x=w2267, y=w2262) -> (0:w2263:bool)
        n808 = Greater?(x=w2266, y=w2262) -> (0:w2268:bool)
        n809 = Select(t=w2266, s=w2268, f=w2262) -> (s? t:f=w2264:i32)
        n810 = Select(t=w2267, s=w2263, f=w2262) -> (s? t:f=w2265:i32)
      }
    }
    n811 = case shown="True" w1121 {
      selector: w1121 -> [_ w2221]
      tunnel: [w2218 w2220] -> w1161
      tunnel: [w2217 i16 0] -> w1162
      tunnel: w1210 -> [w2218 _]
      tunnel: w1211 -> [w2217 _]
      frame False {
      }
      frame True {
        n812 = Not(x=w2221) -> (.not. x?=w2220:bool)
      }
    }
    "Move Respond - R" <- w1161
    "deltaMoveServo\n- R" <- w1162
    n813 = case shown="False" w1172 {
      selector: w1172 -> [_ w2248]
      tunnel: [w2245 w2247] -> w1164
      tunnel: [w2244 i16 0] -> w1167
      tunnel: w1206 -> [w2245 _]
      tunnel: w1207 -> [w2244 _]
      frame False {
      }
      frame True {
        n814 = Not(x=w2248) -> (.not. x?=w2247:bool)
      }
    }
    "Move Respond - L" <- w1164
    "deltaMoveServo\n- L" <- w1167
    "Current Main State - Left" <- w1198
    "Frames Processed\nCount - in -L" <- w1190
    "Recovery Mode Count - in Left" <- w1185
    "Recovery Search\nmove Count - in - L" <- w1184
    "Recovery Search\nAttempt Count - in - L" <- w1183
    "Current Main State - Right" <- w1152
    "Frames Processed\nCount - in Right" <- w1135
    "Recovery Search\nmove Count - Right" <- w1137
    "Recovery Search\nAttempt Count - Right" <- w1136
    "Recovery Mode Count in Right" <- w1128
    "Tracking Timeout\nCount - L" <- w1159
    "Tracking Timeout\nCount - R" <- w1144
    "Current Tracking State - Left" <- w1158
    "Current Tracking State - Right 2" <- w1150
    "Current Recovery State - Right" <- w1151
    "Current Recovery State -L" <- w1155
  }
